vi "Process.vi"(8 "error in":errorcluster, 11 "Lockin.UI":refnum<class "Instrument UI.Lockin.lvclass">) -> (0 "error out":errorcluster, 3 "Lockin.UI out":refnum<class "Instrument UI.Lockin.lvclass">)   [LabVIEW 2019, in "Instrument.Lockin.lvlib" / "Instrument UI.Lockin.lvclass"]
doc: "---------------------------------------------------------------\nJKI State Machine Objects™\nhttp://jki.net/state-machine-objects/\nCopyright (C) 2005-2015, JKI <info@jki.net>\nALL RIGHTS RESERVEDJKI State Machine Objects (SMO) 1.0.0.5\nJKI - JKI\nCopyright (c) 2016, JKI"
uses:
  Instrument UI.Lockin.lvclass
  Instrument.DAQ/Typedefs/DAQ.Calibration--Cluster--Array.ctl
  Instrument.DAQ/Typedefs/DAQ.Calibration--Cluster.ctl
  Instrument.DAQ/Typedefs/Sweep.Channel--Cluster--Array.ctl
  Instrument.DAQ/Typedefs/Sweep.Channel--Cluster.ctl
  Instrument.DAQ/Typedefs/Sweep.Pattern--Enum.ctl
  Instrument.DAQ/Typedefs/Channel.Gain--Cluster--Array.ctl
  Instrument.DAQ/Typedefs/Channel.Gain--Cluster.ctl
  Instrument.Lockin/Typedefs/Results Type--Enum.ctl
  Instrument.DAQ/Typedefs/DAQ.Configuration--Cluster--Array.ctl
  Instrument.DAQ/Typedefs/DAQ.Configuration--Cluster.ctl
  Instrument.DAQ/Typedefs/DAQ.Config.AO.Range--enum.ctl
  Instrument.DAQ/Typedefs/DAQ.TerminalConfiguration--ring.ctl
  Instrument.DAQ/Typedefs/DAQ.Config.AI.Range--enum.ctl
  Instrument.DAQ/Typedefs/DAQ.Config.AI.Coupling--enum.ctl
  Instrument.DAQ/Typedefs/Simulation Mode--enum.ctl
  Instrument.DAQ/Typedefs/DAQ.Sampling.Fs Mode--enum.ctl
  Instrument.DAQ/Typedefs/AO.Channel--Cluster--Array.ctl
  Instrument.DAQ/Typedefs/AO.Channel--Cluster.ctl
  Instrument.DAQ/Typedefs/AO.Channel.Function--Enum.ctl
  Instrument.DAQ/Typedefs/AI.Channel--Cluster--Array.ctl
  Instrument.DAQ/Typedefs/AI.Channel--Cluster.ctl
  Instrument.DAQ/Typedefs/REF.Channel--Cluster--Array.ctl
  Instrument.DAQ/Typedefs/REF.Channel--Cluster.ctl
  Typedefs/Display-Enum.ctl
  C:/Program Files/National Instruments/LabVIEW 2019/vi.lib/JKI/JKI SMO/SMO/SMO.lvclass
  C:/Program Files/National Instruments/LabVIEW 2019/user.lib/LevyLab/Instrument Framework/Instrument UI/Instrument UI.lvclass
  C:/Program Files/National Instruments/LabVIEW 2019/vi.lib/JKI/JKI SMO/SMO.UI/SMO.UI.lvclass
  Instrument.DAQ/Typedefs/DAQ.Sampling.Sample Mode--Ring.ctl
  Instrument.DAQ/Typedefs/State--enum.ctl
  Instrument.Lockin/Typedefs/API/Lockin.setSweep_Table--cluster.ctl
  Instrument.Lockin/Typedefs/Offset Mode--Enum.ctl
  Instrument.DAQ/Typedefs/PrivateEvents--DAQ.setCalibration.ctl
  Instrument.DAQ/Typedefs/Status--enum.ctl
  <userlib>/LevyLab/Instrument Framework/Instrument UI/Instrument UI.lvclass/Instrument UI.ctl
  Instrument.Lockin/Instrument.Lockin.lvclass
  C:/Program Files/National Instruments/LabVIEW 2019/user.lib/LevyLab/Instrument Framework/Instrument/Instrument.lvclass
  Typedefs/UI.Configuration--Cluster.ctl
  Instrument.DAQ/Typedefs/Configuration.Channels--Cluster.ctl
  Instrument.DAQ/Typedefs/DAQ.Sampling--Cluster.ctl
  Instrument.DAQ/Typedefs/DAQ.Sampling.Sampling--Cluster.ctl
  Instrument.DAQ/Typedefs/Configuration.Prefilter--Cluster.ctl
  Instrument.DAQ/Typedefs/Channel.GainsAndOffsets--Cluster.ctl
  Instrument.DAQ/Typedefs/Configuration.AmplitudeLimit--Cluster.ctl
  Instrument.DAQ/Typedefs/Configuration.DCLimit--Cluster.ctl
  Instrument.DAQ/Typedefs/Configuration.LinkFrequencies--Cluster.ctl
  Instrument.DAQ/Typedefs/Sweep.Configuration--Cluster.ctl
  Instrument.DAQ/Typedefs/Configuration.DutyCycle--Cluster.ctl
  Instrument.Lockin/Typedefs/Lockin.getAllData--Cluster.ctl
  Instrument.DAQ/Typedefs/PublicEvents--DAQ.getWaveforms.ctl
  Instrument.DAQ/Typedefs/Results--Cluster.ctl
  Instrument.DAQ/Typedefs/PublicEvents--DAQ.getSweepWaveforms.ctl
  <userlib>/LevyLab/Configuration/Configuration.lvclass
  Typedefs/UI.References--Cluster.ctl
  Typedefs/UI.References.Booleans--Cluster.ctl
  Typedefs/UI.References.Clusters--Cluster.ctl
  Typedefs/UI.References.Graphs--Cluster.ctl
  <userlib>/LevyLab/Configuration/Configuration.lvclass/Configuration.ctl
  <vilib>/JKI/JKI SMO/SMO/SMO.lvclass/SMO.ctl
  <vilib>/JKI/JKI SMO/SMO.UI/SMO.UI.lvclass/SMO.UI.ctl
  Instrument.Lockin/Typedefs/API/Lockin.setState--cluster.ctl
  Instrument.Lockin/Typedefs/API/Lockin.Commands--Enum.ctl
  Instrument.Lockin/Typedefs/API/Lockin.Commands.Local--Enum.ctl
  Instrument.DAQ/Typedefs/PrivateEvents--DAQ.showUI.ctl
  Instrument.Lockin/Typedefs/API/Lockin.setLogMode--cluster.ctl
  Instrument.Lockin/Typedefs/API/Lockin.setSamplingMode--cluster.ctl
  Instrument.Lockin/Typedefs/API/Lockin.setSamplingFsMode--cluster.ctl
  fb76c5f8-a1bb-4bb3-bb88-03f40c6ef356.vi
  76a2c689-62cf-4547-b40d-909294413a54.vi
  ea889f97-4432-4e18-8daa-f8276c71e6b3.vi
  e313e854-8cc0-44b2-b8a5-b0d9dd449797.vi
  f60e4b8a-05f4-439c-aeb3-da82266228cf.vi
  5a499ed1-b987-4b60-a17a-49cbc4aa87e6.vi
  11ce9ad4-6d29-4ca4-b8bb-b11228104e6f.vi
  a8738246-2ac0-499e-83b1-af72f8904bf5.vi
  <vilib>/JKI/JKI SMO/SMO/Private/ReftoDVR--SMO.vi
  <vilib>/JKI/JKI SMO/SMO.UI/SMO.UI.ReftoDVR.vi
  11ce9ad4-6d29-4ca4-b8bb-b11228104e6f.vi/189031a7-82a1-4f0a-9ed5-d68f3439fd4c.vi
  11ce9ad4-6d29-4ca4-b8bb-b11228104e6f.vi/de7eedf1-e1e8-4423-8aaa-e1093bc59ae0.vi
  <userlib>/LevyLab/Debug/Debug/Get Debug Mode.vi
  <vilib>/Platform/browser.llb/Open URL in Default Browser (string).vi
  private/Set Plot Visibility (WDTWFGraph).vi
  <vilib>/measure/matone.llb/Extract Single Tone Information 1 Chan.vi
  private/Set Plot Color (WFChart2D).vi
  private/Set Legend (WDTWFGraph).vi
  <vilib>/Waveform/WDTOps.llb/WDT Waveform Duration DBL.vi
  <vilib>/Utility/Data Type/Get Type Information.vi
  <vilib>/Utility/Data Type/Get Numeric Information.vi
  <userlib>/_OpenG.lib/lvdata/lvdata.llb/Unwrap VVariant__ogtk.vi
  <vilib>/JDP Science/JSONtext/Variant to JSON Text.vi
  <userlib>/LevyLab/Instrument Framework/Instrument/API/Instrument.sendMessageToProcess (string).vi
  <vilib>/JKI/JKI SMO/SMO/SMO.lvclass
  <userlib>/LevyLab/Instrument Framework/Instrument/Instrument.lvclass
  <vilib>/JDP Science/JSONtext/LVClass Serializer/JSONtext LVClass Serializer.lvclass
  <userlib>/LevyLab/Instrument Framework/Instrument UI/Instrument UI.lvclass
  Instrument.DAQ/Instrument.DAQ.lvclass
  <vilib>/measure/NI_MAPro.lvlib
  <vilib>/JKI/JKI SMO/SMO.UI/SMO.UI.lvclass
  Lockin.Utilities/Lockin.Utilities.lvlib
  <userlib>/LevyLab/Debug/Debug.lvlib
  C:/Program Files/National Instruments/LabVIEW 2019/user.lib/LevyLab/Instrument Framework/Instrument Types/Lockin/Instrument.LockinAPI.lvclass
  private/Set All Plot Visibility (WFGraph).vi
  private/Set All Plot Visibility (XYGraph).vi
  private/Get Plot Visibility (WFGraph).vi
  private/Set Plot Visibility (WFGraph).vi
  private/Set Plot Visibility (XYGraph).vi
  private/Set Legend (WFGraph).vi
  private/Set Plot Color (WDTWFGraph).vi
  private/Set Plot Color (WFGraph).vi
  private/Set Legend (XYGraph).vi
  private/Set Plot Color (XYGraph).vi
  <vilib>/measure/maspectr.llb/FFT Power Spectrum and PSD for N Chan.vi
panel:
  out "Version":string="vDevelopment" caption="V"
  in  "Fs Multiplier":dbl=5000.0 format="%#_13g"
  in  "Refresh Rate (Hz)":dbl=10.0 format="%#_13g"
  in  "Decimate":enum16{"1", "10", "100", "1000"}(ring) caption="Enum 3"
  in  "Decimation (pre DSP)":i32=1
  in  "Decimation (post DSP)":i32=1
  in  "....................State....................":bool
  in  "....................Graph and UI....................":bool
  in  "....................DAQ and Channel....................":bool
  in  "....................Dynamic Events....................":bool
  in  "Left Tab":T1(tab)=enum."DAQ Settings"
  in  "f link (Hz)":dbl=13.0 format="%#_6p"
  in  "Link f?":bool
  in  "DC Limit All":bool
  in  "DC Limit None":bool
  in  "AC Limit All":bool
  in  "AC Limit None":bool
  out "-3dB BW (Hz)":dbl=50.0
  out "Noise BW (Hz)":dbl=50.0
  out "Settling Time (s)":dbl=50.0
  in  "REF Channels":T2 {"Roll-Off" min=1 max=4; "TC" min=1e-06 max=100.0 format="%#_3p"; "Phase" format="%#_3p"; "Frequency" min=1e-06 max=102400.0 format="%#_6p"; "Channel" min=1}
  in  "AO DC Limit":dbl=0.009999999 caption="DC limit" format="%#_6p"
  in  "AC Limit":dbl=0.009999999 caption="AC limit" format="%#_6p"
  in  "duty cycle (%)":dbl=50.0
  in  "Disable All":bool
  in  "Enable All":bool
  in  "AI Channels":T4 {"reference index" min=1; "References" items=["", "1", "2", "3", "4", "5", "6", "7", "8", "9"]; "Channel" min=1}
  in  "AO Channels":T6 {"Phase" format="%#_3g"; "Frequency" min=0.0001 max=200000.0 format="%#_6p"; "Offset" format="%#_6p"; "Amplitude" min=0.0 max=10.0 format="%#_6p"}
  out "Fs Output (S/s)":dbl=100.0
  in  "Remove Offset":bool
  in  "Measure Offset":bool
  in  "Fs (S/s) (buffer)":dbl=204800.0 format="%#_13g"
  in  "#s (S) (buffer)":i32=20480
  in  "Show DAQ UI":bool
  out "Actual Fs (S/s)":dbl=10.0 format="%#_13g"
  out "Actual #s (S)":i32=10
  in  "DAQ Config":T9 {"AI terminal config" items=[""=-1, "differential"=10106, "pseudodifferential"=12529]; "AI.Coupling" items=[""=0, "AC"=10045, "DC"=10050, "GND"=10066]; "AO terminal config" items=[""=-1, "differential"=10106, "pseudodifferential"=12529]}
  in  "Auto DAQ":bool caption="Auto Configure"
  in  "Fs Mode":T15
  in  "Logging":bool
  in  "AI Simulation mode":T16=enum."AI = noise*AO"
  in  "Reset Phase":bool
  in  "LP f (Hz)":dbl=100.0 format="%.3p"
  in  "Line":bool
  in  "Lowpass":bool
  in  "PLL AI Channel":i32=1 caption="AI Channel"
  in  "Enable PLL":bool caption="Enable"
  in  "Input Gain":T17
  in  "Output Gain":T17
  in  "Input Offsets":T17 {"Gain" format="%#_3p"}
  in  "Route Signal Type":T19 caption="Signal Type"
  in  "Route Ref Channel":i32=1 caption="Ref Channel"
  in  "Route AI Channel":i32=1 caption="AI Channel"
  out "Route Output (V)":dbl caption="Output (V)"
  in  "Route AO Channel":i32=1 caption="AO Channel" min=1
  in  "Enable Route":bool caption="Enable"
  in  "Sweep Pattern":cluster{"Channel":u16, "Sweep Pattern":dbl[]}[](array[cluster])=[{"Channel"=0, "Sweep Pattern"=[]}] {"Sweep Pattern" format="%#_3p"; "Channel" min=1 max=128}
  in  "Sweep Channels":T20=[{"Enable?"=FALSE, "Channel"=0, "Start"=0.0, "End"=0.1, "Pattern"=enum."Table", "Table"=[]}] {"Table" format="%#_1f"; "Channel" min=1 max=128; "Start" format="%#_6p"; "End" format="%#_6p"}
  in  "Sweep Time (s)":dbl=20.0
  in  "Initial Wait (s)":dbl=1.0
  out "Sweep Timer (s)":dbl caption="Timer (s)"
  in  "Return to Start?":bool
  out "System Serial Number":string caption="SMO State"
  out "Application Version":string caption="SMO State"
  out "Status":string
  out "Sampling Status":u32(colorbox)
  out "State Queue":string
  out "Sampling Status":string="Good"
  out "State History":string
  out "Wfm Refresh Time (ms)":u32=103
  out "Inst.DAQ State":string caption="SMO State"
  out "UI Refresh Time (ms)":u32=103
  out "Sweep Time":dbl format="%<%I:%M:%S %p %m/%d/%Y>T"
  out "State Time":dbl format="%<%I:%M:%S %p %m/%d/%Y>T"
  out "Cal Info":T23 {"DevTemp" format="%.1f"; "SelfCal.LastTemp" format="%.1f"; "SelfCal.LastDate/Time" format="%<%I:%M %p %m/%d/%Y>T"}
  in  "Get Calibration":bool
  in  "Self Calibrate":bool
  in  "Tab Control 3":enum32{"Page 1"}(tab)
  out "mean (V)":dbl format="%_3p"
  out "X (V)":dbl format="%_3p"
  out "Y (V)":dbl format="%_3p"
  in  "channel-reference":u16(ring) items=["AI1 REF 1"]
  out "R (V)":dbl format="%_3p"
  out "theta (°)":dbl format="%_3p"
  in  "Close":bool
  out "String":string
  in  "Pause":bool
  in  "Reset":bool
  in  "Start":bool
  in  "Help":bool
  in  "Start Sweep":bool
  in  "Stop Sweep":bool
  in  "Right Tab":T25(tab)
  in  "Sync?":bool
  in  "Sync Ch":i32=1
  out "f (Hz)":string
  out "phi (°)":string
  in  "Output":enum16{"AO", "REF"}(ring) caption="Enum 3"
  in  "Input":enum16{"Device", "ADC"}(ring) caption="Enum 3"
  out "REF Graph":waveform(dbl)[](graph)
  in  "AO Graph All":bool
  in  "AO Graph None":bool
  in  "AI Graph All":bool
  in  "AI Graph None":bool
  out "AI Graph":waveform(dbl)[](graph)
  in  "X Scale":enum16{"time", "samples"}(ring) caption="Enum 3"
  out "AO Graph":waveform(dbl)[](graph)
  in  "REF Graph None":bool
  in  "REF Graph All":bool
  out "Lockin 1":waveform(dbl)[](graph)
  in  "Display 2":T26 caption="Enum 3"
  in  "Y/Theta Range":dbl caption="Range" format="%#_6p"
  in  "Display 1":T26 caption="Enum 3"
  in  "X/R Range":dbl caption="Range" format="%#_6p"
  out "Lockin 2":waveform(dbl)[](graph)
  in  "Lockin Graph All":bool
  in  "Lockin Graph None":bool
  out "Results":string[][](table)
  out "Lockin XY":cluster{dbl[], dbl[]}[](graph)
  in  "XY Range":dbl caption="Range" format="%#_6p"
  in  "Lockin Graph None 2":bool
  in  "Lockin Graph All 2":bool
  out "Sweep AI":waveform(dbl)[](graph)
  out "Sweep AO":waveform(dbl)[](graph)
  out "Sweep Y":waveform(dbl)[](graph)
  out "Sweep X":waveform(dbl)[](graph)
  in  "chart?":bool=TRUE
  in  "chart all?":bool=TRUE
  in  "PS Display":enum16{"AO", "AI", "X", "Y", "R", "Theta"}(ring) caption="Enum 3"
  in  "# averages":u32=10 min=1
  in  "weighting mode":enum16{"Linear", "Exponential"}(ring)=enum."Exponential"
  in  "averaging mode":T27(ring)=enum."RMS averaging"
  in  "window":u32(ring)=1 items=["Rectangle"=0, "Hanning"=1, "Hamming"=2, "Blackman-Harris"=3, "Exact Blackman"=4, "Blackman"=5, "Flat Top"=6, "4 Term B-Harris "=7, "7 Term B-Harris"=8, "Low Sidelobe"=9, "Blackman Nuttall"=11, "Triangle"=30, "Bartlett-Hanning"=31, "Bohman"=32, "Parzen"=33, "Welch"=34, "Kaiser"=60, "Dolph-Chebyshev"=61, "Gaussian"=62]
  in  "export mode":u16(ring)=1 items=["Power Spectrum", "Power Spectral Density"]
  in  "restart":bool
  out "done?":bool=TRUE
  out "PS Waveform":cluster{"f0":dbl, "df":dbl, "magnitude":dbl[]}[](graph)
  out "averages":dbl=180.0
  out "PS Chart":dbl[][](graph)
  # "Lockin UI"
  # "For instructions on how to use the JKI State Machine Objects, examples and video tutorials, visit:\nhttp://jki.net/state-machine-objects/\n\nJKI State Machine Objects™\nhttp://jki.net/state-machine-objects/\nCopyright (C) 2005-2015, JKI <info@jki.net>\nALL RIGHTS RESERVED"
  # "- Choose an input lockin channel and value (X,Y, etc) and it will be written as a DC value to an output channel of your choosing.\n- Output is scaled by the input amplifier gain."
  # "Output"
  # "Input"
  # ">> DEVICE >>"
  # "(*)"
  # "ch"
  # "AC (V)"
  # "DC (V)"
  # "f (Hz)"
  # "phase (°)"
  # "function"
  # "sweep"
  # "(*)"
  # "ch"
  # "1     2    3"
  # "References"
  # "Offset"
  # "Output Settings"
  # "Reference"
  # "Reference Filter"
  # "ch"
  # "f (Hz)"
  # "phase (°)"
  # "TC (s)"
  # "order (n)"
  # "DAQ Channels"
  # "Device"
  # "AO"
  # "AI"
  # "terminals"
  # "ch"
  # "ch"
  # "range"
  # "range"
  # "coupling"
  # "terminals"
  # "Sampling"
  # "Pre-Filters"
  # "Simulation"
  # "Push \"Reset Acquisiton\" below when you want to apply new settings"
  # "not used during process-ing"
  # "DAQ"
  # "Logging"
  # "Output Gain"
  # "Input Offset / Gain"
  # "Route Lockin Input to Output"
  # "PLL"
  # "experimental ca 11/18/2025"
  # "experimental ca 11/18/2025"
  # "ch"
  # "Input gain"
  # "ch"
  # "Output gain"
  # "ch"
  # "Input offset"
  # "Sweep"
  # "pattern"
  # "(*)"
  # "ch"
  # "start"
  # "end"
  # "ch"
  # "table"
  # "Status"
  # "Calibration"
  # "Most Recent Self-Calibration"
  # "device"
  # "time"
  # "T (°C)"
  # "T (°C)"
  # "OK?"
  # "DAQ"
  # "Sweep"
  # "Application"
  # "Status"
  # "Input Graphs"
  # "Output Graphs"
  # "Lockin Results: Graph 1"
  # "Lockin Results: Graph 2"
  # "Lockin Results: Table"
  # "Lockin Results: Phasor Graph"
  # "Sweep AI"
  # "Sweep AO"
  # "Sweep Results"
  # "Sweep Results"
  # "Power Spectra"
  # "db( ):\ndB(V) for volts\ndB(A) for amps\ndB(°) for degrees"
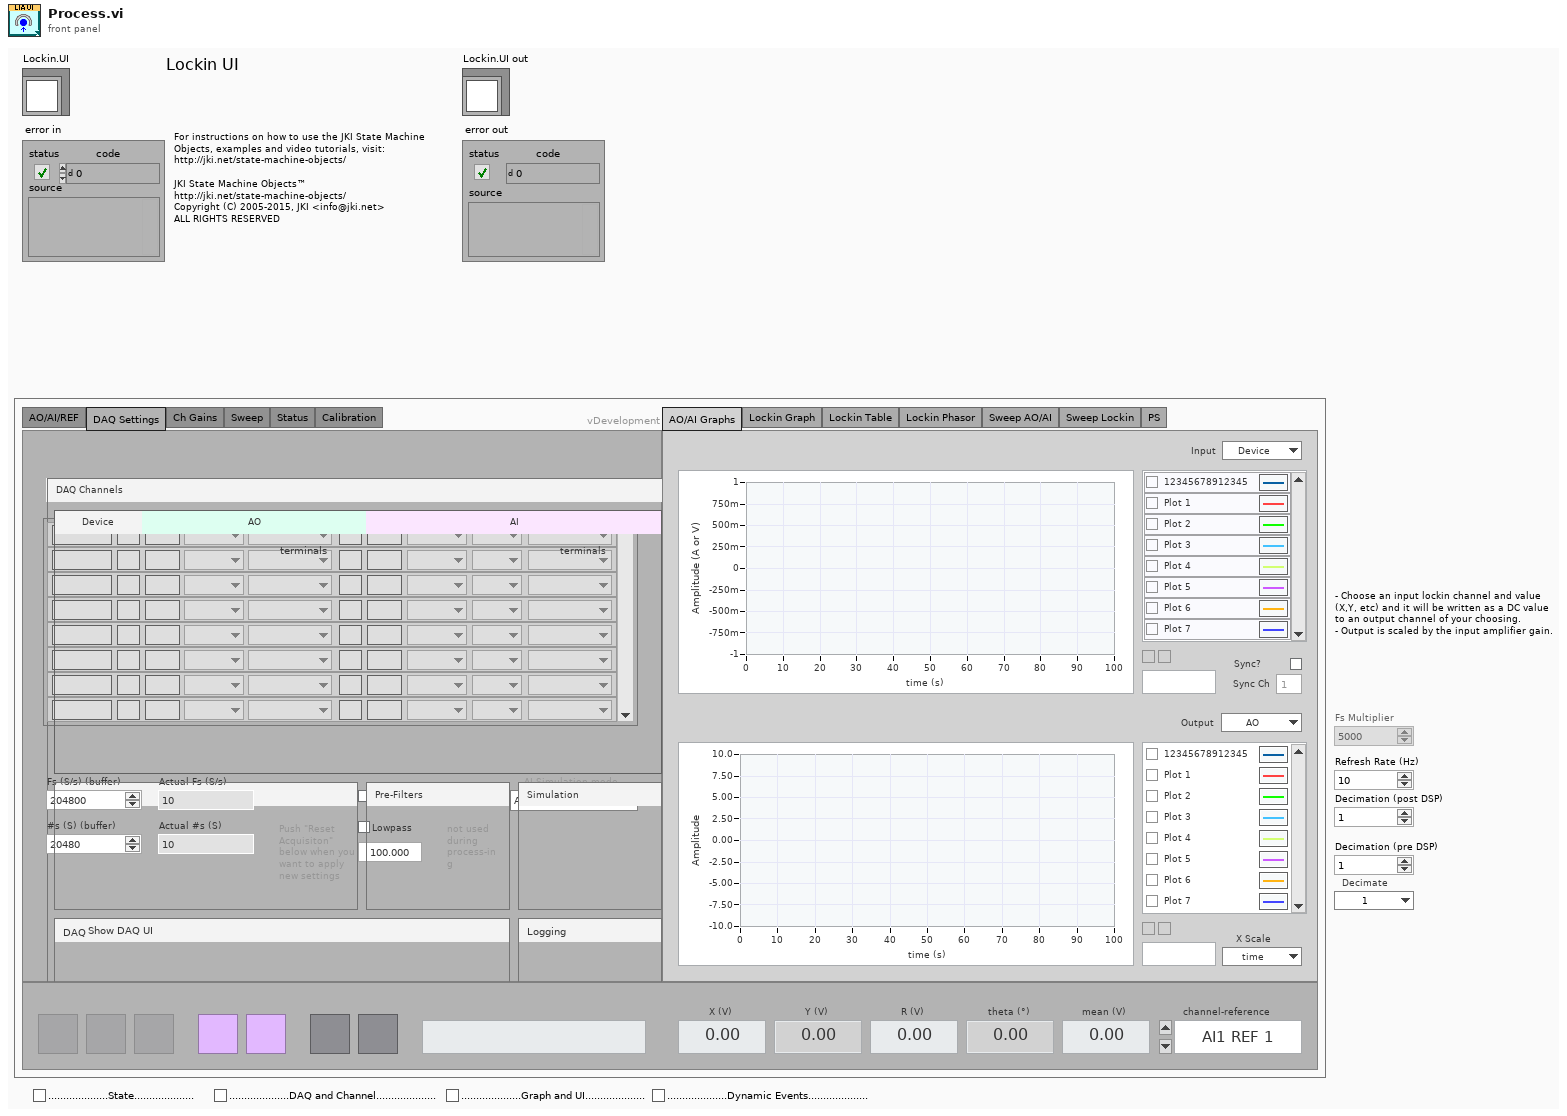
[diagram p1: front panel]
types:
  T1 = enum32{"AO/AI/REF", "DAQ Settings", "Ch Gains", "Sweep", "Status", "Calibration"}
  T2 = typedef "Instrument.Lockin.lvlib/Instrument.DAQ.lvclass/REF.Channel--Cluster--Array.ctl" = T3[]
  T3 = typedef "Instrument.Lockin.lvlib/Instrument.DAQ.lvclass/REF.Channel--Cluster.ctl" = cluster{"Enable?":bool, "Channel":i32, "Frequency":dbl, "Phase":dbl, "TC":dbl, "Roll-Off":i32}
  T4 = typedef "Instrument.Lockin.lvlib/Instrument.DAQ.lvclass/AI.Channel--Cluster--Array.ctl" = T5[]
  T5 = typedef "Instrument.Lockin.lvlib/Instrument.DAQ.lvclass/AI.Channel--Cluster.ctl" = cluster{"Enable?":bool, "Channel":i32, "References":u16[], "reference index":i32}
  T6 = typedef "Instrument.Lockin.lvlib/Instrument.DAQ.lvclass/AO.Channel--Cluster--Array.ctl" = T7[]
  T7 = typedef "Instrument.Lockin.lvlib/Instrument.DAQ.lvclass/AO.Channel--Cluster.ctl" = cluster{"Enable?":bool, "Channel":i32, "Amplitude":dbl, "Offset":dbl, "Frequency":dbl, "Phase":dbl, "Function":T8, "Sweeping?":bool, "Limit AC":bool, "Limit DC?":bool, "Duty Cycle":bool}
  T8 = typedef "Instrument.Lockin.lvlib/Instrument.DAQ.lvclass/AO.Channel.Function--Enum.ctl" = enum16{"sine", "square", "triangle", "saw"}
  T9 = typedef "Instrument.Lockin.lvlib/Instrument.DAQ.lvclass/DAQ.Configuration--Cluster--Array.ctl" = T10[]
  T10 = typedef "Instrument.Lockin.lvlib/Instrument.DAQ.lvclass/DAQ.Configuration--Cluster.ctl" = cluster{"Device":string, "Lockin.AO":string, "AO.Ch":string, "AO.Range":T11, "AO terminal config":T12, "Lockin.AI":string, "AI.Ch":string, "AI.Range":T13, "AI.Coupling":T14, "AI terminal config":T12}
  T11 = typedef "Instrument.Lockin.lvlib/Instrument.DAQ.lvclass/DAQ.Config.AO.Range--enum.ctl" = enum16{"±0.1", "±1.0", "±3.5", "±10.0", ""}
  T12 = typedef "Instrument.Lockin.lvlib/Instrument.DAQ.lvclass/DAQ.TerminalConfiguration--ring.ctl" = i32
  T13 = typedef "Instrument.Lockin.lvlib/Instrument.DAQ.lvclass/DAQ.Config.AI.Range--enum.ctl" = enum16{"±0.316", "±1.00", "±3.16", "±10.0", "±31.6", "±42.4", ""}
  T14 = typedef "Instrument.Lockin.lvlib/Instrument.DAQ.lvclass/DAQ.Config.AI.Coupling--enum.ctl" = u16
  T15 = typedef "Instrument.Lockin.lvlib/Instrument.DAQ.lvclass/DAQ.Sampling.Fs Mode--enum.ctl" = enum16{"Manual", "Auto Fs", "Max Fs"}
  T16 = typedef "Instrument.Lockin.lvlib/Instrument.DAQ.lvclass/Simulation Mode--enum.ctl" = enum16{"AI = HW simulated", "AI = noise*AO", "AI = waveguide"}
  T17 = typedef "Instrument.Lockin.lvlib/Instrument.DAQ.lvclass/Channel.Gain--Cluster--Array.ctl" = T18[]
  T18 = typedef "Instrument.Lockin.lvlib/Instrument.DAQ.lvclass/Channel.Gain--Cluster.ctl" = cluster{"Channel":string, "Gain":dbl}
  T19 = typedef "Instrument.Lockin.lvlib/Instrument.Lockin.lvclass/Results Type--Enum.ctl" = enum16{"X", "Y", "R", "Theta", "Mean"}
  T20 = typedef "Instrument.Lockin.lvlib/Instrument.DAQ.lvclass/Sweep.Channel--Cluster--Array.ctl" = T21[]
  T21 = typedef "Instrument.Lockin.lvlib/Instrument.DAQ.lvclass/Sweep.Channel--Cluster.ctl" = cluster{"Enable?":bool, "Channel":u16, "Start":dbl, "End":dbl, "Pattern":T22, "Table":dbl[]}
  T22 = typedef "Instrument.Lockin.lvlib/Instrument.DAQ.lvclass/Sweep.Pattern--Enum.ctl" = enum16{"Ramp /", "Ramp /\\", "Smooth Ramp _/", "Smooth Ramp _/\\_", "Table"}
  T23 = typedef "Instrument.Lockin.lvlib/Instrument.DAQ.lvclass/DAQ.Calibration--Cluster--Array.ctl" = T24[]
  T24 = typedef "Instrument.Lockin.lvlib/Instrument.DAQ.lvclass/DAQ.Calibration--Cluster.ctl" = cluster{"Active Device":string, "SelfCal.LastDate/Time":dbl, "SelfCal.LastTemp":dbl, "DevTemp":dbl, "calibration due?":bool}
  T25 = enum32{"AO/AI Graphs", "Lockin Graph", "Lockin Table", "Lockin Phasor", "Sweep AO/AI", "Sweep Lockin", "PS"}
  T26 = typedef "Instrument.Lockin.lvlib/Instrument UI.Lockin.lvclass/Display-Enum.ctl" = enum16{"X", "Y", "R", "Theta", "Mean"}
  T27 = enum16{"No averaging", "Vector averaging", "RMS averaging", "Peak hold"}
  T28 = enum16{"Spinner 1", "Spinner 2", "Spinner 3", "Spinner 4", "Spinner 5", "Spinner 6"}
  T29 = typedef "Instrument.Lockin.lvlib/Instrument.DAQ.lvclass/State--enum.ctl" = enum16{"start", "stop", "reset", "start sweep", "stop sweep"}
  T30 = typedef "Instrument.Lockin.lvlib/Instrument.Lockin.lvclass/Lockin.setSweep_Table--cluster.ctl" = cluster{"Channel":i32, "Table":dbl[]}
  T31 = typedef "Instrument.Lockin.lvlib/Instrument.Lockin.lvclass/Offset Mode--Enum.ctl" = enum16{"Measure", "Remove"}
  T32 = typedef "Instrument.Lockin.lvlib/Instrument.DAQ.lvclass/PrivateEvents--DAQ.setCalibration.ctl" = enum16{"Check", "Calibrate"}
  T33 = typedef "Instrument.Lockin.lvlib/Instrument.DAQ.lvclass/Status--enum.ctl" = enum16{"idle", "created", "started", "stopped", "sweeping"}
  T34 = enum32{"invalid app kind", "Development System", "Run Time System", "Student Edition", "Embedded LabVIEW", "Evaluation", "Custom"}
  T35 = enum32{"Invalid", "Standard", "Closed", "Hidden", "Minimized", "Maximized"}
  T36 = enum8{"Enabled", "Disabled", "Disabled and Grayed Out"}
  T37 = typedef "Instrument.Lockin.lvlib/Instrument.Lockin.lvclass/Lockin.setState--cluster.ctl" = cluster{"State":T29}
  T38 = typedef "Instrument.Lockin.lvlib/Instrument.Lockin.lvclass/Lockin.Commands--Enum.ctl" = enum16{"setAO", "setAO_Amplitude", "setAO_DC", "setAO_Frequency", "setAO_Phase", "setAO_Function", "setREF", "setREF_Frequency", "setREF_Phase", "setREF_TC", "setREF_Roll-Off", "setDAQ", "setSampling", "setState", "getState", "getAO", "getAI", "getResults", "getSampling", "getAOconfig", "getREFconfig", "setInputGain", "setOutputGain", "getInputGain", "getOutputGain", "setSamplingFsMode", "getSamplingFsMode", "setSweep", "setSweep_Time", "setSweep_Table", "getStatus", "getSweepResults", "getSweepWaveforms", "logConfiguration", "startLogging", "stopLogging"}
  T39 = typedef "Instrument.Lockin.lvlib/Instrument.Lockin.lvclass/Lockin.Commands.Local--Enum.ctl" = enum16{"autoConfigureDAQ", "setSimulationMode", "zeroPhase", "setCalibration", "setPreFilter", "setFrequencyLink", "setAmplitudeLimit", "setDCLimit", "setDutyCycle", "setSamplingDecimationPreDSP", "setSamplingDecimationPostDSP", "setSamplingMode", "setSamplingFsMultiplier", "setSamplingFsOutput", "setSamplingRefreshRate", "setData_State", "setData_DAQ", "setData_Sampling", "setData_Waveforms", "setData_Results", "setData_SweepWaveforms", "setData_AIChannels", "setData_AOChannels", "setData_REFChannels", "setData_InputGain", "setData_OutputGain", "showUI", "setAI", "setOffset", "setOffsetMode"}
  T40 = typedef "Instrument.Lockin.lvlib/Instrument.DAQ.lvclass/PrivateEvents--DAQ.showUI.ctl" = bool
  T41 = typedef "Instrument.Lockin.lvlib/Instrument.Lockin.lvclass/Lockin.setLogMode--cluster.ctl" = cluster{"interval":u32}
  T42 = typedef "Instrument.Lockin.lvlib/Instrument.Lockin.lvclass/Lockin.setSamplingMode--cluster.ctl" = cluster{"SampleMode":T43}
  T43 = typedef "Instrument.Lockin.lvlib/Instrument.DAQ.lvclass/DAQ.Sampling.Sample Mode--Ring.ctl" = i32
  T44 = typedef "Instrument.Lockin.lvlib/Instrument.Lockin.lvclass/Lockin.setSamplingFsMode--cluster.ctl" = cluster{"FsMode":T15}
  T45 = cluster{"averaging mode":enum16{"No averaging", "Vector averaging", "RMS averaging", "Peak hold"}, "weighting mode":enum16{"Linear", "Exponential"}, "number of averages":u32}
  T46 = typedef "Instrument.Lockin.lvlib/Instrument UI.Lockin.lvclass/UI.Configuration--Cluster.ctl" = cluster{"Channels":T47, "DAQ":cluster{"Configuration":T9, "cfg.Sampling":T48, "Calibration":T23, "Simulation mode":T16}, "PreFilter":T50, "Amplifers":T51, "Limit Amplitude":T52, "Limit DC":T53, "Link Frequencies":T54, "Sweep":T55, "Plot":cluster{"visibility.AI":bool[], "visibility.AO":bool[], "visibility.Lockin":bool[], "Display 1":T26, "Display 2":T26}, "Function Option":T56}
  T47 = typedef "Instrument.Lockin.lvlib/Instrument.DAQ.lvclass/Configuration.Channels--Cluster.ctl" = cluster{"Cfg_AO":T6, "Cfg_AI":T4, "Cfg_REF":T2}
  T48 = typedef "Instrument.Lockin.lvlib/Instrument.DAQ.lvclass/DAQ.Sampling--Cluster.ctl" = cluster{"Sampling":T49, "sample mode":i32, "Fs Mode":T15, "Fs Multiplier":dbl, "Refresh Rate (Hz)":dbl, "Decimation.PreDSP":i32, "Decimation.PostDSP":i32, "Fs.Output":dbl}
  T49 = typedef "Instrument.Lockin.lvlib/Instrument.DAQ.lvclass/DAQ.Sampling.Sampling--Cluster.ctl" = cluster{"Fs":dbl, "#s":i32}
  T50 = typedef "Instrument.Lockin.lvlib/Instrument.DAQ.lvclass/Configuration.Prefilter--Cluster.ctl" = cluster{"60 Hz":bool, "Low Pass":bool, "Low Pass Cutoff (Hz)":dbl}
  T51 = typedef "Instrument.Lockin.lvlib/Instrument.DAQ.lvclass/Channel.GainsAndOffsets--Cluster.ctl" = cluster{"Offset_AI":T17, "Gain_AI":T17, "Gain_AO":T17}
  T52 = typedef "Instrument.Lockin.lvlib/Instrument.DAQ.lvclass/Configuration.AmplitudeLimit--Cluster.ctl" = cluster{"Limit (V)":dbl}
  T53 = typedef "Instrument.Lockin.lvlib/Instrument.DAQ.lvclass/Configuration.DCLimit--Cluster.ctl" = cluster{"Limit (V)":dbl}
  T54 = typedef "Instrument.Lockin.lvlib/Instrument.DAQ.lvclass/Configuration.LinkFrequencies--Cluster.ctl" = cluster{"Link?":bool, "Frequency (Hz)":dbl}
  T55 = typedef "Instrument.Lockin.lvlib/Instrument.DAQ.lvclass/Sweep.Configuration--Cluster.ctl" = cluster{"sweepTime":dbl, "initialWaitTime":dbl, "returnToStart":bool, "sweepChannels":T20}
  T56 = typedef "Instrument.Lockin.lvlib/Instrument.DAQ.lvclass/Configuration.DutyCycle--Cluster.ctl" = cluster{"Option?":bool, "Duty Cycle (%)":dbl}
  T57 = typedef "Instrument.Lockin.lvlib/Instrument.Lockin.lvclass/Lockin.getAllData--Cluster.ctl" = cluster{"DAQ State":T33, "Waveforms":T58, "Results":T59, "SweepWaveforms":T60}
  T58 = typedef "Instrument.Lockin.lvlib/Instrument.DAQ.lvclass/PublicEvents--DAQ.getWaveforms.ctl" = cluster{"AO":waveform(dbl)[], "AI":waveform(dbl)[], "REF_X":waveform(dbl)[], "REF_Y":waveform(dbl)[], "X":waveform(dbl)[], "Y":waveform(dbl)[]}
  T59 = typedef "Instrument.Lockin.lvlib/Instrument.DAQ.lvclass/Results--Cluster.ctl" = cluster{"Time Stamp":timestamp, "Results (Dictionary)":cluster{"key":string, "value":dbl[]}[]}
  T60 = typedef "Instrument.Lockin.lvlib/Instrument.DAQ.lvclass/PublicEvents--DAQ.getSweepWaveforms.ctl" = cluster{"AO":waveform(dbl)[], "AI":waveform(dbl)[], "X":waveform(dbl)[], "Y":waveform(dbl)[]}
  T61 = typedef "Instrument.Lockin.lvlib/Instrument UI.Lockin.lvclass/UI.References--Cluster.ctl" = cluster{"Booleans":T62, "Clusters":T63, "Graphs":T64}
  T62 = typedef "Instrument.Lockin.lvlib/Instrument UI.Lockin.lvclass/UI.References.Booleans--Cluster.ctl" = cluster{"Start":refnum<vi>, "Pause":refnum<vi>, "Reset":refnum<vi>, "Trigger":refnum<vi>, "Help":refnum<vi>, "Close":refnum<vi>, "Start Sweep":refnum<vi>, "Stop Sweep":refnum<vi>}
  T63 = typedef "Instrument.Lockin.lvlib/Instrument UI.Lockin.lvclass/UI.References.Clusters--Cluster.ctl" = cluster{"AO Channels":refnum<vi>, "AI Channels":refnum<vi>, "REF Channels":refnum<vi>, "DAQ Config":refnum<vi>, "Sweep Channels":refnum<vi>, "Cal Info":refnum<vi>}
  T64 = typedef "Instrument.Lockin.lvlib/Instrument UI.Lockin.lvclass/UI.References.Graphs--Cluster.ctl" = cluster{"AI Graph":refnum<vi>, "AO Graph":refnum<vi>, "REF Graph":refnum<vi>, "Lockin 1":refnum<vi>, "Lockin 2":refnum<vi>, "Lockin XY":refnum<vi>, "Sweep X Graph":refnum<vi>, "Sweep Y Graph":refnum<vi>, "Sweep AI Graph":refnum<vi>, "Sweep AO Graph":refnum<vi>, "PS WFGraph":refnum<vi>, "PS Chart":refnum<vi>}
  T65 = cluster{"Core":cluster{"Current VI Reference":refnum<vi>, "Close Panel on Exit?":bool, "Last Error":cluster{"error":errorcluster, "previous state":string, "remaining states":string}, "Shutdown?":bool}, "SMO":refnum<class "Instrument UI.Lockin.lvclass">, "Lockin":refnum<class "Instrument.Lockin.lvclass">, "Configuration":refnum<class "Configuration.lvclass">, "UI Config":T46, "DAQ state":T33, "getAll":T57, "Waveform Charts":waveform(dbl)[][], "References":T61, "Message":cluster{"Command":variant, "Data":variant}, "Front Panel":refnum<vi>, "update waveform graphs":bool, "update lockin graphs":bool, "clear lockin charts":bool}
  T66 = cluster{"Enable?":bool, "Channel":bool, "References":bool[], "reference index":bool}[]
  T67 = typedef "SMO.lvclass/SMOState --Enum.ctl" = enum16{"unknown", "Created", "Started", "Stopped"}
  T68 = cluster{"Fs.Output (S/s)":dbl, "Decimation Factor":i32, "Settling Time (s)":dbl, "Noise Bandwidth (Hz)":dbl, "-3dB Bandwidth (Hz)":dbl, "Attenuation (dB)":dbl}
  T69 = cluster{"Current VI Reference":refnum<vi>, "Close Panel on Exit?":bool, "Last Error":cluster{"error":errorcluster, "previous state":string, "remaining states":string}, "Shutdown?":bool}
  T70 = typedef "SMO.lvclass/Protected Events.ctl" = cluster{"StopProcesses":refnum<user-event>, "AbortProcesses":refnum<user-event>, "Config Changed":refnum<user-event>, "Dependency":refnum<user-event>}
  T71 = typedef "Instrument.lvlib/Instrument.lvclass/PublicEvents--Cluster.ctl" = cluster{"MessageFromProcess":refnum<user-event>}
  T72 = typedef "SMO.UI.lvclass/PublicEvents--Cluster.ctl" = cluster{"UI Hidden":refnum<user-event>, "UI State":refnum<user-event>}
  T73 = typedef "SMO.lvclass/Public Events.ctl" = cluster{"Error":refnum<user-event>, "State":refnum<user-event>, "Reserve State":refnum<user-event>}
  T74 = typedef "Instrument.Lockin.lvlib/Instrument.DAQ.lvclass/PublicEvents--Cluster.ctl" = cluster{"getAIChannels":refnum<user-event>, "getAOChannels":refnum<user-event>, "getREFChannels":refnum<user-event>, "getWaveforms":refnum<user-event>, "getResults":refnum<user-event>, "getSweepWaveforms":refnum<user-event>, "getCalibration":refnum<user-event>, "getDAQState":refnum<user-event>, "getDAQconfig":refnum<user-event>, "getInputGain":refnum<user-event>, "getOutputGain":refnum<user-event>, "getInputOffset":refnum<user-event>, "getSampling":refnum<user-event>, "getSweepChannels":refnum<user-event>, "getDeviceIDN":refnum<user-event>}
  T75 = typedef "Instrument.lvlib/Instrument.lvclass/Instrument.IDN--cluster.ctl" = cluster{"vendor":string, "model":string, "serial":string, "firmware":string}
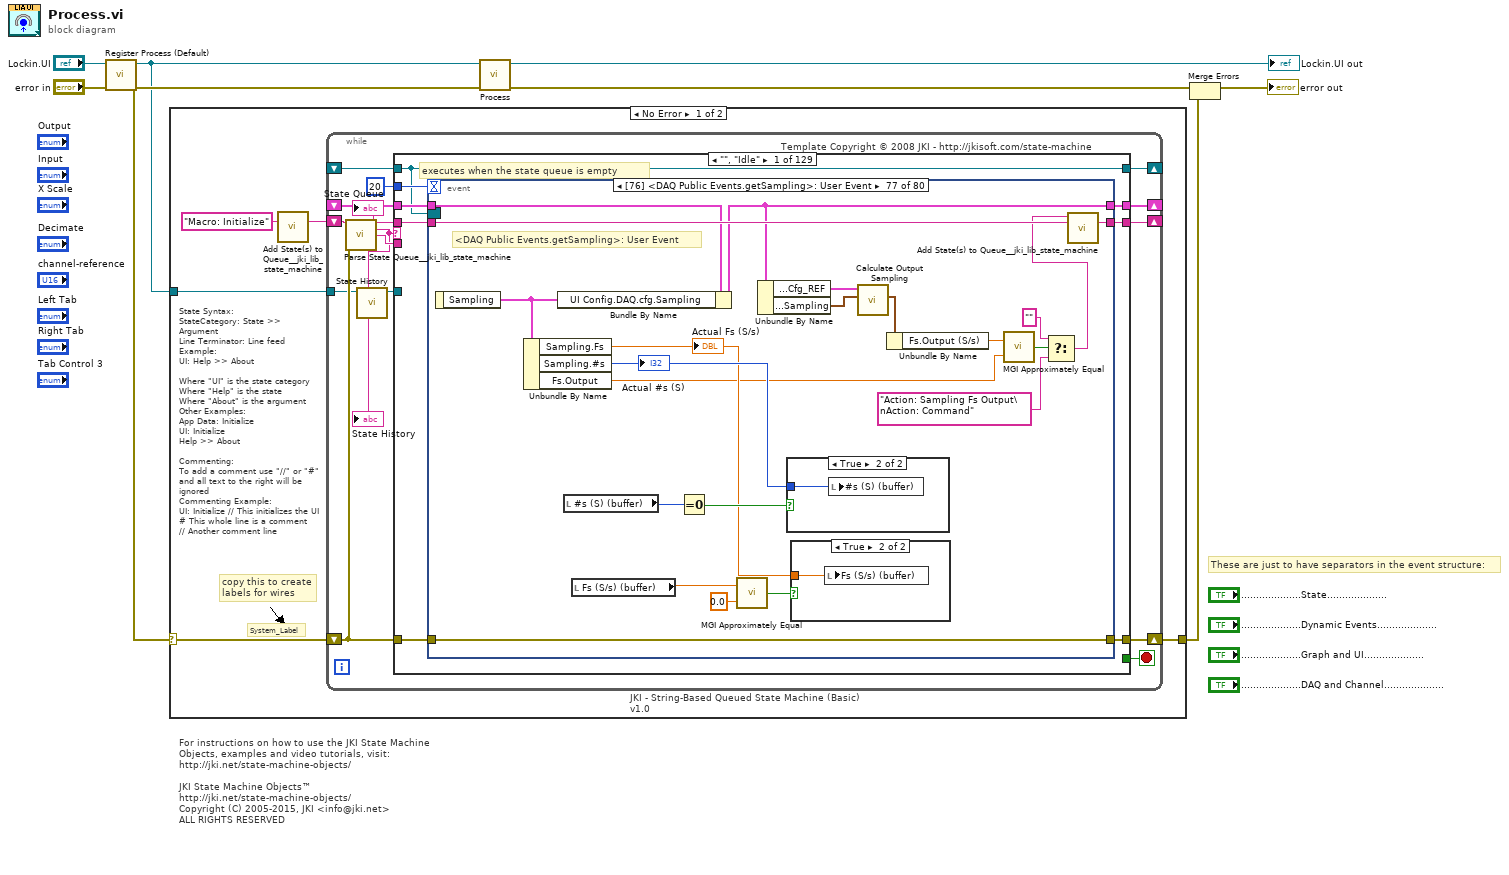
[diagram p0: block diagram]
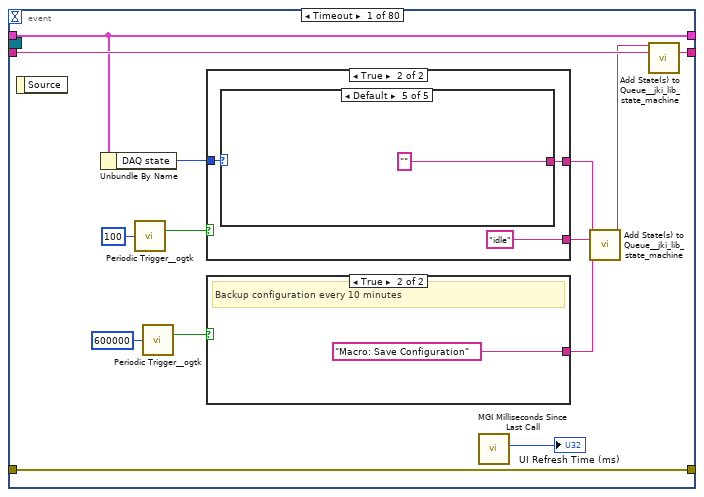
[diagram p2: hidden frame]
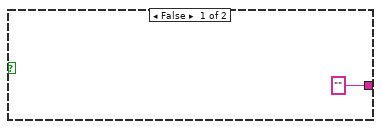
[diagram p3: hidden frame]
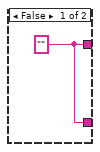
[diagram p4: hidden frame]
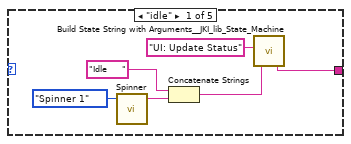
[diagram p5: hidden frame]
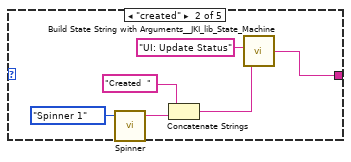
[diagram p6: hidden frame]
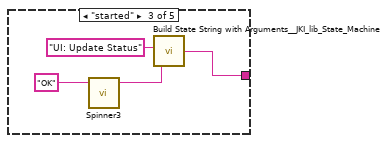
[diagram p7: hidden frame]
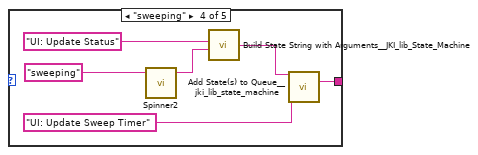
[diagram p8: hidden frame]
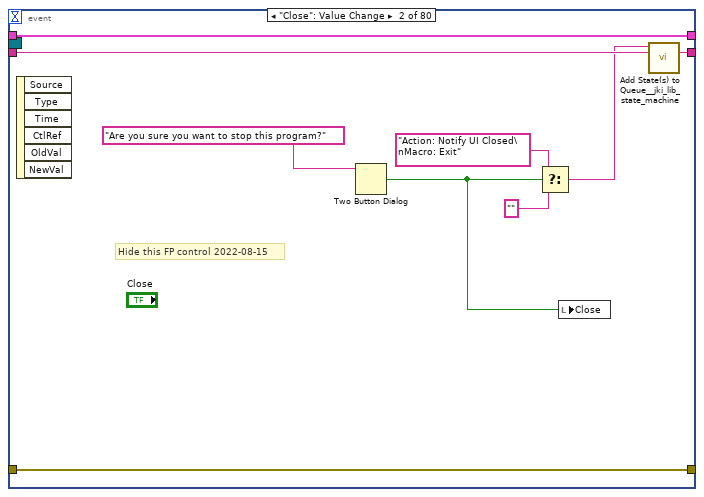
[diagram p9: hidden frame]
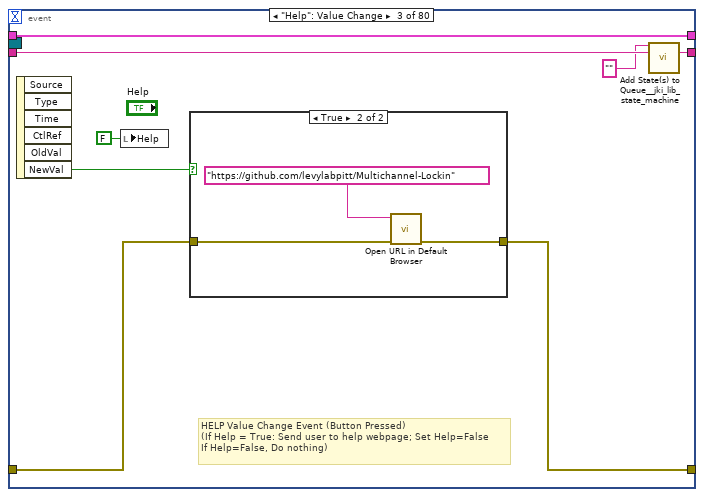
[diagram p10: hidden frame]
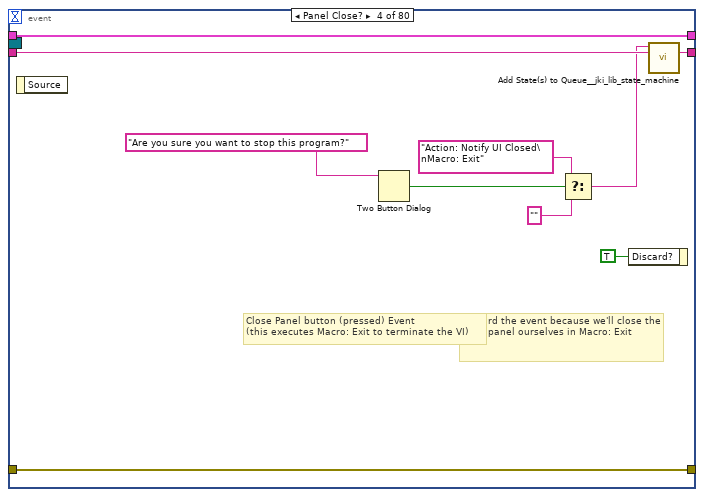
[diagram p12: hidden frame]
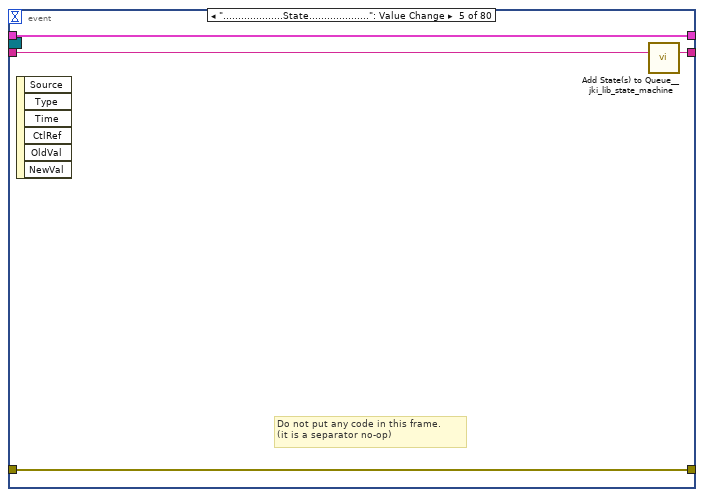
[diagram p13: hidden frame]
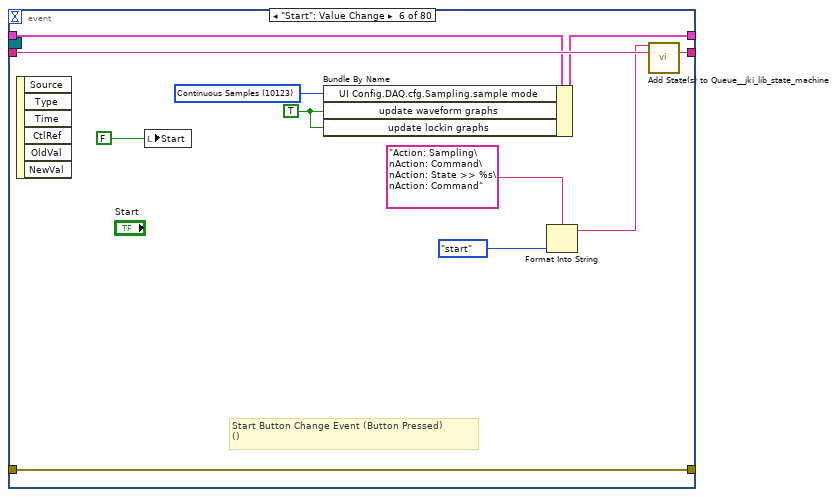
[diagram p14: hidden frame]
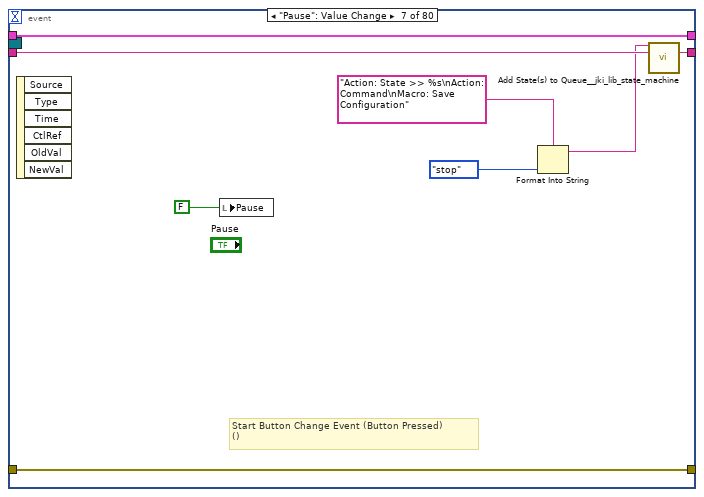
[diagram p15: hidden frame]
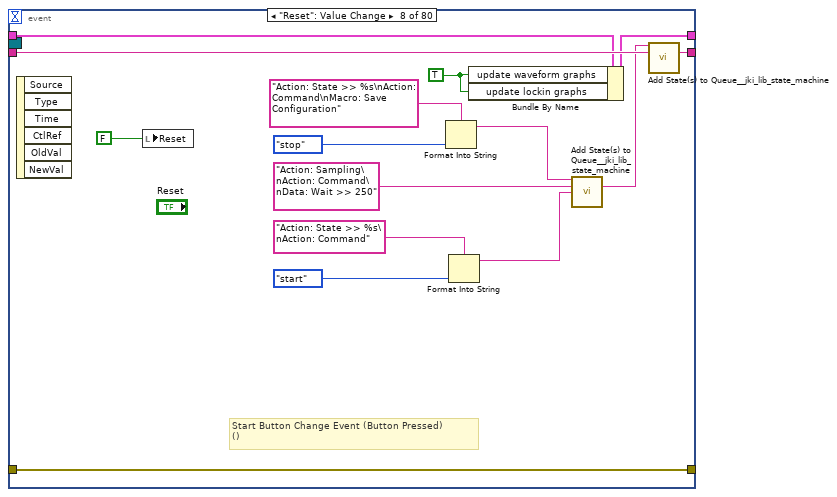
[diagram p16: hidden frame]
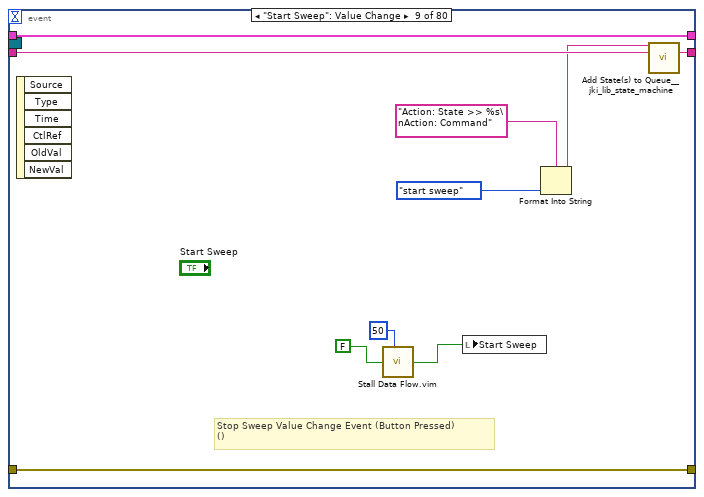
[diagram p17: hidden frame]
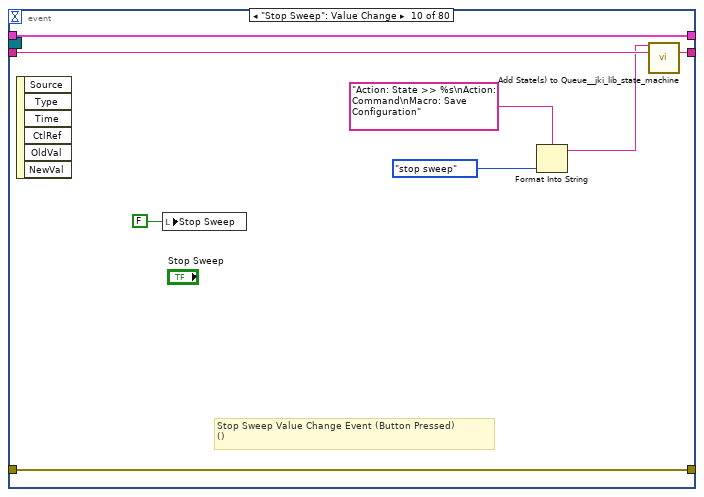
[diagram p18: hidden frame]
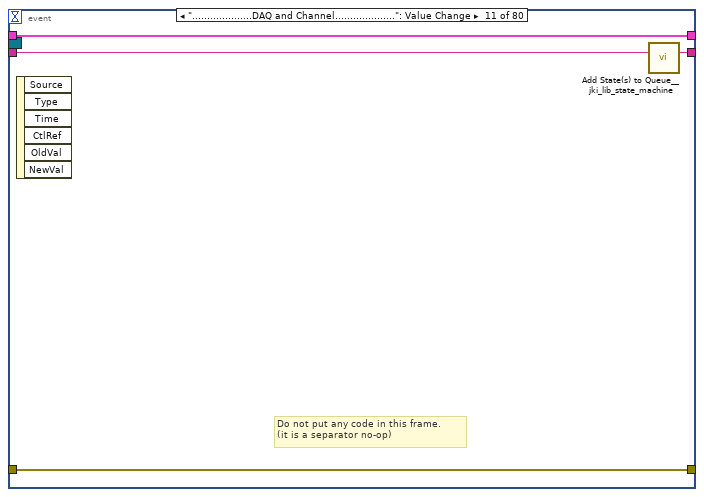
[diagram p19: hidden frame]
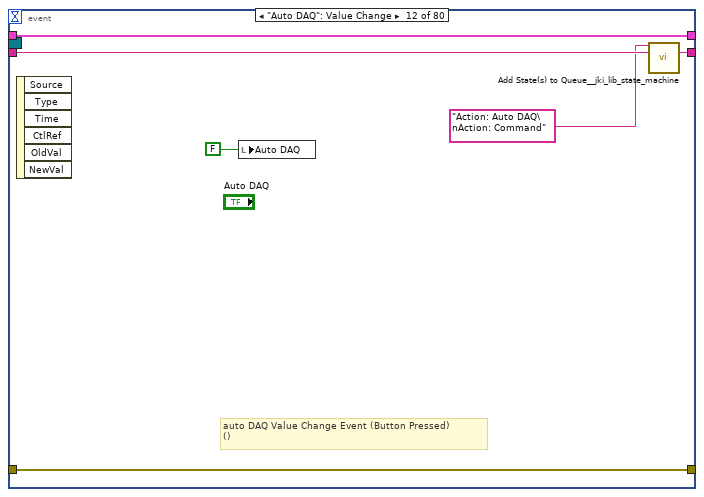
[diagram p20: hidden frame]
diagram:
  # "These are just to have separators in the event structure:"
  # "For instructions on how to use the JKI State Machine Objects, examples and video tutorials, visit:\nhttp://jki.net/state-machine-objects/\n\nJKI State Machine Objects™\nhttp://jki.net/state-machine-objects/\nCopyright (C) 2005-2015, JKI <info@jki.net>\nALL RIGHTS RESERVED"
  n1 = call <vilib>:"Register Process (Default).vi"("error in (no error)"="error in", "SMO"="Lockin.UI") -> ("error out"=w5:errorcluster, "SelfRef"=w4:refnum<class "Instrument UI.Lockin.lvclass">)  [unwired: 8 in]
  n2 = case shown="No Error" w5 {
    selector: w5 -> [w10 w2495]
    tunnel: w4 -> [w11 _]
    tunnel: [w9 w2495] -> w1
    frame No Error {
      # "State Syntax:\nStateCategory: State >> Argument\nLine Terminator: Line feed\nExample:\nUI: Help >> About\n\nWhere \"UI\" is the state category\nWhere \"Help\" is the state\nWhere \"About\" is the argument\nOther Examples:\nApp Data: Initialize\nUI: Initialize\nHelp >> About\n\nCommenting:\nTo add a comment use \"//\" or \"#\" and all text to the right will be ignored\nCommenting Example:\nUI: Initialize // This initializes the UI\n# This whole line is a comment\n// Another comment line"
      # "copy this to create labels for wires"
      # "System_Label"
      n3 = call <vilib>:"Add State(s) to Queue__jki_lib_state_machine.vi"("State(s) in (\"\")"="Macro: Initialize") -> ("States Out"=w13:string)  [unwired: 14 in]
      n4 = while "JKI - String-Based Queued State Machine (Basic) v1.0" {
        shift-right: [w24] -> _
        shift-left: _ -> [w23]
        shift-right: [w27] -> w9
        shift-left: w10 -> [w21]
        shift-right: [w26] -> _
        shift-left: w13 -> [w28]
        tunnel: w11 -> [w14]
        shift-right: [w20] -> _
        shift-left: _ -> [w19]
        stop <- w25 stop-if-true
        # "Template Copyright © 2008 JKI - http://jkisoft.com/state-machine"
        n5 = call <vilib>:"Parse State Queue__jki_lib_state_machine.vi"("State Queue"=w28, "Error In (no error)"=w21) -> ("Remaining States"=w16:string, "Current State"=w18:string, "Arguments"=w29:string)  [unwired: 11 in]
        "State Queue" <- w16
        n6 = call <userlib>:"State History.vi"("Current State"=w18, "SMO"=w14) -> ("SMO"=w15:refnum<class "Instrument UI.Lockin.lvclass">, "History"=→"State History":string)  [unwired: 8 in]
        n7 = case shown="\"\", \"Idle\"" w18 {
          selector: w18 -> [_ _ w792 _ _ _ _ _ _ _ _ _ _ _ _ _ _ _ _ _ _ _ _ _ _ _ _ _ _ _ _ _ _ _ _ _ _ _ _ _ _ _ _ _ _ _ _ _ _ _ _ _ _ _ _ _ _ _ _ _ _ _ _ _ _ _ _ _ _ _ _ _ _ _ _ _ _ _ _ _ _ _ _ _ _ _ _ _ _ _ _ _ _ _ _ _ _ _ _ _ _ _ _ _ _ _ _ _ _ _ _ _ _ _ _ _ _ _ _ _ _ _ _ _ _ _ _ _ _]
          tunnel: w16 -> [w37 w790 w796 w815 w818 w834 w839 w862 w883 w900 w929 w937 w944 w949 w963 w973 w986 w991 w1003 w1010 w1026 w1062 w1070 w1078 w1085 w1091 w1120 w1131 w1160 w1172 w1181 w1189 w1198 w1214 w1247 w1260 w1271 w1290 w1308 w1323 w1336 w1347 w1364 w1399 w1449 w1463 w1476 w1487 w1503 w1510 w1524 w1541 w1566 w1584 w1618 w1642 w1666 w1684 w1695 w1716 w1729 w1749 w1762 w1772 w1784 w1823 w1834 w1849 w1865 w1876 w1906 w1911 w1922 w1934 w1945 w1954 w1963 w1977 w1983 w1989 w1998 w2015 w2021 w2038 w2043 w2054 w2061 w2066 w2085 w2091 w2098 w2103 w2110 w2122 w2134 w2146 w2156 w2174 w2182 w2189 w2197 w2205 w2213 w2223 w2236 w2244 w2255 w2265 w2275 w2283 w2297 w2305 w2313 w2321 w2329 w2337 w2345 w2353 w2361 w2369 w2378 w2389 w2400 w2413 w2423 w2430 w2457 w2487 w2494]
          tunnel: w29 -> [_ _ _ _ _ _ _ _ _ _ _ w930 _ _ _ _ _ _ _ w1004 w1020 w1057 w1065 w1073 _ w1086 _ _ _ _ _ _ _ _ w1239 w1253 w1266 w1284 _ _ _ _ _ _ _ _ _ _ _ _ _ _ _ _ _ _ _ _ _ _ _ _ _ _ _ _ _ w1841 _ w1867 _ _ _ _ _ _ _ _ _ _ _ _ _ _ _ _ _ _ _ _ _ _ _ _ _ w2139 w2150 w2168 _ _ _ _ _ _ _ _ _ _ _ _ _ _ _ _ _ _ _ _ _ _ _ _ _ w2406 w2416 _ _ _ _]
          tunnel: w23 -> [w35 w787 w794 w806 w821 w830 w836 _ w864 w890 w924 w934 w939 w946 w959 w969 w982 w988 w997 w1008 w1022 w1058 w1067 w1075 w1082 w1088 w1101 w1127 w1155 w1163 w1173 w1184 w1194 w1203 w1241 w1255 w1267 w1285 w1305 w1312 w1333 w1344 w1361 w1395 w1446 w1460 w1473 w1484 w1500 w1507 w1521 w1538 w1562 w1579 w1594 w1627 w1663 w1678 w1687 w1712 w1722 w1745 w1759 w1767 w1780 w1820 w1829 w1846 w1862 w1868 w1890 w1908 w1918 w1924 w1942 w1951 w1960 w1974 w1979 w1985 w1990 w2004 w2018 w2024 w2040 w2051 w2056 w2063 w2083 w2089 w2092 w2099 w2106 w2118 w2130 w2141 w2151 w2169 w2177 w2184 w2192 w2200 w2208 w2214 w2231 w2239 w2250 w2260 w2270 w2278 w2292 w2300 w2308 w2316 w2324 w2332 w2340 w2348 w2356 w2364 w2373 w2384 w2393 w2408 w2418 w2425 w2454 w2481 w2488]
          tunnel: [w34 w788 w798 w812 w823 w829 w837 w852 w881 w898 w927 w935 w940 w947 w951 w968 w977 w989 w999 w1005 w1023 w1060 w1068 w1076 w1083 w1089 w1118 w1129 w1158 w1170 w1179 w1187 w1196 w1212 w1243 w1252 w1265 w1280 w1299 w1316 w1332 w1342 w1359 w1393 w1445 w1459 w1472 w1477 w1499 w1505 w1520 w1533 w1564 w1582 w1614 w1635 w1658 w1682 w1693 w1714 w1727 w1747 w1756 w1770 w1776 w1813 w1826 w1847 w1859 w1874 w1888 w1909 w1920 w1932 w1943 w1952 w1961 w1975 w1978 w1984 w1991 w2011 w2019 w2036 w2041 w2045 w2057 w2064 w2081 w2086 w2095 w2100 w2104 w2112 w2126 w2143 w2153 w2171 w2179 w2186 w2194 w2202 w2210 w2220 w2233 w2241 w2252 w2262 w2272 w2280 w2294 w2302 w2310 w2318 w2326 w2334 w2342 w2350 w2358 w2366 w2375 w2386 w2397 w2410 w2420 w2427 w2433 w2484 w2491] -> w27
          tunnel: w21 -> [w33 w788 w797 w812 w826 _ w837 w851 w881 w898 w927 w935 w941 w947 w957 w966 w978 w989 w1000 w1006 w1024 w1060 w1068 w1076 w1083 w1089 w1118 w1129 w1158 w1170 w1179 w1187 w1196 w1212 w1242 w1256 w1268 w1286 w1296 w1313 w1325 w1339 w1349 w1374 w1443 w1451 w1464 w1478 w1494 w1504 w1513 w1526 w1564 w1582 w1615 w1622 w1652 w1682 w1693 w1714 w1727 w1747 w1756 w1770 w1775 w1818 w1827 w1847 w1858 w1874 w1887 w1909 w1920 w1932 w1943 w1952 w1961 w1975 w1978 w1984 w1991 w2010 w2019 w2036 w2041 w2046 w2058 w2064 w2076 w2087 w2095 w2100 w2105 w2113 w2127 w2143 w2153 w2171 w2179 w2186 w2194 w2202 w2210 w2220 w2233 w2241 w2252 w2262 w2272 w2280 w2294 w2302 w2310 w2318 w2326 w2334 w2342 w2350 w2358 w2366 w2375 w2386 w2397 w2410 w2420 w2427 w2453 w2484 w2491]
          tunnel: [w36 w789 w795 w814 w817 w833 w838 w861 w882 w899 w928 w936 w943 w948 w962 w972 w985 w990 w1002 w1009 w1025 w1061 w1069 w1077 w1084 w1090 w1119 w1130 w1159 w1171 w1180 w1188 w1197 w1213 w1246 w1259 w1270 w1289 w1307 w1322 w1335 w1346 w1363 w1398 w1448 w1462 w1475 w1486 w1502 w1509 w1523 w1540 w1565 w1583 w1617 w1641 w1665 w1683 w1694 w1715 w1728 w1748 w1761 w1771 w1783 w1822 w1833 w1848 w1864 w1875 w1905 w1910 w1921 w1933 w1944 w1953 w1962 w1976 w1982 w1988 w1997 w2014 w2020 w2037 w2042 w2053 w2060 w2065 w2084 w2090 w2097 w2102 w2109 w2121 w2133 w2145 w2155 w2173 w2181 w2188 w2196 w2204 w2212 w2222 w2235 w2243 w2254 w2264 w2274 w2282 w2296 w2304 w2312 w2320 w2328 w2336 w2344 w2352 w2360 w2368 w2377 w2388 w2399 w2412 w2422 w2429 w2456 w2486 w2493] -> w26
          tunnel: [_ _ _ _ _ TRUE _ _ _ _ _ _ _ _ _ _ _ _ _ _ _ _ _ _ _ _ _ _ _ _ _ _ _ _ _ _ _ _ _ _ _ _ _ _ _ _ _ _ _ _ _ _ _ _ _ _ _ _ _ _ _ _ _ _ _ _ _ _ _ _ _ _ _ _ _ _ _ _ _ _ _ _ _ _ _ _ _ _ _ _ _ _ _ _ _ _ _ _ _ _ _ _ _ _ _ _ _ _ _ _ _ _ _ _ _ _ _ _ _ _ _ _ _ _ _ _ _ _ _] -> w25
          tunnel: [w32 w787 w794 w813 w820 w830 w836 w860 w879 w889 w924 w934 w939 w946 w960 w970 w983 w988 w997 w1008 w1022 w1058 w1067 w1075 w1082 w1088 w1101 w1127 w1156 w1164 w1173 w1184 w1194 w1203 w1241 w1255 w1267 w1285 w1304 w1312 w1333 w1344 w1361 w1395 w1446 w1460 w1473 w1484 w1500 w1507 w1521 w1538 w1562 w1579 w1595 w1627 w1663 w1678 w1687 w1712 w1722 w1745 w1759 w1767 w1780 w1820 w1829 w1846 w1862 w1870 w1890 w1908 w1918 w1925 w1942 w1951 w1960 w1974 w1979 w1985 w1990 w2004 w2018 w2025 w2040 w2051 w2056 w2063 w2083 w2089 w2093 w2099 w2106 w2119 w2131 w2142 w2152 w2170 w2178 w2185 w2193 w2201 w2209 w2215 w2232 w2240 w2251 w2261 w2271 w2279 w2293 w2301 w2309 w2317 w2325 w2333 w2341 w2349 w2357 w2365 w2374 w2385 w2396 w2409 w2419 w2426 w2454 w2482 w2489] -> w24
          tunnel: 20 ("Timeout") -> [w31 _ _ _ _ _ _ _ _ _ _ _ _ _ _ _ _ _ _ _ _ _ _ _ _ _ _ _ _ _ _ _ _ _ _ _ _ _ _ _ _ _ _ _ _ _ _ _ _ _ _ _ _ _ _ _ _ _ _ _ _ _ _ _ _ _ _ _ _ _ _ _ _ _ _ _ _ _ _ _ _ _ _ _ _ _ _ _ _ _ _ _ _ _ _ _ _ _ _ _ _ _ _ _ _ _ _ _ _ _ _ _ _ _ _ _ _ _ _ _ _ _ _ _ _ _ _ _ _]
          tunnel: w15 -> [_ _ _ _ _ _ _ w853 _ _ _ _ _ _ _ _ _ _ _ _ _ _ _ _ _ _ _ _ _ _ _ _ _ _ _ _ _ _ _ _ _ _ _ _ _ _ _ _ _ _ _ _ _ _ _ _ _ _ _ _ _ _ _ _ _ _ _ _ _ _ _ _ _ _ _ _ _ _ _ _ _ _ _ _ _ _ _ _ _ _ _ _ _ _ _ _ _ _ _ _ _ _ _ _ _ _ _ _ _ _ _ _ _ _ _ _ _ _ _ _ _ _ _ _ _ _ _ _ _]
          tunnel: [w30 w786 w791 w803 w828 w831 w835 w859 w880 w897 w926 w933 w938 w945 w961 w971 w984 w987 w1001 w1007 w1019 w1059 w1066 w1074 w1081 w1087 w1117 w1128 w1157 w1169 w1178 w1186 w1195 w1211 w1245 w1258 w1269 w1288 w1306 w1321 w1334 w1345 w1362 w1397 w1447 w1461 w1474 w1485 w1501 w1508 w1522 w1539 w1563 w1581 w1616 w1640 w1664 w1681 w1692 w1713 w1726 w1746 w1760 w1769 w1782 w1821 w1832 w1845 w1863 w1873 w1904 w1907 w1919 w1931 w1941 w1950 w1959 w1973 w1981 w1987 w1996 w2013 w2017 w2031 w2039 w2052 w2059 w2062 w2082 w2088 w2096 w2101 w2108 w2120 w2132 w2144 w2154 w2172 w2180 w2187 w2195 w2203 w2211 w2221 w2234 w2242 w2253 w2263 w2273 w2281 w2295 w2303 w2311 w2319 w2327 w2335 w2343 w2351 w2359 w2367 w2376 w2387 w2398 w2411 w2421 w2428 w2455 w2485 w2492] -> w20
          tunnel: w19 -> [w30 w786 w791 w803 w828 w831 w835 w859 w880 w897 w926 w933 w938 w945 w961 w971 w984 w987 w1001 w1007 w1019 w1059 w1066 w1074 w1081 w1087 w1117 w1128 w1157 w1169 w1178 w1186 w1195 w1211 w1245 w1258 w1269 w1288 w1306 w1321 w1334 w1345 w1362 w1397 w1447 w1461 w1474 w1485 w1501 w1508 w1522 w1539 w1563 w1581 w1616 w1640 w1664 w1681 w1692 w1713 w1726 w1746 w1760 w1769 w1782 w1821 w1832 w1845 w1863 w1873 w1904 w1907 w1919 w1931 w1941 w1950 w1959 w1973 w1981 w1987 w1996 w2013 w2017 w2031 w2039 w2052 w2059 w2062 _ w2088 w2096 w2101 w2108 w2120 w2132 w2144 w2154 w2172 w2180 w2187 w2195 w2203 w2211 w2221 w2234 w2242 w2253 w2263 w2273 w2281 w2295 w2303 w2311 w2319 w2327 w2335 w2343 w2351 w2359 w2367 w2376 w2387 w2398 w2411 w2421 w2428 w2455 w2485 w2492]
          frame "", "Idle" {
            # "executes when the state queue is empty"
            n8 = event shown="[76] <DAQ Public Events.getSampling>: User Event" {
              selector: w30 -> [_ _ _ _ _ _ _ _ _ _ _ _ _ _ _ _ _ _ _ _ _ _ _ _ _ _ _ _ _ _ _ _ _ _ _ _ _ _ _ _ _ _ _ _ _ _ _ _ _ _ _ _ _ _ _ _ _ _ _ _ _ _ _ _ _ _ _ _ _ _ _ _ _ _ _ _ _ _ _ _]
              dyn-events: _ -> [_ _ _ _ _ _ _ _ _ _ _ _ _ _ _ _ _ _ _ _ _ _ _ _ _ _ _ _ _ _ _ _ _ _ _ _ _ _ _ _ _ _ _ _ _ _ _ _ _ _ _ _ _ _ _ _ _ _ _ _ _ _ _ _ _ _ _ _ _ _ _ _ _ _ _ _ _ _ _ _]
              timeout: w31 -> [_ _ _ _ _ _ _ _ _ _ _ _ _ _ _ _ _ _ _ _ _ _ _ _ _ _ _ _ _ _ _ _ _ _ _ _ _ _ _ _ _ _ _ _ _ _ _ _ _ _ _ _ _ _ _ _ _ _ _ _ _ _ _ _ _ _ _ _ _ _ _ _ _ _ _ _ _ _ _ _]
              tunnel: w37 -> [w51 w89 w97 w111 w115 w126 w134 w149 w159 w167 w171 w177 w184 w190 w201 w220 w233 w240 w247 w255 w273 w290 w297 w304 w311 w318 w325 w332 w340 w351 w362 w373 w383 w391 w399 w405 w414 w430 w442 w449 w456 w463 w470 w477 w481 w486 w491 w496 w501 w506 w515 w531 w545 w557 w569 w584 w589 w594 w599 w604 w608 w613 w618 w622 w631 w637 w653 w668 w681 w688 w695 w702 w709 w716 w733 w740 w762 w771 w778 w785]
              tunnel: [w50 w88 w96 w110 w114 w125 w133 w148 w158 w166 w170 w176 w183 w189 w200 w219 w232 w239 w246 w254 w272 w289 w296 w303 w310 w317 w324 w331 w339 w350 w361 w372 w382 w390 w398 w404 w413 w429 w441 w448 w455 w462 w469 w476 w480 w485 w490 w495 w500 w505 w514 w530 w544 w556 w568 w583 w588 w593 w598 w603 w607 w612 w617 w621 w630 w636 w652 w667 w680 w687 w694 w701 w708 w715 w732 w739 w761 w770 w777 w784] -> w36
              tunnel: w35 -> [w48 w86 w94 w108 w113 w118 w127 w137 w154 w161 w169 w172 w179 w185 w197 w211 w228 w235 w241 w248 w264 w285 w292 w299 w306 w313 w320 w327 w335 w345 w356 w367 w378 w386 w394 w400 w409 w417 w436 w443 w453 w460 w467 w474 w479 w482 w487 w492 w497 w502 w510 w528 w542 w554 w566 w581 w586 w592 w596 w601 w606 w610 w615 w619 w628 w634 w645 w662 w674 w683 w691 w697 w705 w711 w725 w735 w759 w766 w773 w780]
              tunnel: [w49 w87 w93 w107 w112 w123 w131 w146 w153 w164 w168 w173 w181 w188 w199 w214 w231 w238 w245 w253 w271 w287 w294 w301 w308 w315 w322 w329 w337 w348 w359 w370 w380 w388 w396 w401 w411 w427 w440 w447 w454 w461 w468 w475 w478 w483 w488 w493 w498 w503 w512 w529 w543 w555 w567 w582 w585 w591 w595 w600 w605 w611 w616 w620 w629 w635 w651 w666 w677 w686 w693 w700 w707 w714 w731 w738 w760 w769 w776 w783] -> w34
              tunnel: w33 -> [w49 w87 w92 w107 w112 w123 w131 w146 w153 w164 w168 w173 w181 w188 w199 w214 w231 w238 w245 w253 w271 w287 w294 w301 w308 w315 w322 w329 w337 w348 w359 w370 w380 w388 w396 w401 w411 w427 w440 w447 w454 w461 w468 w475 w478 w483 w488 w493 w498 w503 w512 w529 w543 w555 w567 w582 w585 w591 w595 w600 w605 w611 w616 w620 w629 w635 w651 w666 w677 w686 w693 w700 w707 w714 w731 w738 w760 w769 w776 w783]
              tunnel: [w48 w86 w94 w108 w113 w119 w127 w136 w154 w161 w169 w172 w180 w187 w198 w213 w230 w237 w244 w252 w263 w286 w293 w300 w307 w314 w321 w328 w336 w344 w355 w366 w379 w387 w395 w400 w410 w426 w436 w443 w453 w460 w467 w474 w479 w482 w487 w492 w497 w502 w511 w528 w542 w554 w566 w581 w586 w592 w596 w601 w606 w610 w615 w619 w628 w634 w650 w661 w679 w684 w692 w699 w706 w712 w730 w736 w750 w767 w774 w781] -> w32
              event Timeout {
                n9 = event-data() -> ()  [unwired: 1 in, 1 out]
                n10 = Unbundle By Name(w48) -> ("DAQ state"=w47:T33)
                n11 = call <userlib>:"Periodic Trigger__ogtk.vi"("time (ms)"=u32 100) -> ("Triggered"=w45:bool)  [unwired: 12 in, 2 out]
                n12 = call <userlib>:"Periodic Trigger__ogtk.vi"("time (ms)"=u32 600000) -> ("Triggered"=w42:bool)  [unwired: 12 in, 2 out]
                n13 = case shown="True" w45 {
                  tunnel: w47 -> [_ w57]
                  tunnel: [w54 w56] -> w40
                  tunnel: [w54 "idle"] -> w38
                  frame False {
                    w54 = "" ("States Out")
                  }
                  frame True {
                    n14 = case shown="Default" w57 {
                      tunnel: [w58 w64 w72 w76 ""] -> w56
                      frame "idle" {
                        n15 = call "Spinner.vi"("Enum"=T28."Spinner 1") -> ("Spinner Out"=w61:string)  [unwired: 4 in]
                        n16 = Concatenate Strings("Idle     " ("Status"), w61) -> (w59:string)
                        n17 = call <vilib>:"Build State String with Arguments__JKI_lib_State_Machine.vi"("Arguments (\"\")"=w59, "State"="UI: Update Status") -> ("State with Arguments"=w58:string)  [unwired: 4 in]
                      }
                      frame "created" {
                        n18 = call "Spinner.vi"("Enum"=T28."Spinner 1") -> ("Spinner Out"=w67:string)  [unwired: 4 in]
                        n19 = Concatenate Strings("Created  " ("Status"), w67) -> (w65:string)
                        n20 = call <vilib>:"Build State String with Arguments__JKI_lib_State_Machine.vi"("Arguments (\"\")"=w65, "State"="UI: Update Status") -> ("State with Arguments"=w64:string)  [unwired: 4 in]
                      }
                      frame "started" {
                        n21 = call "Spinner3.vi"("String In"="OK") -> ("Spinner Out"=w70:string)  [unwired: 4 in]
                        n22 = call <vilib>:"Build State String with Arguments__JKI_lib_State_Machine.vi"("Arguments (\"\")"=w70, "State"="UI: Update Status") -> ("State with Arguments"=w72:string)  [unwired: 4 in]
                      }
                      frame "sweeping" {
                        n23 = call "Spinner2.vi"("String In"="sweeping") -> ("Spinner Out"=w74:string)  [unwired: 4 in]
                        n24 = call <vilib>:"Build State String with Arguments__JKI_lib_State_Machine.vi"("Arguments (\"\")"=w74, "State"="UI: Update Status") -> ("State with Arguments"=w78:string)  [unwired: 4 in]
                        n25 = call <vilib>:"Add State(s) to Queue__jki_lib_state_machine.vi"("State(s) in Front (\"\")"=w78, "State(s) at Back (\"\")"="UI: Update Sweep Timer") -> ("States Out"=w76:string)  [unwired: 13 in]
                      }
                      frame Default {
                      }
                    }
                  }
                }
                n26 = case shown="True" w42 {
                  tunnel: ["" "Macro: Save Configuration"] -> w41
                  frame False {
                  }
                  frame True {
                    # "Backup configuration every 10 minutes"
                  }
                }
                n27 = call <userlib>:"MGI Milliseconds Since Last Call.vi"() -> ("ms"=→"UI Refresh Time (ms)":u32)  [unwired: 6 in, 1 out]
                n28 = call <vilib>:"Add State(s) to Queue__jki_lib_state_machine.vi"("State(s) in Front (\"\")"=w40, "State(s) in (\"\")"=w38, "State(s) at Back (\"\")"=w41) -> ("States Out"=w39:string)  [unwired: 12 in]
                n29 = call <vilib>:"Add State(s) to Queue__jki_lib_state_machine.vi"("State(s) in Front (\"\")"=w39, "State(s) in (\"\")"=w51) -> ("States Out"=w50:string)  [unwired: 13 in]
              }
              event "Close": Value Change {
                # "Hide this FP control 2022-08-15"
                n30 = event-data() -> ()  [unwired: 1 in, 6 out]
                n31 = Two Button Dialog(message="Are you sure you want to stop this program?") -> (T button?=w81:bool)  [unwired: 2 in]
                n32 = Select(t="Action: Notify UI Closed\nMacro: Exit", s=w81, f="") -> (s? t:f=w82:string)
                n33 = local write "Close"(w81) -> ()
                n34 = call <vilib>:"Add State(s) to Queue__jki_lib_state_machine.vi"("State(s) in Front (\"\")"=w82, "State(s) in (\"\")"=w89) -> ("States Out"=w88:string)  [unwired: 13 in]
              }
              event "Help": Value Change {
                # "HELP Value Change Event (Button Pressed)\n(If Help = True: Send user to help webpage; Set Help=False\nIf Help=False, Do nothing)"
                n35 = event-data() -> ("NewVal"=w91:bool)  [unwired: 1 in, 5 out]
                n36 = local write "Help"(FALSE ("Help")) -> ()
                n37 = case shown="True" w91 {
                  tunnel: w92 -> [w98 w101]
                  tunnel: [w98 w100] -> w93
                  frame False {
                  }
                  frame True {
                    n38 = call-poly <vilib>:"Open URL in Default Browser.vi"("error in (no error)"=w101, "URL"="https://github.com/levylabpitt/Multichannel-Lockin") -> ("error out"=w100:errorcluster)  [unwired: 4 in, 1 out]
                  }
                }
                n39 = call <vilib>:"Add State(s) to Queue__jki_lib_state_machine.vi"("State(s) in Front (\"\")"="", "State(s) in (\"\")"=w97) -> ("States Out"=w96:string)  [unwired: 13 in]
              }
              event Panel Close? {
                # "Discard the event because we'll close the front panel ourselves in Macro: Exit"
                # "Close Panel button (pressed) Event\n(this executes Macro: Exit to terminate the VI)"
                n40 = event-data() -> ()  [unwired: 1 in, 1 out]
                n41 = Two Button Dialog(message="Are you sure you want to stop this program?") -> (T button?=w106:bool)  [unwired: 2 in]
                n42 = Select(t="Action: Notify UI Closed\nMacro: Exit", s=w106, f="") -> (s? t:f=w102:string)
                n43 = event-data("Discard?"=TRUE) -> ()  [unwired: 1 in, 1 out]
                n44 = call <vilib>:"Add State(s) to Queue__jki_lib_state_machine.vi"("State(s) in Front (\"\")"=w102, "State(s) in (\"\")"=w111) -> ("States Out"=w110:string)  [unwired: 13 in]
              }
              event "....................State....................": Value Change {
                # "Do not put any code in this frame.\n(it is a separator no-op)"
                n45 = event-data() -> ()  [unwired: 1 in, 6 out]
                n46 = call <vilib>:"Add State(s) to Queue__jki_lib_state_machine.vi"("State(s) in (\"\")"=w115) -> ("States Out"=w114:string)  [unwired: 14 in]
              }
              event "Start": Value Change {
                w116 = TRUE ("update graphs")
                w117 = T43 10123 items=["Finite Samples"=10178, "Continuous Samples"=10123] ("UI Config.DAQ.Sampling.Sample Mode")
                # "Start Button Change Event (Button Pressed)\n()"
                n47 = event-data() -> ()  [unwired: 1 in, 6 out]
                n48 = local write "Start"(FALSE ("Help")) -> ()
                n49 = Bundle By Name(cluster=w118, "UI Config.DAQ.cfg.Sampling.sample mode"=w117, "update waveform graphs"=w116, "update lockin graphs"=w116) -> (w119:T65)
                n50 = Format Into String(format string="Action: Sampling\nAction: Command\nAction: State >> %s\nAction: Command", State--enum."start" ("State")) -> (resulting string=w120:string)  [unwired: 2 in, 1 out]
                n51 = call <vilib>:"Add State(s) to Queue__jki_lib_state_machine.vi"("State(s) in Front (\"\")"=w120, "State(s) in (\"\")"=w126) -> ("States Out"=w125:string)  [unwired: 13 in]
              }
              event "Pause": Value Change {
                # "Start Button Change Event (Button Pressed)\n()"
                n52 = event-data() -> ()  [unwired: 1 in, 6 out]
                n53 = local write "Pause"(FALSE ("Help")) -> ()
                n54 = Format Into String(format string="Action: State >> %s\nAction: Command\nMacro: Save Configuration", State--enum."stop" ("State")) -> (resulting string=w128:string)  [unwired: 2 in, 1 out]
                n55 = call <vilib>:"Add State(s) to Queue__jki_lib_state_machine.vi"("State(s) in Front (\"\")"=w128, "State(s) in (\"\")"=w134) -> ("States Out"=w133:string)  [unwired: 13 in]
              }
              event "Reset": Value Change {
                w135 = TRUE
                # "Start Button Change Event (Button Pressed)\n()"
                n56 = event-data() -> ()  [unwired: 1 in, 6 out]
                n57 = local write "Reset"(FALSE ("Help")) -> ()
                n58 = Format Into String(format string="Action: State >> %s\nAction: Command\nMacro: Save Configuration", State--enum."stop" ("State")) -> (resulting string=w141:string)  [unwired: 2 in, 1 out]
                n59 = Format Into String(format string="Action: State >> %s\nAction: Command", State--enum."start" ("State")) -> (resulting string=w139:string)  [unwired: 2 in, 1 out]
                n60 = Bundle By Name(cluster=w137, "update waveform graphs"=w135, "update lockin graphs"=w135) -> (w136:T65)
                n61 = call <vilib>:"Add State(s) to Queue__jki_lib_state_machine.vi"("State(s) in Front (\"\")"=w141, "State(s) in (\"\")"="Action: Sampling\nAction: Command\nData: Wait >> 250", "State(s) at Back (\"\")"=w139) -> ("States Out"=w138:string)  [unwired: 12 in]
                n62 = call <vilib>:"Add State(s) to Queue__jki_lib_state_machine.vi"("State(s) in Front (\"\")"=w138, "State(s) in (\"\")"=w149) -> ("States Out"=w148:string)  [unwired: 13 in]
              }
              event "Start Sweep": Value Change {
                # "Stop Sweep Value Change Event (Button Pressed)\n()"
                n63 = event-data() -> ()  [unwired: 1 in, 6 out]
                n64 = call "Stall Data Flow.vim"("value in"=FALSE ("Start Sweep"), "milliseconds to wait"=u32 50) -> ("value out"=w150:bool)  [unwired: 1 out]
                n65 = local write "Start Sweep"(w150) -> ()
                n66 = Format Into String(format string="Action: State >> %s\nAction: Command", State--enum."start sweep" ("State")) -> (resulting string=w156:string)  [unwired: 2 in, 1 out]
                n67 = call <vilib>:"Add State(s) to Queue__jki_lib_state_machine.vi"("State(s) in Front (\"\")"=w156, "State(s) in (\"\")"=w159) -> ("States Out"=w158:string)  [unwired: 13 in]
              }
              event "Stop Sweep": Value Change {
                # "Stop Sweep Value Change Event (Button Pressed)\n()"
                n68 = event-data() -> ()  [unwired: 1 in, 6 out]
                n69 = local write "Stop Sweep"(FALSE ("Help")) -> ()
                n70 = Format Into String(format string="Action: State >> %s\nAction: Command\nMacro: Save Configuration", State--enum."stop sweep" ("State")) -> (resulting string=w160:string)  [unwired: 2 in, 1 out]
                n71 = call <vilib>:"Add State(s) to Queue__jki_lib_state_machine.vi"("State(s) in Front (\"\")"=w160, "State(s) in (\"\")"=w167) -> ("States Out"=w166:string)  [unwired: 13 in]
              }
              event "....................DAQ and Channel....................": Value Change {
                # "Do not put any code in this frame.\n(it is a separator no-op)"
                n72 = event-data() -> ()  [unwired: 1 in, 6 out]
                n73 = call <vilib>:"Add State(s) to Queue__jki_lib_state_machine.vi"("State(s) in (\"\")"=w171) -> ("States Out"=w170:string)  [unwired: 14 in]
              }
              event "Auto DAQ": Value Change {
                # "auto DAQ Value Change Event (Button Pressed)\n()"
                n74 = event-data() -> ()  [unwired: 1 in, 6 out]
                n75 = local write "Auto DAQ"(FALSE ("Help")) -> ()
                n76 = call <vilib>:"Add State(s) to Queue__jki_lib_state_machine.vi"("State(s) in Front (\"\")"="Action: Auto DAQ\nAction: Command", "State(s) in (\"\")"=w177) -> ("States Out"=w176:string)  [unwired: 13 in]
              }
              event Value Change {
                # "DAQ Config Value Change Event (Button Pressed)\n()"
                n77 = event-data() -> ()  [unwired: 1 in, 6 out]
                n78 = Bundle By Name(cluster=w179, "UI Config.DAQ.Configuration"="DAQ Config") -> (w180:T65)
                n79 = call <vilib>:"Add State(s) to Queue__jki_lib_state_machine.vi"("State(s) in Front (\"\")"="Action: DAQ Config\nAction: Command", "State(s) in (\"\")"=w184) -> ("States Out"=w183:string)  [unwired: 13 in]
              }
              event "Actual Fs (S/s)", "Actual #s (S)": Value Change {
                # "DAQ Config Value Change Event (Button Pressed)\n()"
                n80 = event-data() -> ()  [unwired: 1 in, 6 out]
                n81 = disable-structure shown="Disabled" {
                  disable-tunnel: [w194 w195] -> w187
                  disable-tunnel: ["Action: Sampling\nAction: Command" _] -> w186
                  disable-tunnel: w185 -> [w192 w195]
                  frame Disabled {
                    n82 = local read "Fs Output (S/s)"() -> (w191:dbl)
                    n83 = Bundle By Name(cluster=w192) -> (w194:T65)  [unwired: 2 in]
                    n84 = property on="Fs Output (S/s)" class="DigNum (strict)"("Val(Sgnl)"=w191) -> ()  [unwired: 2 in, 2 out]
                  }
                  frame Enabled {
                  }
                }
                n85 = call <vilib>:"Add State(s) to Queue__jki_lib_state_machine.vi"("State(s) in Front (\"\")"=w186, "State(s) in (\"\")"=w190) -> ("States Out"=w189:string)  [unwired: 13 in]
              }
              event "Fs Output (S/s)": Value Change {
                # "DAQ Config Value Change Event (Button Pressed)\n()"
                n86 = event-data() -> ()  [unwired: 1 in, 6 out]
                n87 = disable-structure shown="Disabled" {
                  disable-tunnel: [w208 w209] -> w198
                  disable-tunnel: w197 -> [w207 w209]
                  disable-tunnel: ["Action: Sampling Fs Output\nAction: Command" _] -> w196
                  frame Disabled {
                    n88 = Unbundle By Name(w207) -> ("UI Config.DAQ.cfg.Sampling.Sampling.Fs"=w205:dbl, "UI Config.DAQ.cfg.Sampling.Sampling.#s"=w206:i32)
                    n89 = Divide(x=w205, y=w206) -> (x/y=w204:dbl)
                    n90 = In Range and Coerce(upper limit=w205, lower limit=w204) -> (coerced(x)=w203:dbl)  [unwired: 1 in, 1 out]
                    n91 = local write "Fs Output (S/s)"(w203) -> ()
                    n92 = Bundle By Name(cluster=w207, "UI Config.DAQ.cfg.Sampling.Fs.Output"=w203) -> (w208:T65)
                  }
                  frame Enabled {
                  }
                }
                n93 = call <vilib>:"Add State(s) to Queue__jki_lib_state_machine.vi"("State(s) in Front (\"\")"=w196, "State(s) in (\"\")"=w201) -> ("States Out"=w200:string)  [unwired: 13 in]
              }
              event Value Change {
                n94 = event-data() -> ()  [unwired: 1 in, 6 out]
                n95 = control-ref of="Fs Multiplier"() -> (w218:refnum<vi>)
                n96 = control-ref of="Refresh Rate (Hz)"() -> (w217:refnum<vi>)
                n97 = Bundle By Name(cluster=w211, "UI Config.DAQ.cfg.Sampling.Fs Mode"="Fs Mode") -> (w213:T65)
                n98 = case shown="\"Manual\"" "Fs Mode" {
                  tunnel: [FALSE ("Visible") TRUE ("Visible") FALSE ("Visible")] -> w216
                  tunnel: [FALSE ("Visible") FALSE ("Visible") TRUE ("Visible")] -> w215
                  frame "Manual" {
                  }
                  frame "Auto Fs" {
                  }
                  frame "Max Fs" {
                  }
                }
                n99 = property class="DigNum (strict)"(reference=w218, "Visible"=w216) -> ()  [unwired: 1 in, 2 out]
                n100 = property class="DigNum (strict)"(reference=w217, "Visible"=w215) -> ()  [unwired: 1 in, 2 out]
                n101 = call <vilib>:"Add State(s) to Queue__jki_lib_state_machine.vi"("State(s) in Front (\"\")"="Action: Sampling Fs Mode\nAction: Command", "State(s) in (\"\")"=w220) -> ("States Out"=w219:string)  [unwired: 13 in]
              }
              event "Fs Multiplier": Value Change {
                # "DAQ Config Value Change Event (Button Pressed)\n()"
                n102 = event-data() -> ()  [unwired: 1 in, 6 out]
                n103 = Bundle By Name(cluster=w228, "UI Config.DAQ.cfg.Sampling.Fs Multiplier"="Fs Multiplier") -> (w230:T65)
                n104 = call <vilib>:"Add State(s) to Queue__jki_lib_state_machine.vi"("State(s) in Front (\"\")"="Action: Sampling Fs Multiplier\nAction: Command", "State(s) in (\"\")"=w233) -> ("States Out"=w232:string)  [unwired: 13 in]
              }
              event "Refresh Rate (Hz)": Value Change {
                # "DAQ Config Value Change Event (Button Pressed)\n()"
                n105 = event-data() -> ()  [unwired: 1 in, 6 out]
                n106 = Bundle By Name(cluster=w235, "UI Config.DAQ.cfg.Sampling.Refresh Rate (Hz)"="Refresh Rate (Hz)") -> (w237:T65)
                n107 = call <vilib>:"Add State(s) to Queue__jki_lib_state_machine.vi"("State(s) in Front (\"\")"="Action: Sampling Refresh Rate\nAction: Command", "State(s) in (\"\")"=w240) -> ("States Out"=w239:string)  [unwired: 13 in]
              }
              event "Decimation (pre DSP)": Value Change {
                # "Decimation Value Change Event (Button Pressed)\n()"
                n108 = event-data() -> ()  [unwired: 1 in, 6 out]
                n109 = Bundle By Name(cluster=w241, "UI Config.DAQ.cfg.Sampling.Decimation.PreDSP"="Decimation (pre DSP)") -> (w244:T65)
                n110 = call <vilib>:"Add State(s) to Queue__jki_lib_state_machine.vi"("State(s) in Front (\"\")"="Action: Sampling Decimation Pre DSP\nAction: Command", "State(s) in (\"\")"=w247) -> ("States Out"=w246:string)  [unwired: 13 in]
              }
              event "Decimation (post DSP)": Value Change {
                # "hide from user for now (8/12/2022)"
                # "Decimation Value Change Event (Button Pressed)\n()"
                n111 = event-data() -> ()  [unwired: 1 in, 6 out]
                n112 = Unbundle By Name(w248) -> ("DAQ state"=w250:T33)
                n113 = Bundle By Name(cluster=w248, "UI Config.DAQ.cfg.Sampling.Decimation.PostDSP"="Decimation (post DSP)") -> (w252:T65)
                n114 = case shown="\"started\"" w250 {
                  tunnel: ["Action: Sampling Decimation Post DSP\nAction: Command" w258] -> w249
                  frame Default {
                  }
                  frame "started" {
                    n115 = Format Into String(format string="Action: State >> %s\nAction: Command\nAction: Sampling Decimation Post DSP\nAction: Command\nAction: State >> %s\nAction: Command", State--enum."stop" ("State"), State--enum."start" ("State")) -> (resulting string=w258:string)  [unwired: 2 in, 1 out]
                  }
                }
                n116 = call <vilib>:"Add State(s) to Queue__jki_lib_state_machine.vi"("State(s) in Front (\"\")"=w249, "State(s) in (\"\")"=w255) -> ("States Out"=w254:string)  [unwired: 13 in]
              }
              event Value Change {
                # "check if ref index changed"
                # "AI Channels Value Change Event (Button Pressed)\n()"
                n117 = event-data() -> ("OldVal"=w270:T4, "NewVal"=w266:T4)  [unwired: 1 in, 4 out]
                n118 = Not Equal?(x=w270, y=w266) -> (x != y?=w269:T66)
                n119 = for {
                  tunnel: w269 -> [w283] mode=indexing
                  tunnel: [w282] -> w268 mode=indexing
                  n120 = Unbundle By Name(w283) -> ("reference index"=w282:bool)
                }
                n121 = Search 1D Array(1D array=w268, element=TRUE) -> (index of element=w265:i32)  [unwired: 1 in]
                n122 = case shown="-1" w265 {
                  selector: w265 -> [_ w280]
                  tunnel: w264 -> [w277 w281]
                  tunnel: [w276 w281] -> w263
                  tunnel: ["Action: AI Channels\nAction: Command" w278] -> w262
                  tunnel: "AI Channels" -> [w274 _]
                  frame -1 {
                    # "something else changed, alert DAQ process"
                    n123 = Bundle By Name(cluster=w277, "UI Config.Channels.Cfg_AI"=w274) -> (w276:T65)
                  }
                  frame Default {
                    n124 = Format Into String(format string="UI: Sync AI Ref Array >> %d", w280) -> (resulting string=w278:string)  [unwired: 2 in, 1 out]
                  }
                }
                n125 = call <vilib>:"Add State(s) to Queue__jki_lib_state_machine.vi"("State(s) in Front (\"\")"=w262, "State(s) in (\"\")"=w273) -> ("States Out"=w272:string)  [unwired: 13 in]
              }
              event Value Change {
                # "AO Channels Value Change Event (Button Pressed)\n()"
                n126 = event-data() -> ()  [unwired: 1 in, 6 out]
                n127 = Bundle By Name(cluster=w285, "UI Config.Channels.Cfg_AO"="AO Channels") -> (w286:T65)
                n128 = call <vilib>:"Add State(s) to Queue__jki_lib_state_machine.vi"("State(s) in Front (\"\")"="Action: AO Channels\nAction: Command", "State(s) in (\"\")"=w290) -> ("States Out"=w289:string)  [unwired: 13 in]
              }
              event Value Change {
                # "REF Channels Value Change Event (Button Pressed)\n()"
                n129 = event-data() -> ()  [unwired: 1 in, 6 out]
                n130 = Bundle By Name(cluster=w292, "UI Config.Channels.Cfg_REF"="REF Channels") -> (w293:T65)
                n131 = call <vilib>:"Add State(s) to Queue__jki_lib_state_machine.vi"("State(s) in Front (\"\")"="Action: REF Channels\nAction: Command\nAction: Sampling Fs Output\nAction: Command", "State(s) in (\"\")"=w297) -> ("States Out"=w296:string)  [unwired: 13 in]
              }
              event Value Change {
                # "DAQ Config Value Change Event (Button Pressed)\n()"
                n132 = event-data() -> ()  [unwired: 1 in, 6 out]
                n133 = Bundle By Name(cluster=w299, "UI Config.DAQ.Simulation mode"="AI Simulation mode") -> (w300:T65)
                n134 = call <vilib>:"Add State(s) to Queue__jki_lib_state_machine.vi"("State(s) in Front (\"\")"="Action: AI Simulate Mode\nAction: Command", "State(s) in (\"\")"=w304) -> ("States Out"=w303:string)  [unwired: 13 in]
              }
              event Value Change {
                # "DAQ Config Value Change Event (Button Pressed)\n()"
                n135 = event-data() -> ()  [unwired: 1 in, 6 out]
                n136 = Bundle By Name(cluster=w306, "UI Config.Amplifers.Gain_AI"="Input Gain") -> (w307:T65)
                n137 = call <vilib>:"Add State(s) to Queue__jki_lib_state_machine.vi"("State(s) in Front (\"\")"="Action: Input Gain\nAction: Command", "State(s) in (\"\")"=w311) -> ("States Out"=w310:string)  [unwired: 13 in]
              }
              event Value Change {
                # "DAQ Config Value Change Event (Button Pressed)\n()"
                n138 = event-data() -> ()  [unwired: 1 in, 6 out]
                n139 = Bundle By Name(cluster=w313, "UI Config.Amplifers.Offset_AI"="Input Offsets") -> (w314:T65)
                n140 = call <vilib>:"Add State(s) to Queue__jki_lib_state_machine.vi"("State(s) in Front (\"\")"="Action: Offset\nAction: Command", "State(s) in (\"\")"=w318) -> ("States Out"=w317:string)  [unwired: 13 in]
              }
              event Value Change {
                # "DAQ Config Value Change Event (Button Pressed)\n()"
                n141 = event-data() -> ()  [unwired: 1 in, 6 out]
                n142 = Bundle By Name(cluster=w320, "UI Config.Amplifers.Gain_AO"="Output Gain") -> (w321:T65)
                n143 = call <vilib>:"Add State(s) to Queue__jki_lib_state_machine.vi"("State(s) in Front (\"\")"="Action: Output Gain\nAction: Command", "State(s) in (\"\")"=w325) -> ("States Out"=w324:string)  [unwired: 13 in]
              }
              event "AC Limit": Value Change {
                # "Limit Amplitudes Paramaters Change Event ()\n()"
                n144 = event-data() -> ()  [unwired: 1 in, 6 out]
                n145 = Bundle By Name(cluster=w327, "UI Config.Limit Amplitude.Limit (V)"="AC Limit") -> (w328:T65)
                n146 = call <vilib>:"Add State(s) to Queue__jki_lib_state_machine.vi"("State(s) in Front (\"\")"="Action: Limit Amplitude\nAction: Command", "State(s) in (\"\")"=w332) -> ("States Out"=w331:string)  [unwired: 13 in]
              }
              event "AC Limit All": Value Change {
                # "Limit Amplitudes Paramaters Change Event ()\n()"
                n147 = event-data() -> ()  [unwired: 1 in, 6 out]
                n148 = Unbundle By Name(w335) -> ("UI Config.Channels.Cfg_AO"=w334:T6)
                n149 = for {
                  tunnel: w334 -> [w343] mode=indexing
                  tunnel: [w341] -> w333 mode=indexing
                  n150 = Bundle By Name(cluster=w343, "Limit AC"=TRUE) -> (w341:T7)
                }
                n151 = Bundle By Name(cluster=w335, "UI Config.Channels.Cfg_AO"=w333) -> (w336:T65)
                n152 = local write "AO Channels"(w333) -> ()
                n153 = call <vilib>:"Add State(s) to Queue__jki_lib_state_machine.vi"("State(s) in Front (\"\")"="Action: AO Channels\nAction: Command", "State(s) in (\"\")"=w340) -> ("States Out"=w339:string)  [unwired: 13 in]
              }
              event "AC Limit None": Value Change {
                # "Limit Amplitudes Paramaters Change Event ()\n()"
                n154 = event-data() -> ()  [unwired: 1 in, 6 out]
                n155 = Unbundle By Name(w345) -> ("UI Config.Channels.Cfg_AO"=w347:T6)
                n156 = for {
                  tunnel: w347 -> [w354] mode=indexing
                  tunnel: [w352] -> w346 mode=indexing
                  n157 = Bundle By Name(cluster=w354, "Limit AC"=FALSE) -> (w352:T7)
                }
                n158 = Bundle By Name(cluster=w345, "UI Config.Channels.Cfg_AO"=w346) -> (w344:T65)
                n159 = local write "AO Channels"(w346) -> ()
                n160 = call <vilib>:"Add State(s) to Queue__jki_lib_state_machine.vi"("State(s) in Front (\"\")"="Action: AO Channels\nAction: Command", "State(s) in (\"\")"=w351) -> ("States Out"=w350:string)  [unwired: 13 in]
              }
              event "DC Limit All": Value Change {
                # "Limit Amplitudes Paramaters Change Event ()\n()"
                n161 = event-data() -> ()  [unwired: 1 in, 6 out]
                n162 = Unbundle By Name(w356) -> ("UI Config.Channels.Cfg_AO"=w358:T6)
                n163 = for {
                  tunnel: w358 -> [w365] mode=indexing
                  tunnel: [w363] -> w357 mode=indexing
                  n164 = Bundle By Name(cluster=w365, "Limit DC?"=TRUE ("Limit AC")) -> (w363:T7)
                }
                n165 = Bundle By Name(cluster=w356, "UI Config.Channels.Cfg_AO"=w357) -> (w355:T65)
                n166 = local write "AO Channels"(w357) -> ()
                n167 = call <vilib>:"Add State(s) to Queue__jki_lib_state_machine.vi"("State(s) in Front (\"\")"="Action: AO Channels\nAction: Command", "State(s) in (\"\")"=w362) -> ("States Out"=w361:string)  [unwired: 13 in]
              }
              event "DC Limit None": Value Change {
                # "Limit Amplitudes Paramaters Change Event ()\n()"
                n168 = event-data() -> ()  [unwired: 1 in, 6 out]
                n169 = Unbundle By Name(w367) -> ("UI Config.Channels.Cfg_AO"=w369:T6)
                n170 = for {
                  tunnel: w369 -> [w376] mode=indexing
                  tunnel: [w374] -> w368 mode=indexing
                  n171 = Bundle By Name(cluster=w376, "Limit DC?"=FALSE ("Limit AC")) -> (w374:T7)
                }
                n172 = Bundle By Name(cluster=w367, "UI Config.Channels.Cfg_AO"=w368) -> (w366:T65)
                n173 = local write "AO Channels"(w368) -> ()
                n174 = call <vilib>:"Add State(s) to Queue__jki_lib_state_machine.vi"("State(s) in Front (\"\")"="Action: AO Channels\nAction: Command", "State(s) in (\"\")"=w373) -> ("States Out"=w372:string)  [unwired: 13 in]
              }
              event "AO DC Limit": Value Change {
                # "Limit Amplitudes Paramaters Change Event ()\n()"
                n175 = event-data() -> ()  [unwired: 1 in, 6 out]
                n176 = Bundle By Name(cluster=w378, "UI Config.Limit DC.Limit (V)"="AO DC Limit") -> (w379:T65)
                n177 = call <vilib>:"Add State(s) to Queue__jki_lib_state_machine.vi"("State(s) in Front (\"\")"="Action: Limit DC\nAction: Command", "State(s) in (\"\")"=w383) -> ("States Out"=w382:string)  [unwired: 13 in]
              }
              event "Link f?", "f link (Hz)": Value Change {
                # "Link Frequencies Parameters Change Event ()\n()"
                n178 = event-data() -> ()  [unwired: 1 in, 6 out]
                n179 = Bundle By Name(cluster=w386, "UI Config.Link Frequencies.Link?"="Link f?", "UI Config.Link Frequencies.Frequency (Hz)"="f link (Hz)") -> (w387:T65)
                n180 = call <vilib>:"Add State(s) to Queue__jki_lib_state_machine.vi"("State(s) in Front (\"\")"="Action: Link Frequencies\nAction: Command", "State(s) in (\"\")"=w391) -> ("States Out"=w390:string)  [unwired: 13 in]
              }
              event "duty cycle (%)": Value Change {
                # "Link Frequencies Parameters Change Event ()\n()"
                n181 = event-data() -> ()  [unwired: 1 in, 6 out]
                n182 = Bundle By Name(cluster=w394, "UI Config.Function Option.Option?"=FALSE ("Function Option"), "UI Config.Function Option.Duty Cycle (%)"="duty cycle (%)") -> (w395:T65)
                n183 = call <vilib>:"Add State(s) to Queue__jki_lib_state_machine.vi"("State(s) in Front (\"\")"="Action: Duty Cycle\nAction: Command", "State(s) in (\"\")"=w399) -> ("States Out"=w398:string)  [unwired: 13 in]
              }
              event "Reset Phase": Value Change {
                # "Reset Phase Value Change Event (Button Pressed)\n()"
                n184 = event-data() -> ()  [unwired: 1 in, 6 out]
                n185 = local write "Reset Phase"(FALSE ("Help")) -> ()
                n186 = call <vilib>:"Add State(s) to Queue__jki_lib_state_machine.vi"("State(s) in Front (\"\")"="Action: Zero Phase\nAction: Command", "State(s) in (\"\")"=w405) -> ("States Out"=w404:string)  [unwired: 13 in]
              }
              event "Line", "Lowpass", "LP f (Hz)": Value Change {
                # "Prefilter Paramters Change Event ()\n()"
                n187 = event-data() -> ()  [unwired: 1 in, 6 out]
                n188 = Bundle By Name(cluster=w409, "UI Config.PreFilter.60 Hz"="Line", "UI Config.PreFilter.Low Pass"="Lowpass", "UI Config.PreFilter.Low Pass Cutoff (Hz)"="LP f (Hz)") -> (w410:T65)
                n189 = call <vilib>:"Add State(s) to Queue__jki_lib_state_machine.vi"("State(s) in Front (\"\")"="Action: PreFilter\nAction: Command", "State(s) in (\"\")"=w414) -> ("States Out"=w413:string)  [unwired: 13 in]
              }
              event "Sweep Time (s)", "Return to Start?", "Initial Wait (s)", "Sweep Pattern": Value Change {
                # "Sweep Parameters (Time, Wait, Return, Channels) Change Event ()\n()"
                n190 = event-data() -> ()  [unwired: 1 in, 6 out]
                n191 = Unbundle By Name(w417) -> ("UI Config.Sweep"=w422:T55)
                n192 = for {
                  tunnel: [w435] -> w415 mode=indexing
                  tunnel: "Sweep Pattern" -> [w434] mode=indexing
                  n193 = Unbundle By Name(w434) -> ("Channel"=w433:u16, "Sweep Pattern"=w432:dbl[])
                  n194 = Bundle By Name(cluster=T30 {"Channel"=1, "Table"=[]} ("setSweep_Table"), "Channel"=w433, "Table"=w432) -> (w435:T30)
                }
                n195 = Bundle By Name(cluster=w422, "sweepTime"="Sweep Time (s)", "initialWaitTime"="Initial Wait (s)", "returnToStart"="Return to Start?", "sweepChannels"="Sweep Channels") -> (w416:T55)
                n196 = call "Replace Sweep Waveforms.vi"("Channels New"=w415, "Sweep in"=w416) -> ("Sweep out"=w423:T55)  [unwired: 9 in]
                n197 = Bundle By Name(cluster=w417, "UI Config.Sweep"=w423) -> (w426:T65)
                n198 = call <vilib>:"Add State(s) to Queue__jki_lib_state_machine.vi"("State(s) in Front (\"\")"="Action: Sweep\nAction: Command", "State(s) in (\"\")"=w430) -> ("States Out"=w429:string)  [unwired: 13 in]
                "Sweep Timer (s)" <- 0.0 ("Sweep Timer (s)")
              }
              event "Remove Offset": Value Change {
                # "Remove Offset Value Change Event (Button Pressed)\n()"
                n199 = event-data() -> ()  [unwired: 1 in, 6 out]
                n200 = Format Into String(format string="Action: Offset Mode >> %s\nAction: Command", Offset_Mode--Enum."Remove" ("Offset Mode")) -> (resulting string=w437:string)  [unwired: 2 in, 1 out]
                n201 = call <vilib>:"Add State(s) to Queue__jki_lib_state_machine.vi"("State(s) in Front (\"\")"=w437, "State(s) in (\"\")"=w442) -> ("States Out"=w441:string)  [unwired: 13 in]
              }
              event "Measure Offset": Value Change {
                # "Measure Offset Value Change Event (Button Pressed)\n()"
                n202 = event-data() -> ()  [unwired: 1 in, 6 out]
                n203 = Format Into String(format string="Action: Offset Mode >> %s\nAction: Command", Offset_Mode--Enum."Measure" ("Offset Mode")) -> (resulting string=w444:string)  [unwired: 2 in, 1 out]
                n204 = call <vilib>:"Add State(s) to Queue__jki_lib_state_machine.vi"("State(s) in Front (\"\")"=w444, "State(s) in (\"\")"=w449) -> ("States Out"=w448:string)  [unwired: 13 in]
              }
              event "Get Calibration": Value Change {
                # "Get Calibration Value Change Event (Button Pressed)\n()"
                n205 = event-data() -> ()  [unwired: 1 in, 6 out]
                n206 = Format Into String(format string="Action: Calibrate >> %s\nAction: Command", PrivateEvents--DAQ.setCalibration."Check" ("setCalibration")) -> (resulting string=w451:string)  [unwired: 2 in, 1 out]
                n207 = call <vilib>:"Add State(s) to Queue__jki_lib_state_machine.vi"("State(s) in Front (\"\")"=w451, "State(s) in (\"\")"=w456) -> ("States Out"=w455:string)  [unwired: 13 in]
              }
              event "Self Calibrate": Value Change {
                # "Get Calibration Value Change Event (Button Pressed)\n()"
                n208 = event-data() -> ()  [unwired: 1 in, 6 out]
                n209 = Format Into String(format string="Action: Calibrate >> %s\nAction: Command", PrivateEvents--DAQ.setCalibration."Calibrate" ("setCalibration")) -> (resulting string=w457:string)  [unwired: 2 in, 1 out]
                n210 = call <vilib>:"Add State(s) to Queue__jki_lib_state_machine.vi"("State(s) in Front (\"\")"=w457, "State(s) in (\"\")"=w463) -> ("States Out"=w462:string)  [unwired: 13 in]
              }
              event "Show DAQ UI": Value Change {
                # "Get Calibration Value Change Event (Button Pressed)\n()"
                n211 = event-data() -> ()  [unwired: 1 in, 6 out]
                n212 = Format Into String(format string="Action: show DAQ UI >> %s\nAction: Command", "Show DAQ UI") -> (resulting string=w464:string)  [unwired: 2 in, 1 out]
                n213 = call <vilib>:"Add State(s) to Queue__jki_lib_state_machine.vi"("State(s) in Front (\"\")"=w464, "State(s) in (\"\")"=w470) -> ("States Out"=w469:string)  [unwired: 13 in]
              }
              event "Logging": Value Change {
                # "Get Calibration Value Change Event (Button Pressed)\n()"
                n214 = event-data() -> ("NewVal"=w471:bool)  [unwired: 1 in, 5 out]
                n215 = Format Into String(format string="Action: Logging >> %s\nAction: Command", w471) -> (resulting string=w472:string)  [unwired: 2 in, 1 out]
                n216 = call <vilib>:"Add State(s) to Queue__jki_lib_state_machine.vi"("State(s) in Front (\"\")"=w472, "State(s) in (\"\")"=w477) -> ("States Out"=w476:string)  [unwired: 13 in]
              }
              event "....................Graph and UI....................": Value Change {
                # "Do not put any code in this frame.\n(it is a separator no-op)"
                n217 = event-data() -> ()  [unwired: 1 in, 6 out]
                n218 = call <vilib>:"Add State(s) to Queue__jki_lib_state_machine.vi"("State(s) in (\"\")"=w481) -> ("States Out"=w480:string)  [unwired: 14 in]
              }
              event Value Change {
                # "Display Value Change Event (Button Pressed)\n()"
                n219 = event-data() -> ()  [unwired: 1 in, 6 out]
                n220 = call <vilib>:"Add State(s) to Queue__jki_lib_state_machine.vi"("State(s) in Front (\"\")"="UI: Defer Panel Updates >> TRUE\nUI: Update Lockin Graph Labels\nUI: Defer Panel Updates >> FALSE", "State(s) in (\"\")"=w486) -> ("States Out"=w485:string)  [unwired: 13 in]
              }
              event "PS Display": Value Change {
                w489 = "UI: Defer Panel Updates >> TRUE\nUI: Update PS Graph Labels\nUI: Update PS Graph Legend\nUI: Defer Panel Updates >> FALSE"  # UI: Defer Panel Updates >> TRUE UI: Update PS Graph Labels UI: Update PS Graph Legend UI: Defer Panel Updates >> FALSE
                # "Display Value Change Event (Button Pressed)\n()"
                n221 = event-data() -> ()  [unwired: 1 in, 6 out]
                n222 = call <vilib>:"Add State(s) to Queue__jki_lib_state_machine.vi"("State(s) in Front (\"\")"=w489, "State(s) in (\"\")"=w491) -> ("States Out"=w490:string)  [unwired: 13 in]
              }
              event "AI Graph": Plot Attribute Change {
                # "Display Value Change Event (Button Pressed)\n()"
                n223 = event-data() -> ()  [unwired: 1 in, 8 out]
                n224 = call <vilib>:"Add State(s) to Queue__jki_lib_state_machine.vi"("State(s) in Front (\"\")"="UI: Defer Panel Updates >> TRUE\nUI: Sync AI Plot Visibility\nUI: Defer Panel Updates >> FALSE", "State(s) in (\"\")"=w496) -> ("States Out"=w495:string)  [unwired: 13 in]
              }
              event "AO Graph": Value Change {
                # "Display Value Change Event (Button Pressed)\n()"
                n225 = event-data() -> ()  [unwired: 1 in, 6 out]
                n226 = call <vilib>:"Add State(s) to Queue__jki_lib_state_machine.vi"("State(s) in Front (\"\")"="UI: Defer Panel Updates >> TRUE\nUI: Sync AO Plot Visibility\nUI: Defer Panel Updates >> FALSE", "State(s) in (\"\")"=w501) -> ("States Out"=w500:string)  [unwired: 13 in]
              }
              event "Lockin 1": Plot Attribute Change {
                # "Display Value Change Event (Button Pressed)\n()"
                n227 = event-data() -> ()  [unwired: 1 in, 8 out]
                n228 = call <vilib>:"Add State(s) to Queue__jki_lib_state_machine.vi"("State(s) in Front (\"\")"="UI: Defer Panel Updates >> TRUE\nUI: Sync Lockin Plot Visibility\nUI: Defer Panel Updates >> FALSE", "State(s) in (\"\")"=w506) -> ("States Out"=w505:string)  [unwired: 13 in]
              }
              event "Lockin 1", "Lockin 2": Shortcut Menu Selection? (App) {
                # "Display Value Change Event (Button Pressed)\n()"
                n229 = event-data() -> ("ItemTag"=w509:string)  [unwired: 1 in]
                n230 = Equal?(x="APP_SC_CLEAR_GRAPH", y=w509) -> (x = y?=w507:bool)
                n231 = Bundle By Name(cluster=w510, "clear lockin charts"=w507) -> (w511:T65)
                n232 = event-data("Discard?"=w507) -> ()  [unwired: 1 in, 1 out]
                n233 = call <vilib>:"Add State(s) to Queue__jki_lib_state_machine.vi"("State(s) in Front (\"\")"="", "State(s) in (\"\")"=w515) -> ("States Out"=w514:string)  [unwired: 13 in]
              }
              event "Disable All", "Enable All": Value Change {
                # "AI Disable or Enable Change Event (Button Pressed)\n()"
                n234 = event-data() -> ("CtlRef"=w518:refnum<vi>)  [unwired: 1 in, 5 out]
                n235 = control-ref of="Disable All"() -> (w520:refnum<vi>)
                n236 = Equal?(x=w518, y=w520) -> (x = y?=w519:bool)
                n237 = call "Stall Data Flow.vim"("value in"=w519, "milliseconds to wait"=u32 50) -> ("value out"=w517:bool)  [unwired: 1 out]
                n238 = Select(t="Disable" ("Arguments (\"\")"), s=w519, f="ALL 1" ("Arguments (\"\")")) -> (s? t:f=w521:string)
                n239 = flat-sequence {
                  tunnel: w517 -> [_]
                  frame #0 {
                    n240 = local write "Enable All"(FALSE ("Disable all AI Ref")) -> ()
                    n241 = local write "Disable All"(FALSE ("Disable all AI Ref")) -> ()
                  }
                }
                n242 = call <vilib>:"Build State String with Arguments__JKI_lib_State_Machine.vi"("Arguments (\"\")"=w521, "State"="UI: Update AI REF Channels") -> ("State with Arguments"=w526:string)  [unwired: 4 in]
                n243 = call <vilib>:"Add State(s) to Queue__jki_lib_state_machine.vi"("State(s) in Front (\"\")"=w526, "State(s) at Back (\"\")"="Action: AI Channels\nAction: Command") -> ("States Out"=w524:string)  [unwired: 13 in]
                n244 = call <vilib>:"Add State(s) to Queue__jki_lib_state_machine.vi"("State(s) in Front (\"\")"=w524, "State(s) in (\"\")"=w531) -> ("States Out"=w530:string)  [unwired: 13 in]
              }
              event "AI Graph All", "AI Graph None": Value Change {
                # "AI Graph All/None Value Change Event (Button Pressed)\n()"
                n245 = event-data() -> ("CtlRef"=w541:refnum<vi>)  [unwired: 1 in, 5 out]
                n246 = control-ref of="AI Graph All"() -> (w540:refnum<vi>)
                n247 = Equal?(x=w541, y=w540) -> (x = y?=w537:bool)
                n248 = Select(t="ALL" ("Arguments (\"\")"), s=w537, f="NONE" ("Arguments (\"\")")) -> (s? t:f=w535:string)
                n249 = Format Into String(format string="UI: Defer Panel Updates >> TRUE\nUI: AI Graphs Plot Visibility >> %s\nUI: Defer Panel Updates >> FALSE", w535) -> (resulting string=w534:string)  [unwired: 2 in, 1 out]
                n250 = call <vilib>:"Add State(s) to Queue__jki_lib_state_machine.vi"("State(s) in Front (\"\")"=w534, "State(s) in (\"\")"=w545) -> ("States Out"=w544:string)  [unwired: 13 in]
              }
              event "AO Graph All", "AO Graph None": Value Change {
                # "AO Graph All Value Change Event (Button Pressed)\n()"
                n251 = event-data() -> ("CtlRef"=w553:refnum<vi>)  [unwired: 1 in]
                n252 = control-ref of="AO Graph All"() -> (w552:refnum<vi>)
                n253 = Equal?(x=w553, y=w552) -> (x = y?=w551:bool)
                n254 = Select(t="ALL" ("Arguments (\"\")"), s=w551, f="NONE" ("Arguments (\"\")")) -> (s? t:f=w547:string)
                n255 = Format Into String(format string="UI: Defer Panel Updates >> TRUE\nUI: AO Graphs Plot Visibility >> %s\nUI: Defer Panel Updates >> FALSE", w547) -> (resulting string=w546:string)  [unwired: 2 in, 1 out]
                n256 = call <vilib>:"Add State(s) to Queue__jki_lib_state_machine.vi"("State(s) in Front (\"\")"=w546, "State(s) in (\"\")"=w557) -> ("States Out"=w556:string)  [unwired: 13 in]
              }
              event "REF Graph All", "REF Graph None": Value Change {
                # "AO Graph All Value Change Event (Button Pressed)\n()"
                n257 = event-data() -> ("CtlRef"=w565:refnum<vi>)  [unwired: 1 in]
                n258 = control-ref of="REF Graph All"() -> (w564:refnum<vi>)
                n259 = Equal?(x=w565, y=w564) -> (x = y?=w563:bool)
                n260 = Select(t="ALL" ("Arguments (\"\")"), s=w563, f="NONE" ("Arguments (\"\")")) -> (s? t:f=w559:string)
                n261 = Format Into String(format string="UI: Defer Panel Updates >> TRUE\nUI: REF Graphs Plot Visibility >> %s\nUI: Defer Panel Updates >> FALSE", w559) -> (resulting string=w558:string)  [unwired: 2 in, 1 out]
                n262 = call <vilib>:"Add State(s) to Queue__jki_lib_state_machine.vi"("State(s) in Front (\"\")"=w558, "State(s) in (\"\")"=w569) -> ("States Out"=w568:string)  [unwired: 13 in]
              }
              event "Lockin Graph All", "Lockin Graph None", "Lockin Graph All 2", "Lockin Graph None 2": Value Change {
                # "Lockin Graph All Value Change Event (Button Pressed)\n()"
                n263 = event-data() -> ("CtlRef"=w573:refnum<vi>)  [unwired: 1 in]
                n264 = control-ref of="Lockin Graph All"() -> (w580:refnum<vi>)
                n265 = control-ref of="Lockin Graph All 2"() -> (w574:refnum<vi>)
                n266 = Equal?(x=w573, y=w580) -> (x = y?=w571:bool)
                n267 = Equal?(x=w573, y=w574) -> (x = y?=w572:bool)
                n268 = Or(x=w571, y=w572) -> (x .or. y?=w570:bool)
                n269 = Select(t="ALL" ("Arguments (\"\")"), s=w570, f="NONE" ("Arguments (\"\")")) -> (s? t:f=w576:string)
                n270 = Format Into String(format string="UI: Defer Panel Updates >> TRUE\nUI: Lockin Graphs Plot Visibility >> %s\nUI: Defer Panel Updates >> FALSE", w576) -> (resulting string=w575:string)  [unwired: 2 in, 1 out]
                n271 = call <vilib>:"Add State(s) to Queue__jki_lib_state_machine.vi"("State(s) in Front (\"\")"=w575, "State(s) in (\"\")"=w584) -> ("States Out"=w583:string)  [unwired: 13 in]
              }
              event "X/R Range", "Y/Theta Range", "XY Range": Value Change {
                # "X/R Range, Y/Theta Range, XY Range Value Change Event\n(this executes UI: Update Lockin Graph Range)"
                n272 = event-data() -> ()  [unwired: 1 in, 6 out]
                n273 = call <vilib>:"Add State(s) to Queue__jki_lib_state_machine.vi"("State(s) in Front (\"\")"="UI: Defer Panel Updates >> TRUE\nUI: Update Lockin Graph Range\nUI: Defer Panel Updates >> FALSE", "State(s) in (\"\")"=w589) -> ("States Out"=w588:string)  [unwired: 13 in]
              }
              event "Output": Value Change {
                # "Y Axis (Output) Value Change Event\n(this executes UI: Show Hide AO Waveform Graphs)"
                n274 = event-data() -> ()  [unwired: 1 in, 6 out]
                n275 = call <vilib>:"Add State(s) to Queue__jki_lib_state_machine.vi"("State(s) in Front (\"\")"="UI: Defer Panel Updates >> TRUE\nUI: Show Hide AO Waveform Graphs\nUI: Defer Panel Updates >> FALSE", "State(s) in (\"\")"=w594) -> ("States Out"=w593:string)  [unwired: 13 in]
              }
              event "X Scale": Value Change {
                # "X Axis Value Change Event\n(this executes UI: Update Waveform Graph Labels)"
                n276 = event-data() -> ()  [unwired: 1 in, 6 out]
                n277 = call <vilib>:"Add State(s) to Queue__jki_lib_state_machine.vi"("State(s) in Front (\"\")"="UI: Defer Panel Updates >> TRUE\nUI: Update Waveform Graph Labels\nUI: Defer Panel Updates >> FALSE", "State(s) in (\"\")"=w599) -> ("States Out"=w598:string)  [unwired: 13 in]
              }
              event "export mode": Value Change {
                # "PS export mode Value Change Event\n(this executes UI: Update PS Graph Labels)"
                n278 = event-data() -> ()  [unwired: 1 in, 6 out]
                n279 = call <vilib>:"Add State(s) to Queue__jki_lib_state_machine.vi"("State(s) in Front (\"\")"="UI: Defer Panel Updates >> TRUE\nUI: Update PS Graph Labels\nUI: Defer Panel Updates >> FALSE", "State(s) in (\"\")"=w604) -> ("States Out"=w603:string)  [unwired: 13 in]
              }
              event "....................Dynamic Events....................": Value Change {
                # "Do not put any code in this frame.\n(it is a separator no-op)"
                n280 = event-data() -> ()  [unwired: 1 in, 6 out]
                n281 = call <vilib>:"Add State(s) to Queue__jki_lib_state_machine.vi"("State(s) in (\"\")"=w608) -> ("States Out"=w607:string)  [unwired: 14 in]
              }
              event User Event {
                # "<SMO Protected Events.StopProcesses>: User Event"
                n282 = event-data() -> ()  [unwired: 1 in, 5 out]
                n283 = call <vilib>:"Add State(s) to Queue__jki_lib_state_machine.vi"("State(s) in Front (\"\")"="Macro: Exit", "State(s) in (\"\")"=w613) -> ("States Out"=w612:string)  [unwired: 13 in]
              }
              event User Event {
                # "<SMO Protected Events.AbortProcesses>: User Event"
                # "On Abort, no nice macro exit, but exit right away"
                n284 = event-data() -> ()  [unwired: 1 in, 5 out]
                n285 = call <vilib>:"Add State(s) to Queue__jki_lib_state_machine.vi"("State(s) in Front (\"\")"="Exit", "State(s) in (\"\")"=w618) -> ("States Out"=w617:string)  [unwired: 13 in]
              }
              event User Event {
                # "<SMO.UI Public Events.UI Hidden>: User Event"
                n286 = event-data() -> ()  [unwired: 1 in, 5 out]
                n287 = call <vilib>:"Add State(s) to Queue__jki_lib_state_machine.vi"("State(s) in (\"\")"=w622) -> ("States Out"=w621:string)  [unwired: 14 in]
              }
              event User Event {
                # "<DAQ SMO Public Events.Error>: User Event"
                n288 = event-data() -> ("code"=w626:i32, "source"=w625:string)  [unwired: 1 in]
                n289 = Format Into String(format string="%d %s", w626, w625) -> (resulting string=w624:string)  [unwired: 2 in, 1 out]
                n290 = call <userlib>:"State History.vi"("Current State"=w624) -> ("History"=→"Status":string)  [unwired: 9 in, 1 out]
                n291 = call <vilib>:"Add State(s) to Queue__jki_lib_state_machine.vi"("State(s) in (\"\")"=w631) -> ("States Out"=w630:string)  [unwired: 14 in]
              }
              event User Event {
                # "<DAQ SMO Public Events.State>: User Event"
                n292 = event-data() -> ("SMO State"=w632:T67)  [unwired: 1 in, 4 out]
                n293 = case shown="\"Started\"" w632 {
                  tunnel: ["UI: Enable Buttons" ("State Queue") "//DONE: Stop\n//DONE: Start" ("State Queue")] -> w633
                  frame "Started" {
                  }
                  frame Default {
                  }
                }
                n294 = call <vilib>:"Add State(s) to Queue__jki_lib_state_machine.vi"("State(s) in Front (\"\")"=w633, "State(s) in (\"\")"=w637) -> ("States Out"=w636:string)  [unwired: 13 in]
              }
              event User Event {
                # "<DAQ Public Events.getDAQState>: User Event"
                n295 = event-data() -> ("status"=w644:T33)  [unwired: 1 in, 4 out]
                n296 = Get Date/Time In Seconds() -> (seconds since 1Jan1904=w647:timestamp)
                n297 = Format Into String(w644) -> (resulting string=→"Inst.DAQ State":string)  [unwired: 3 in, 1 out]
                n298 = To Double Precision Float(number=w647) -> (double precision float=→"State Time":dbl)
                n299 = case shown="\"sweeping\"" w644 {
                  frame Default {
                  }
                  frame "sweeping" {
                    n300 = call <userlib>:"MGI Milliseconds Since Last Reset.vi"("Reset (F)"=TRUE) -> ()  [unwired: 5 in, 2 out]
                  }
                }
                n301 = Bundle By Name(cluster=w645, "DAQ state"=w644) -> (w650:T65)
                n302 = Format Into String(w644) -> (resulting string=w643:string)  [unwired: 3 in, 1 out]
                n303 = call <vilib>:"Build State String with Arguments__JKI_lib_State_Machine.vi"("Arguments (\"\")"=w643, "State"="UI: Update Status") -> ("State with Arguments"=w642:string)  [unwired: 4 in]
                n304 = call <vilib>:"Add State(s) to Queue__jki_lib_state_machine.vi"("State(s) in Front (\"\")"=w642, "State(s) in (\"\")"="UI: Defer Panel Updates >> TRUE\nUI: Update Booleans\nUI: Defer Panel Updates >> FALSE" ("State")) -> ("States Out"=w641:string)  [unwired: 13 in]
                n305 = call <vilib>:"Add State(s) to Queue__jki_lib_state_machine.vi"("State(s) in Front (\"\")"=w641, "State(s) in (\"\")"=w653) -> ("States Out"=w652:string)  [unwired: 13 in]
              }
              event User Event {
                # "== T when \"start\" button pressed"
                # "<DAQ Public Events.getWaveforms>: User Event"
                n306 = event-data() -> ("AO"=w660:waveform(dbl)[], "AI"=w659:waveform(dbl)[], "REF_X"=w658:waveform(dbl)[], "REF_Y"=w657:waveform(dbl)[])  [unwired: 1 in, 4 out]
                n307 = Unbundle By Name(w662) -> ("update waveform graphs"=w665:bool)
                n308 = Bundle By Name(cluster=w662, "update waveform graphs"=FALSE ("update graphs"), "getAll.Waveforms.AO"=w660, "getAll.Waveforms.AI"=w659, "getAll.Waveforms.REF_X"=w658, "getAll.Waveforms.REF_Y"=w657) -> (w661:T65)
                n309 = Select(t="Macro: Initialize Waveform Graphs", s=w665, f="Macro: Update Waveform Graphs") -> (s? t:f=w655:string)
                n310 = call <vilib>:"Add State(s) to Queue__jki_lib_state_machine.vi"("State(s) in Front (\"\")"=w655, "State(s) in (\"\")"=w668) -> ("States Out"=w667:string)  [unwired: 13 in]
              }
              event User Event {
                # "== T when \"start\" button pressed"
                # "<DAQ Public Events.getResults>: User Event"
                n311 = event-data() -> ("Results"=w678:T59)  [unwired: 1 in, 4 out]
                n312 = Unbundle By Name(w674) -> ("update lockin graphs"=w673:bool)
                n313 = Bundle By Name(cluster=w674, "update lockin graphs"=FALSE, "getAll.Results"=w678) -> (w679:T65)
                n314 = Select(t="Macro: Initialize Lockin Graphs", s=w673, f="") -> (s? t:f=w669:string)
                n315 = call <vilib>:"Add State(s) to Queue__jki_lib_state_machine.vi"("State(s) in Front (\"\")"=w669, "State(s) at Back (\"\")"="Macro: Update Lockin Graphs") -> ("States Out"=w672:string)  [unwired: 13 in]
                n316 = call <vilib>:"Add State(s) to Queue__jki_lib_state_machine.vi"("State(s) in Front (\"\")"=w672, "State(s) in (\"\")"=w681) -> ("States Out"=w680:string)  [unwired: 13 in]
              }
              event User Event {
                # "<DAQ Public Events.getCalibration>: User Event"
                n317 = event-data() -> ("Calibration"=w682:T23)  [unwired: 1 in, 4 out]
                "Cal Info" <- w682
                n318 = Bundle By Name(cluster=w683, "UI Config.DAQ.Calibration"=w682) -> (w684:T65)
                n319 = call <vilib>:"Add State(s) to Queue__jki_lib_state_machine.vi"("State(s) in Front (\"\")"="", "State(s) in (\"\")"=w688) -> ("States Out"=w687:string)  [unwired: 13 in]
              }
              event User Event {
                # "<DAQ Public Events.getAOChannels>: User Event"
                n320 = event-data() -> ("Channels: AO"=w690:T6)  [unwired: 1 in, 4 out]
                n321 = local write "AO Channels"(w690) -> ()
                n322 = Bundle By Name(cluster=w691, "UI Config.Channels.Cfg_AO"=w690) -> (w692:T65)
                n323 = call <vilib>:"Add State(s) to Queue__jki_lib_state_machine.vi"("State(s) in Front (\"\")"="" ("f"), "State(s) in (\"\")"=w695) -> ("States Out"=w694:string)  [unwired: 13 in]
              }
              event User Event {
                # "<DAQ Public Events.getAIChannels>: User Event"
                n324 = event-data() -> ("Channels.AI"=w698:T4)  [unwired: 1 in, 4 out]
                n325 = Bundle By Name(cluster=w697, "UI Config.Channels.Cfg_AI"=w698) -> (w699:T65)
                n326 = local write "AI Channels"(w698) -> ()
                n327 = call <vilib>:"Add State(s) to Queue__jki_lib_state_machine.vi"("State(s) in Front (\"\")"="" ("State(s) in Front (\"\")"), "State(s) in (\"\")"=w702) -> ("States Out"=w701:string)  [unwired: 13 in]
              }
              event User Event {
                # "<DAQ Public Events.getREFChannels>: User Event"
                n328 = event-data() -> ("Channels: REF"=w704:T2)  [unwired: 1 in, 4 out]
                n329 = Bundle By Name(cluster=w705, "UI Config.Channels.Cfg_REF"=w704) -> (w706:T65)
                n330 = local write "REF Channels"(w704) -> ()
                n331 = call <vilib>:"Add State(s) to Queue__jki_lib_state_machine.vi"("State(s) in Front (\"\")"="UI: Defer Panel Updates >> TRUE\nUI: Update Channel Ring\nUI: Update AI REF Channel Ring\nUI: Remove Unused References\nUI: Defer Panel Updates >> FALSE", "State(s) in (\"\")"=w709) -> ("States Out"=w708:string)  [unwired: 13 in]
              }
              event User Event {
                # "<DAQ Public Events.getSweepChannels>: User Event"
                n332 = event-data() -> ("Channels.Sweep"=w710:T55)  [unwired: 1 in, 4 out]
                n333 = Bundle By Name(cluster=w711, "UI Config.Sweep"=w710) -> (w712:T65)
                n334 = call <vilib>:"Add State(s) to Queue__jki_lib_state_machine.vi"("State(s) in Front (\"\")"="UI: Update Sweep Config", "State(s) in (\"\")"=w716) -> ("States Out"=w715:string)  [unwired: 13 in]
              }
              event User Event {
                # "<DAQ Public Events.getSweepWaveforms>: User Event"
                n335 = event-data() -> ("AO"=w729:waveform(dbl)[], "AI"=w728:waveform(dbl)[], "X"=w727:waveform(dbl)[], "Y"=w726:waveform(dbl)[])  [unwired: 1 in, 4 out]
                n336 = Bundle By Name(cluster=w725, "getAll.SweepWaveforms.AO"=w729, "getAll.SweepWaveforms.AI"=w728, "getAll.SweepWaveforms.X"=w727, "getAll.SweepWaveforms.Y"=w726) -> (w730:T65)
                n337 = Unbundle By Name(w725) -> ("DAQ state"=w717:T33)
                n338 = Get Date/Time In Seconds() -> (seconds since 1Jan1904=w719:timestamp)
                n339 = To Double Precision Float(number=w719) -> (double precision float=→"Sweep Time":dbl)
                n340 = Equal?(x=Status--enum."idle" ("getAll.DAQ state"), y=w717) -> (x = y?=w722:bool)
                n341 = Format Into String(w717) -> ()  [unwired: 3 in, 2 out]
                n342 = Select(t="Macro: Initialize Waveform Graphs", s=w722, f="UI: Update Sweep Graphs") -> (s? t:f=w720:string)
                n343 = call <vilib>:"Add State(s) to Queue__jki_lib_state_machine.vi"("State(s) in Front (\"\")"=w720, "State(s) in (\"\")"=w733) -> ("States Out"=w732:string)  [unwired: 13 in]
              }
              event User Event {
                # "<DAQ Public Events.getDAQconfig>: User Event"
                n344 = event-data() -> ("New Ch []"=w734:T9)  [unwired: 1 in]
                n345 = Bundle By Name(cluster=w735, "UI Config.DAQ.Configuration"=w734) -> (w736:T65)
                n346 = local write "DAQ Config"(w734) -> ()
                n347 = call <vilib>:"Add State(s) to Queue__jki_lib_state_machine.vi"("State(s) in Front (\"\")"="UI: Defer Panel Updates >> TRUE\nUI: Update AI Waveform Graphs Legends\nUI: Update AI Waveform Graphs Colors\nUI: Update AO Waveform Graphs Legends\nUI: Update AO Waveform Graphs Colors\nUI: Defer Panel Updates >> FALSE", "State(s) in (\"\")"=w740) -> ("States Out"=w739:string)  [unwired: 13 in]
              }
              event User Event {
                # "<DAQ Public Events.getSampling>: User Event"
                n348 = event-data() -> ("Sampling"=w758:T48)  [unwired: 1 in]
                n349 = Unbundle By Name(w758) -> ("Sampling.Fs"=w751:dbl, "Sampling.#s"=w753:i32, "Fs.Output"=w745:dbl)
                "Actual Fs (S/s)" <- w751
                "Actual #s (S)" <- w753
                n350 = Bundle By Name(cluster=w759, "UI Config.DAQ.cfg.Sampling"=w758) -> (w750:T65)
                n351 = local read "#s (S) (buffer)"() -> (w757:i32)
                n352 = local read "Fs (S/s) (buffer)"() -> (w755:dbl)
                n353 = Equal To 0?(x=w757) -> (x = 0?=w754:bool)
                n354 = call <userlib>:"MGI Approximately Equal.vi"("Numeric 2"=0.0, "Numeric 1"=w755) -> ("approx = ?"=w752:bool)
                n355 = Unbundle By Name(w750) -> ("UI Config.Channels.Cfg_REF"=w749:T2, "UI Config.DAQ.cfg.Sampling.Sampling"=w748:T49)
                n356 = case shown="True" w754 {
                  tunnel: w753 -> [_ w764]
                  frame False {
                  }
                  frame True {
                    n357 = local write "#s (S) (buffer)"(w764) -> ()
                  }
                }
                n358 = case shown="True" w752 {
                  tunnel: w751 -> [_ w763]
                  frame False {
                  }
                  frame True {
                    n359 = local write "Fs (S/s) (buffer)"(w763) -> ()
                  }
                }
                n360 = call "Calculate Output Sampling.vi"("sampling info"=w748, "Cfg_REF"=w749) -> ("Filter Parameters"=w747:T68)  [unwired: 8 in, 1 out]
                n361 = Unbundle By Name(w747) -> ("Fs.Output (S/s)"=w746:dbl)
                n362 = call <userlib>:"MGI Approximately Equal.vi"("Numeric 2"=w745, "Numeric 1"=w746) -> ("approx = ?"=w744:bool)
                n363 = Select(t="", s=w744, f="Action: Sampling Fs Output\nAction: Command") -> (s? t:f=w741:string)
                n364 = call <vilib>:"Add State(s) to Queue__jki_lib_state_machine.vi"("State(s) in Front (\"\")"=w741, "State(s) in (\"\")"=w762) -> ("States Out"=w761:string)  [unwired: 13 in]
              }
              event User Event {
                # "<DAQ Public Events.getInputGain>: User Event"
                n365 = event-data() -> ("Input Gain"=w765:T17)  [unwired: 1 in, 4 out]
                n366 = Bundle By Name(cluster=w766, "UI Config.Amplifers.Gain_AI"=w765) -> (w767:T65)
                n367 = local write "Input Gain"(w765) -> ()
                n368 = call <vilib>:"Add State(s) to Queue__jki_lib_state_machine.vi"("State(s) in Front (\"\")"="", "State(s) in (\"\")"=w771) -> ("States Out"=w770:string)  [unwired: 13 in]
              }
              event User Event {
                # "<DAQ Public Events.getOutputGain>: User Event"
                n369 = event-data() -> ("Output Gain"=w772:T17)  [unwired: 1 in, 4 out]
                n370 = Bundle By Name(cluster=w773, "UI Config.Amplifers.Gain_AO"=w772) -> (w774:T65)
                n371 = local write "Output Gain"(w772) -> ()
                n372 = call <vilib>:"Add State(s) to Queue__jki_lib_state_machine.vi"("State(s) in Front (\"\")"="", "State(s) in (\"\")"=w778) -> ("States Out"=w777:string)  [unwired: 13 in]
              }
              event User Event {
                # "<DAQ Public Events.getInputOffset>: User Event"
                n373 = event-data() -> ("Input Offset"=w779:T17)  [unwired: 1 in, 4 out]
                n374 = Bundle By Name(cluster=w780, "UI Config.Amplifers.Offset_AI"=w779) -> (w781:T65)
                n375 = local write "Input Offsets"(w779) -> ()
                n376 = call <vilib>:"Add State(s) to Queue__jki_lib_state_machine.vi"("State(s) in Front (\"\")"="", "State(s) in (\"\")"=w785) -> ("States Out"=w784:string)  [unwired: 13 in]
              }
            }
          }
          frame "---------- Core ----------" {
            # "Do not put any code in this frame.\n(it is a separator no-op)"
            n377 = call <vilib>:"Add State(s) to Queue__jki_lib_state_machine.vi"("State(s) in (\"\")"=w790) -> ("States Out"=w789:string)  [unwired: 14 in]
          }
          frame Default {
            w801 = 42 items=["No error", "Argument error", "Memory is full", "Out of zone", "End of file", "File already open", "Generic file I/O error", "File not found", "File permission error", "Disk is full", "Duplicate path", "Too many files open", "System feature not enabled", "Resource file not found", "Cannot add resource", "Resource not found", "Image not found", "Image memory error", "Pen does not exist", "Config type invalid", "Config token not found", "Config parse error", "Config memory error", "Bad external code format", "Bad external code offset", "External code not present", "Null window", "Destroy window error", "Null menu", "Print aborted", "Bad print record", "Print driver error", "Windows error during printing", "Memory error during printing", "Print dialog error", "Generic print error", "Invalid device refnum", "Device not found", "Device parameter error", "Device unit error", "Cannot open device", "Device call aborted", "Generic error", "Cancelled by user", "Object ID too low", "Object ID too high", "Object not in heap", "Unknown heap", "Unknown object (invalid DefProc)", "Unknown object (DefProc not in table)", "Message out of range", "Invalid (null) method", "Unknown message", "Manager call not supported", "Bad address", "Network operation in progress", "Network operation timed out", "Connection is busy", "Network attribute not supported", "Network error", "Address in use", "System out of memory", "Connection aborted", "Connection refused", "Not connected", "Already connected", "Connection closed", "Initialization error (interapplication manager)", "Bad occurrence", "Wait on unbound occurrence handler", "Occurrence queue overflow", "Datalog type conflict", "Unused", "Unrecognized type (interapplication manager)", "Memory corrupt", "Failed to make temporary DLL", "Old CIN version", "Drag socket not found", "Failed to load drop-object", "Failed to register OLE object", "Failed to release OLE object", "Format specifier type mismatch", "Unknown format specifier", "Too few format specifiers", "Too many format specifiers", "Scan failed", "Newer CIN version", "Error converting to variant", "Runtime menu error", "Password tampered", "Variant attribute not found", "Incompatible variant data type", "Event data is not available", "Event Store is not present", "Occurrence is not found", "Event Queue is not created", "Event info is not available", "Refnum passed is NULL", "Error retrieving Class GUID", "Error retrieving CoClass GUID", "Error retrieving TypeLib GUID.", "Bad built application magic bytes.", "Specific driver is different from the specific driver associated with the Logical Name.", "There is no session opened to the class driver.", "Max Error", "MAX - Error with config objects", "MAX - Error loading configuration", "MAX - Group not supported"]
            # "Current State"
            # "Do not delete, rename, or modify this frame.\n(this is used to capture unhandled states and typos)"
            # "Handle mistyped state name (developer tool)"
            n378 = Format Into String(format string="Software Exception: Unhandled State \"%s\"." ("message"), error in=w797, w792) -> (resulting string=w800:string, error out=w799:errorcluster)  [unwired: 1 in]
            n379 = call <vilib>:"Error Cluster From Error Code.vi"("show call chain? (False)"=TRUE, "error in (no error)"=w799, "error message (\"\")"=w800, "error code (0)"=w801) -> ("error out"=w798:errorcluster)  [unwired: 5 in]
            n380 = call <vilib>:"Add State(s) to Queue__jki_lib_state_machine.vi"("State(s) in (\"\")"=w796) -> ("States Out"=w795:string)  [unwired: 14 in]
          }
          frame "Initialize Core Data" {
            # "Do not delete, rename, or modify this frame.\n(this is used to determine panel behavior on exit)"
            # "originally closed?"
            # "exe?"
            # "If panel starts closed or is an EXE, then close it when we exit"
            n381 = property class="VI"() -> ("Front Panel.Open"=w811:bool)  [unwired: 2 in, 2 out]
            n382 = property class="App"() -> ("App.Kind"=w810:T34)  [unwired: 2 in, 2 out]
            n383 = control-ref of="Current VI Reference"() -> (w804:refnum<vi>)
            n384 = Not(x=w811) -> (.not. x?=w808:bool)
            n385 = Equal?(x=w810, y=T34."Run Time System" ("Application:Kind")) -> (x = y?=w807:bool)
            n386 = Or(x=w808, y=w807) -> (x .or. y?=w805:bool)
            n387 = Bundle By Name(cluster=w806, "Core.Current VI Reference"=w804, "Core.Close Panel on Exit?"=w805) -> (w813:T65)
            n388 = call <vilib>:"Add State(s) to Queue__jki_lib_state_machine.vi"("State(s) in (\"\")"=w815) -> ("States Out"=w814:string)  [unwired: 14 in]
          }
          frame "Error Handler" {
            w823 = errorcluster {"status"=FALSE, "code"=0, "source"=""}  # No error
            # "There was an error while handling the error.\nStop the process. This error can only occur if public events references are invalid or if the state machine object is destroyed."
            # "Overwrite this method to handle errors and pass to parent if not handled. Parent will fire a public event if the error is not handled up the chain of classes."
            # "Handle any errors here.\nYou can also output any states to clean-up after errors occur"
            n389 = Unbundle By Name(w821) -> ("SMO"=w827:refnum<class "Instrument UI.Lockin.lvclass">)
            n390 = call-dynamic "Handle Error.vi"("Stop on Unhandled Error (T)"=FALSE, "error in"=w826, "SMO"=w827) -> ("handling error"=w824:errorcluster, "Unhandled error"=w822:errorcluster)  [unwired: 6 in, 1 out]
            n391 = Bundle By Name(cluster=w821, "Core.Last Error.remaining states"=w818, "Core.Last Error.error"=w822) -> (w820:T65)
            n392 = Select(t="Exit", s=w824, f="Macro: Post Error Handling") -> (s? t:f=w817:string)
          }
          frame "Exit" {
            # "Do not put any code in this frame.\n(No errors that occur here will be handled.)"
            n393 = Unbundle By Name(w830) -> ("Core.Last Error.error"=w829:errorcluster)
            n394 = call <vilib>:"Add State(s) to Queue__jki_lib_state_machine.vi"("State(s) in (\"\")"=w834) -> ("States Out"=w833:string)  [unwired: 14 in]
          }
          frame "---------- Data ----------" {
            # "Do not put any code in this frame.\n(It is a separator no-op. You can make a copy of this frame to create a new Data frame)"
            n395 = call <vilib>:"Add State(s) to Queue__jki_lib_state_machine.vi"("State(s) in (\"\")"=w839) -> ("States Out"=w838:string)  [unwired: 14 in]
          }
          frame "Data: Initialize" {
            w840 = FALSE  # clear lockin charts
            w841 = waveform(dbl)[][] []  # Waveform Charts
            w842 = FALSE  # update lockin graphs
            w843 = FALSE  # update waveform graphs
            w847 = T69 {"Current VI Reference"=refnum, "Close Panel on Exit?"=FALSE, "Last Error"={"error"={"status"=FALSE, "code"=0, "source"=""}, "previous state"="", "remaining states"=""}, "Shutdown?"=FALSE}  # Core
            w846 = refnum<vi> refnum  # Front Panel
            w845 = Status--enum."idle"  # DAQ state
            (unwired) string[] []  # Plot Names
            w849 = refnum<class "Instrument.Lockin.lvclass"> refnum  # Lockin
            w855 = T46 {"Channels"={"Cfg_AO"=[], "Cfg_AI"=[], "Cfg_REF"=[]}, "DAQ"={"Configuration"=[], "cfg.Sampling"={"Sampling"={"Fs"=0.0, "#s"=0}, "sample mode"=0, "Fs Mode"=enum."Manual", "Fs Multiplier"=0.0, "Refresh Rate (Hz)"=0.0, "Decimation.PreDSP"=0, "Decimation.PostDSP"=0, "Fs.Output"=0.0}, "Calibration"=[], "Simulation mode"=enum."AI = HW simulated"}, "PreFilter"={"60 Hz"=FALSE, "Low Pass"=FALSE, "Low Pass Cutoff (Hz)"=0.0}, "Amplifers"={"Offset_AI"=[], "Gain_AI"=[], "Gain_AO"=[]}, "Limit Amplitude"={"Limit (V)"=0.0}, "Limit DC"={"Limit (V)"=0.0}, "Link Frequencies"={"Link?"=FALSE, "Frequency (Hz)"=0.0}, "Sweep"={"sweepTime"=0.0, "initialWaitTime"=0.0, "returnToStart"=FALSE, "sweepChannels"=[]}, "Plot"={"visibility.AI"=[], "visibility.AO"=[], "visibility.Lockin"=[], "Display 1"=enum."X", "Display 2"=enum."X"}, "Function Option"={"Option?"=FALSE, "Duty Cycle (%)"=0.0}}  # UI Config
            w856 = cluster{"Command":variant, "Data":variant} {"Command"=variant, "Data"=variant}  # Message
            w844 = T57 {"DAQ State"=enum."idle", "Waveforms"={"AO"=[], "AI"=[], "REF_X"=[], "REF_Y"=[], "X"=[], "Y"=[]}, "Results"={"Time Stamp"=timestamp(0 s since 1904-01-01), "Results (Dictionary)"=[]}, "SweepWaveforms"={"AO"=[], "AI"=[], "X"=[], "Y"=[]}}  # getAll
            w857 = refnum<class "Configuration.lvclass"> refnum  # Configuration
            w858 = T61 {"Booleans"={"Start"=refnum, "Pause"=refnum, "Reset"=refnum, "Trigger"=refnum, "Help"=refnum, "Close"=refnum, "Start Sweep"=refnum, "Stop Sweep"=refnum}, "Clusters"={"AO Channels"=refnum, "AI Channels"=refnum, "REF Channels"=refnum, "DAQ Config"=refnum, "Sweep Channels"=refnum, "Cal Info"=refnum}, "Graphs"={"AI Graph"=refnum, "AO Graph"=refnum, "REF Graph"=refnum, "Lockin 1"=refnum, "Lockin 2"=refnum, "Lockin XY"=refnum, "Sweep X Graph"=refnum, "Sweep Y Graph"=refnum, "Sweep AI Graph"=refnum, "Sweep AO Graph"=refnum, "PS WFGraph"=refnum, "PS Chart"=refnum}}  # References
            # "do not delete - used by framework"
            # "Initialize the shift-register data, here.\n(data names are defined by what you wire into the bundle function)"
            n396 = call <userlib>:"Read Instrument.vi"("error in (no error)"=w851, "Instrument UI in"=w853) -> ("error out"=w850:errorcluster, "Instrument"=w854:refnum<class "Instrument.lvclass">)  [unwired: 7 in, 1 out]
            n397 = To More Specific Class(target class=w849, reference=w854, error in=w850) -> (specific class reference=w848:refnum<class "Instrument.Lockin.lvclass">, error out=w852:errorcluster)
            n398 = Bundle("Core"=w847, "SMO"=w853, "Lockin"=w848, "Configuration"=w857, "UI Config"=w855, "DAQ state"=w845, "getAll"=w844, "Waveform Charts"=w841, "References"=w858, "Message"=w856, "Front Panel"=w846, "update waveform graphs"=w843, "update lockin graphs"=w842, "clear lockin charts"=w840) -> (w860:T65)  [unwired: 1 in]
            n399 = call <vilib>:"Add State(s) to Queue__jki_lib_state_machine.vi"("State(s) in (\"\")"=w862) -> ("States Out"=w861:string)  [unwired: 14 in]
          }
          frame "Data: Initialize Control References" {
            n400 = Unbundle By Name(w864) -> ("Core.Current VI Reference"=w863:refnum<vi>)
            n401 = control-ref of="Start"() -> (w872:refnum<vi>)
            n402 = control-ref of="Pause"() -> (w871:refnum<vi>)
            n403 = control-ref of="Reset"() -> (w870:refnum<vi>)
            n404 = control-ref of="Help"() -> (w869:refnum<vi>)
            n405 = control-ref of="Close"() -> (w868:refnum<vi>)
            n406 = control-ref of="Start Sweep"() -> (w867:refnum<vi>)
            n407 = control-ref of="Stop Sweep"() -> (w866:refnum<vi>)
            n408 = control-ref of="AO Channels"() -> (w878:refnum<vi>)
            n409 = control-ref of="AI Channels"() -> (w873:refnum<vi>)
            n410 = control-ref of="REF Channels"() -> (w877:refnum<vi>)
            n411 = control-ref of="DAQ Config"() -> (w876:refnum<vi>)
            n412 = control-ref of="Sweep Channels"() -> (w875:refnum<vi>)
            n413 = control-ref of="Cal Info"() -> (w874:refnum<vi>)
            n414 = property class="VI"(reference=w863) -> ("Front Panel"=w865:refnum<vi>)  [unwired: 1 in, 2 out]
            n415 = Bundle By Name(cluster=w864, "References.Booleans.Start"=w872, "References.Booleans.Pause"=w871, "References.Booleans.Reset"=w870, "References.Booleans.Help"=w869, "References.Booleans.Close"=w868, "References.Booleans.Start Sweep"=w867, "References.Booleans.Stop Sweep"=w866, "References.Clusters.AO Channels"=w878, "References.Clusters.AI Channels"=w873, "References.Clusters.REF Channels"=w877, "References.Clusters.DAQ Config"=w876, "References.Clusters.Sweep Channels"=w875, "References.Clusters.Cal Info"=w874, "Front Panel"=w865) -> (w879:T65)
            n416 = call <vilib>:"Add State(s) to Queue__jki_lib_state_machine.vi"("State(s) in (\"\")"=w883) -> ("States Out"=w882:string)  [unwired: 14 in]
          }
          frame "Data: Initialize Graph References" {
            n417 = control-ref of="REF Graph"() -> (w884:refnum<vi>)
            n418 = control-ref of="Lockin 1"() -> (w894:refnum<vi>)
            n419 = control-ref of="Lockin 2"() -> (w893:refnum<vi>)
            n420 = control-ref of="AI Graph"() -> (w896:refnum<vi>)
            n421 = control-ref of="AO Graph"() -> (w895:refnum<vi>)
            n422 = control-ref of="Lockin XY"() -> (w892:refnum<vi>)
            n423 = control-ref of="Sweep X"() -> (w885:refnum<vi>)
            n424 = control-ref of="Sweep Y"() -> (w886:refnum<vi>)
            n425 = control-ref of="Sweep AI"() -> (w887:refnum<vi>)
            n426 = control-ref of="Sweep AO"() -> (w888:refnum<vi>)
            n427 = control-ref of="PS Waveform"() -> (w891:refnum<vi>)
            n428 = Bundle By Name(cluster=w890, "References.Graphs.AI Graph"=w896, "References.Graphs.AO Graph"=w895, "References.Graphs.REF Graph"=w884, "References.Graphs.Lockin 1"=w894, "References.Graphs.Lockin 2"=w893, "References.Graphs.Lockin XY"=w892, "References.Graphs.Sweep X Graph"=w885, "References.Graphs.Sweep Y Graph"=w886, "References.Graphs.Sweep AI Graph"=w887, "References.Graphs.Sweep AO Graph"=w888, "References.Graphs.PS WFGraph"=w891) -> (w889:T65)
            n429 = call <vilib>:"Add State(s) to Queue__jki_lib_state_machine.vi"("State(s) in (\"\")"=w900) -> ("States Out"=w899:string)  [unwired: 14 in]
          }
          frame "Data: Waveform Legends" {
            n430 = Unbundle By Name(w924) -> ("getAll.Waveforms.AI"=w923:waveform(dbl)[], "getAll.Waveforms.AO"=w922:waveform(dbl)[], "getAll.Waveforms.REF_X"=w905:waveform(dbl)[])
            n431 = Array Size(array=w923) -> (size(s)=w918:i32)
            n432 = Array Size(array=w922) -> (size(s)=w920:i32)
            n433 = Array Size(array=w905) -> (size(s)=w902:i32)
            n434 = call "Is Value Changed.vim"("value"=w902) -> ("changed or first call?"=w901:bool)
            n435 = call "Is Value Changed.vim"("value"=w918) -> ("changed or first call?"=w917:bool)
            n436 = call "Is Value Changed.vim"("value"=w920) -> ("changed or first call?"=w919:bool)
            n437 = Select(t="UI: Update AI Waveform Graphs Legends\nUI: Update AI Waveform Graphs Colors", s=w917, f="") -> (s? t:f=w907:string)
            n438 = Select(t="UI: Update AO Waveform Graphs Legends\nUI: Update AO Waveform Graphs Colors", s=w919, f="") -> (s? t:f=w908:string)
            n439 = Select(t="UI: Update REF Waveform Graphs Legends\nUI: Update REF Waveform Graphs Colors", s=w901, f="") -> (s? t:f=w903:string)
            n440 = call <vilib>:"Add State(s) to Queue__jki_lib_state_machine.vi"("State(s) in Front (\"\")"=w907, "State(s) in (\"\")"=w908, "State(s) at Back (\"\")"=w903) -> ("States Out"=w910:string)  [unwired: 12 in]
            n441 = call <vilib>:"Add State(s) to Queue__jki_lib_state_machine.vi"("State(s) in Front (\"\")"="UI: Defer Panel Updates >> TRUE" ("State(s) in Front (\"\")"), "State(s) in (\"\")"=w910, "State(s) at Back (\"\")"="UI: Defer Panel Updates >> FALSE" ("State(s) in Front (\"\")")) -> ("States Out"=w911:string)  [unwired: 12 in]
            n442 = Empty String/Path?(string/path=w910) -> (empty?=w914:bool)
            n443 = Select(t=w910, s=w914, f=w911) -> (s? t:f=w909:string)
            n444 = call <vilib>:"Add State(s) to Queue__jki_lib_state_machine.vi"("State(s) in Front (\"\")"=w909, "State(s) in (\"\")"=w929) -> ("States Out"=w928:string)  [unwired: 13 in]
          }
          frame "Data: Wait" {
            # "Data: wait.\n(wait for X ms)"
            n445 = Scan From String(input string=w930, default 1=u32 0 ("milliseconds to wait")) -> (output 1=w931:u32)  [unwired: 3 in, 3 out]
            n446 = Wait (ms)(milliseconds to wait=w931) -> ()  [unwired: 1 out]
            n447 = call <vilib>:"Add State(s) to Queue__jki_lib_state_machine.vi"("State(s) in (\"\")"=w937) -> ("States Out"=w936:string)  [unwired: 14 in]
          }
          frame "Data: Cleanup" {
            # "Cleanup any data and references, here.\n(this is called automatically, by the Macro: Exit)"
            n448 = Unbundle By Name(w939) -> ("Core.Current VI Reference"=w942:refnum<vi>)
            n449 = Close Reference(reference=w942, error in (no error)=w941) -> (error out=w940:errorcluster)
            n450 = call <vilib>:"Add State(s) to Queue__jki_lib_state_machine.vi"("State(s) in (\"\")"=w944) -> ("States Out"=w943:string)  [unwired: 14 in]
          }
          frame "---------- Configuration ----------" {
            # "Do not put any code in this frame.\n(It is a separator no-op. You can make a copy of this frame to create a new Data frame)"
            n451 = call <vilib>:"Add State(s) to Queue__jki_lib_state_machine.vi"("State(s) in (\"\")"=w949) -> ("States Out"=w948:string)  [unwired: 14 in]
          }
          frame "Configuration: Initialize" {
            # "Do not put any code in this frame.\n(It is a separator no-op. You can make a copy of this frame to create a new Data frame)"
            n452 = Unbundle By Name(w959) -> ("Lockin"=w958:refnum<class "Instrument.Lockin.lvclass">)
            n453 = call <vilib>:"GetName.vi"("error in (no error)"=w957, "SMO"=w958) -> ("error out"=w955:errorcluster, "Name"=w956:string)  [unwired: 6 in, 2 out]
            n454 = call <userlib>:"Default Path.vi"("error in (no error)"=w955, "Folder Name [Application Name]"=w956) -> ("error out"=w952:errorcluster, "Configuration out"=w954:refnum<class "Configuration.lvclass">)  [unwired: 8 in]
            n455 = call <userlib>:"Write Section.vi"("error in (no error)"=w952, "Section"="UI", "Configuration in"=w954) -> ("error out"=w951:errorcluster, "Configuration out"=w953:refnum<class "Configuration.lvclass">)  [unwired: 7 in]
            n456 = Bundle By Name(cluster=w959, "Configuration"=w953) -> (w960:T65)
            n457 = call <vilib>:"Add State(s) to Queue__jki_lib_state_machine.vi"("State(s) in (\"\")"=w963) -> ("States Out"=w962:string)  [unwired: 14 in]
          }
          frame "Configuration: Write File" {
            # "Do not put any code in this frame.\n(It is a separator no-op. You can make a copy of this frame to create a new Data frame)"
            n458 = Unbundle By Name(w969) -> ("Configuration"=w964:refnum<class "Configuration.lvclass">, "UI Config"=w965:T46)
            n459 = call <userlib>:"Write Configuration.vi"("error in (no error)"=w966, "Variant"=w965, "Configuration in"=w964) -> ("error out"=w968:errorcluster, "Configuration out"=w967:refnum<class "Configuration.lvclass">)  [unwired: 7 in]
            n460 = Bundle By Name(cluster=w969, "Configuration"=w967) -> (w970:T65)
            n461 = call <vilib>:"Add State(s) to Queue__jki_lib_state_machine.vi"("State(s) in (\"\")"=w973) -> ("States Out"=w972:string)  [unwired: 14 in]
          }
          frame "Configuration: Read File" {
            # "Do not put any code in this frame.\n(It is a separator no-op. You can make a copy of this frame to create a new Data frame)"
            n462 = Unbundle By Name(w982) -> ("Configuration"=w974:refnum<class "Configuration.lvclass">, "UI Config"=w976:T46)
            n463 = call <userlib>:"Read Configuration.vi"("INI Fomatted Cluster Type"=w976, "error in (no error)"=w978, "Configuration in"=w974) -> ("error out"=w980:errorcluster, "Configuration"=w981:variant, "Configuration out"=w979:refnum<class "Configuration.lvclass">)  [unwired: 6 in]
            n464 = Variant To Data(error in=w980, type=w976, Variant=w981) -> (data=w975:T46, error out=w977:errorcluster)
            n465 = Bundle By Name(cluster=w982, "Configuration"=w979, "UI Config"=w975) -> (w983:T65)
            n466 = call <vilib>:"Add State(s) to Queue__jki_lib_state_machine.vi"("State(s) in (\"\")"=w986) -> ("States Out"=w985:string)  [unwired: 14 in]
          }
          frame "---------- UI ----------" {
            # "Do not put any code in this frame.\n(It is a separator no-op. You can make a copy of this frame to create a new UI frame)"
            n467 = call <vilib>:"Add State(s) to Queue__jki_lib_state_machine.vi"("State(s) in (\"\")"=w991) -> ("States Out"=w990:string)  [unwired: 14 in]
          }
          frame "UI: Initialize" {
            # "size window to decoration box on front panel"
            # "Initialize the User Interface here.\n(this is called automatically, by the Macro: Init)"
            n468 = call "Application Version.vi"() -> ("Version"=→"Version" →"Application Version":string)
            n469 = call <userlib>:"Fit VI window to Largest Dec__ogtk.vi"("error in (no error)"=w1000, "border spacing (2 px)"=-4) -> ("error out"=w999:errorcluster)  [unwired: 4 in, 1 out]
            n470 = local write "Sampling Status"(u32 6618880) -> ()
            n471 = call <vilib>:"Build State String with Arguments__JKI_lib_State_Machine.vi"("Arguments (\"\")"="Initializing..." ("Status"), "State"="UI: Update Status") -> ("State with Arguments"=w994:string)  [unwired: 4 in]
            n472 = call <vilib>:"Add State(s) to Queue__jki_lib_state_machine.vi"("State(s) in Front (\"\")"=w994, "State(s) in (\"\")"=w1003) -> ("States Out"=w1002:string)  [unwired: 13 in]
          }
          frame "UI: Cursor Set" {
            # "Argument"
            # "Initialize the User Interface, here.\n(this is called automatically, by the Macro: Init)"
            n473 = disable-structure shown="Default" {
              disable-tunnel: w1006 -> [w1011 w1014]
              disable-tunnel: [w1011 w1013] -> w1005
              disable-tunnel: w1004 -> [_ w1012]
              frame condition #0 {
              }
              frame condition #1 (active) {
                n474 = case shown="\"Idle\", Default" w1012 {
                  tunnel: w1014 -> [w1016 w1018]
                  tunnel: [w1015 w1017] -> w1013
                  frame "Idle", Default {
                    n475 = call <vilib>:"Unset Busy.vi"("error in (no error)"=w1016) -> ("error out"=w1015:errorcluster)  [unwired: 10 in]
                  }
                  frame "Busy" {
                    n476 = call <vilib>:"Set Busy.vi"("error in (no error)"=w1018) -> ("error out"=w1017:errorcluster)  [unwired: 9 in, 1 out]
                  }
                }
              }
            }
            n477 = call <vilib>:"Add State(s) to Queue__jki_lib_state_machine.vi"("State(s) in (\"\")"=w1010) -> ("States Out"=w1009:string)  [unwired: 14 in]
          }
          frame "UI: Front Panel State" {
            # "Argument"
            # "Set Front Panel Open or Closed\n(Usage: \"UI: Front Panel State >> Open|Close\")"
            n478 = Unbundle By Name(w1022) -> ("Core.Current VI Reference"=w1021:refnum<vi>)
            n479 = disable-structure shown="Default" {
              disable-tunnel: w1024 -> [w1030 w1053]
              disable-tunnel: [w1029 w1053] -> w1023
              disable-tunnel: w1021 -> [w1028 _]
              disable-tunnel: w1020 -> [w1027 _]
              frame condition #0 (active) {
                n480 = case shown="\"Close\"" w1027 {
                  tunnel: w1030 -> [w1034 w1047]
                  tunnel: [w1036 w1048] -> w1029
                  tunnel: w1028 -> [w1035 w1045]
                  frame "Open", Default {
                    n481 = property class="VI"(reference=w1035, error in=w1034) -> (reference out=w1032:refnum<vi>, error out=w1033:errorcluster, "FP.State"=w1031:T35)
                    n482 = case shown="\"Closed\"" w1031 {
                      tunnel: [w1039 w1042] -> w1036
                      tunnel: w1033 -> [w1038 w1042]
                      tunnel: w1032 -> [w1037 _]
                      frame "Closed" {
                        n483 = invoke class="VI" method="FP.Open"(reference=w1037, error in=w1038, "Activate"=TRUE, "State"=T35."Standard") -> (error out=w1039:errorcluster)  [unwired: 1 in, 4 out]
                      }
                      frame Default {
                      }
                    }
                  }
                  frame "Close" {
                    n484 = property class="VI"(reference=w1045, error in=w1047) -> (reference out=w1044:refnum<vi>, error out=w1046:errorcluster, "FP.State"=w1043:T35)
                    n485 = case shown="Default" w1043 {
                      tunnel: [w1049 w1052] -> w1048
                      tunnel: w1046 -> [w1049 w1051]
                      tunnel: w1044 -> [_ w1050]
                      frame "Invalid", "Closed" {
                      }
                      frame Default {
                        n486 = invoke class="VI" method="FP.Close"(reference=w1050, error in=w1051) -> (error out=w1052:errorcluster)  [unwired: 1 in, 2 out]
                      }
                    }
                  }
                }
              }
              frame condition #1 {
              }
            }
            n487 = call <vilib>:"Add State(s) to Queue__jki_lib_state_machine.vi"("State(s) in (\"\")"=w1026) -> ("States Out"=w1025:string)  [unwired: 14 in]
          }
          frame "UI: Defer Panel Updates" {
            # "Do not put any code in this frame.\n(It is a separator no-op. You can make a copy of this frame to create a new UI frame)"
            n488 = Unbundle By Name(w1058) -> ("Front Panel"=w1056:refnum<vi>)
            n489 = Scan From String(input string=w1057, default 1=FALSE) -> (output 1=w1055:bool)  [unwired: 3 in, 3 out]
            n490 = property class="Pnl"(reference=w1056, "Defer Panel Updates"=w1055) -> ()  [unwired: 1 in, 2 out]
            n491 = call <vilib>:"Add State(s) to Queue__jki_lib_state_machine.vi"("State(s) in (\"\")"=w1062) -> ("States Out"=w1061:string)  [unwired: 14 in]
          }
          frame "UI: Set Left Tab" {
            # "Do not put any code in this frame.\n(It is a separator no-op. You can make a copy of this frame to create a new UI frame)"
            n492 = Scan From String(input string=w1065, default 1=T1."AO/AI/REF" ("Left Tab")) -> (output 1=w1064:T1)  [unwired: 3 in, 3 out]
            n493 = local write "Left Tab"(w1064) -> ()
            n494 = call <vilib>:"Add State(s) to Queue__jki_lib_state_machine.vi"("State(s) in (\"\")"=w1070) -> ("States Out"=w1069:string)  [unwired: 14 in]
          }
          frame "UI: Set Right Tab" {
            # "Do not put any code in this frame.\n(It is a separator no-op. You can make a copy of this frame to create a new UI frame)"
            n495 = Scan From String(input string=w1073, default 1=T25."AO/AI Graphs" ("Right Tab")) -> (output 1=w1072:T25)  [unwired: 3 in, 3 out]
            n496 = local write "Right Tab"(w1072) -> ()
            n497 = call <vilib>:"Add State(s) to Queue__jki_lib_state_machine.vi"("State(s) in (\"\")"=w1078) -> ("States Out"=w1077:string)  [unwired: 14 in]
          }
          frame "UI: Init Scroll Bars" {
            w1080 = u32[] [0] ("Index Values")
            w1079 = u32 0 ("Legend:Scroll Position")
            # "UI: Init Scroll Bars.\n(Scroll to the top)"
            n498 = property on="Lockin 1" class="WFGraph (strict)"("LegScrollPos"=w1079) -> ()  [unwired: 2 in, 2 out]
            n499 = property on="Lockin 2" class="WFGraph (strict)"("LegScrollPos"=w1079) -> ()  [unwired: 2 in, 2 out]
            n500 = property on="AI Graph" class="WFGraph (strict)"("LegScrollPos"=w1079) -> ()  [unwired: 2 in, 2 out]
            n501 = property on="AO Graph" class="WFGraph (strict)"("LegScrollPos"=w1079) -> ()  [unwired: 2 in, 2 out]
            n502 = property on="REF Graph" class="WFGraph (strict)"("LegScrollPos"=w1079) -> ()  [unwired: 2 in, 2 out]
            n503 = property on="Lockin XY" class="XYGraph (strict)"("LegScrollPos"=w1079) -> ()  [unwired: 2 in, 2 out]
            n504 = property on="AO Channels" class="Arr (strict)"("Index Values"=w1080) -> ()  [unwired: 2 in, 2 out]
            n505 = property on="DAQ Config" class="Arr (strict)"("Index Values"=w1080) -> ()  [unwired: 2 in, 2 out]
            n506 = property on="Sweep AI" class="WFGraph (strict)"("LegScrollPos"=w1079) -> ()  [unwired: 2 in, 2 out]
            n507 = property on="Sweep AO" class="WFGraph (strict)"("LegScrollPos"=w1079) -> ()  [unwired: 2 in, 2 out]
            n508 = property on="Sweep X" class="WFGraph (strict)"("LegScrollPos"=w1079) -> ()  [unwired: 2 in, 2 out]
            n509 = property on="Sweep Y" class="WFGraph (strict)"("LegScrollPos"=w1079) -> ()  [unwired: 2 in, 2 out]
            n510 = property on="PS Waveform" class="WFGraph (strict)"("LegScrollPos"=w1079) -> ()  [unwired: 2 in, 2 out]
            n511 = property on="AI Channels" class="Arr (strict)"("Index Values"=w1080) -> ()  [unwired: 2 in, 2 out]
            n512 = call <vilib>:"Add State(s) to Queue__jki_lib_state_machine.vi"("State(s) in (\"\")"=w1085) -> ("States Out"=w1084:string)  [unwired: 14 in]
          }
          frame "UI: Update Status" {
            # "UI: Update Status.\n()"
            n513 = case shown="Default" w1086 {
              selector: w1086 -> [w1092 _]
              frame Default {
                "String" <- w1092
              }
              frame "" {
              }
            }
            n514 = call <vilib>:"Add State(s) to Queue__jki_lib_state_machine.vi"("State(s) in (\"\")"=w1091) -> ("States Out"=w1090:string)  [unwired: 14 in]
          }
          frame "UI: Cluster to UI" {
            # "Initialize the UI elements from data wire\n(this is called automatically, by the Macro: Init)"
            n515 = Unbundle By Name(w1101) -> ("UI Config.Channels.Cfg_AO"=w1116:T6, "UI Config.Channels.Cfg_AI"=w1114:T4, "UI Config.Channels.Cfg_REF"=w1115:T2, "UI Config.DAQ.Configuration"=w1108:T9, "UI Config.DAQ.cfg.Sampling.Sampling.Fs"=w1097:dbl, "UI Config.DAQ.cfg.Sampling.Sampling.#s"=w1096:i32, "UI Config.DAQ.cfg.Sampling.Fs Mode"=w1093:T15, "UI Config.DAQ.cfg.Sampling.Fs Multiplier"=w1109:dbl, "UI Config.DAQ.cfg.Sampling.Refresh Rate (Hz)"=w1110:dbl, "UI Config.DAQ.cfg.Sampling.Fs.Output"=w1100:dbl, "UI Config.DAQ.cfg.Sampling.Decimation.PreDSP"=w1106:i32, "UI Config.DAQ.Simulation mode"=w1107:T16, "UI Config.PreFilter.60 Hz"=w1113:bool, "UI Config.PreFilter.Low Pass"=w1112:bool, "UI Config.PreFilter.Low Pass Cutoff (Hz)"=w1111:dbl, "UI Config.Amplifers.Offset_AI"=w1094:T17, "UI Config.Amplifers.Gain_AI"=w1099:T17, "UI Config.Amplifers.Gain_AO"=w1095:T17, "UI Config.Sweep.sweepTime"=w1102:dbl, "UI Config.Sweep.initialWaitTime"=w1103:dbl, "UI Config.Sweep.returnToStart"=w1104:bool, "UI Config.Sweep.sweepChannels"=w1105:T20)
            n516 = local write "Actual #s (S)"(w1096) -> ()
            n517 = local write "Actual Fs (S/s)"(w1097) -> ()
            n518 = local write "Input Offsets"(w1094) -> ()
            n519 = local write "Input Gain"(w1099) -> ()
            n520 = local write "Output Gain"(w1095) -> ()
            n521 = local write "Fs Output (S/s)"(w1100) -> ()
            n522 = local write "Fs (S/s) (buffer)"(w1097) -> ()
            n523 = local write "#s (S) (buffer)"(w1096) -> ()
            n524 = local write "AO Channels"(w1116) -> ()
            n525 = local write "AI Channels"(w1114) -> ()
            n526 = local write "REF Channels"(w1115) -> ()
            n527 = local write "DAQ Config"(w1108) -> ()
            n528 = local write "Fs Multiplier"(w1109) -> ()
            n529 = local write "Refresh Rate (Hz)"(w1110) -> ()
            n530 = local write "Decimation (pre DSP)"(w1106) -> ()
            n531 = local write "AI Simulation mode"(w1107) -> ()
            n532 = local write "Line"(w1113) -> ()
            n533 = local write "Lowpass"(w1112) -> ()
            n534 = local write "LP f (Hz)"(w1111) -> ()
            n535 = local write "Sweep Time (s)"(w1102) -> ()
            n536 = local write "Initial Wait (s)"(w1103) -> ()
            n537 = local write "Return to Start?"(w1104) -> ()
            n538 = local write "Sweep Channels"(w1105) -> ()
            n539 = local write "Fs Mode"(w1093) -> ()
            n540 = call <vilib>:"Add State(s) to Queue__jki_lib_state_machine.vi"("State(s) in Front (\"\")"="" ("State(s) in Front (\"\")"), "State(s) in (\"\")"=w1120) -> ("States Out"=w1119:string)  [unwired: 13 in]
          }
          frame "UI: Cluster to UI 2" {
            # "Initialize the UI elements from data wire (2)\n(this is called automatically by Macro: Init)"
            n541 = Unbundle By Name(w1127) -> ("UI Config.Limit Amplitude.Limit (V)"=w1126:dbl, "UI Config.Limit DC.Limit (V)"=w1123:dbl, "UI Config.Link Frequencies.Link?"=w1124:bool, "UI Config.Link Frequencies.Frequency (Hz)"=w1125:dbl, "UI Config.Plot.Display 1"=w1122:T26, "UI Config.Plot.Display 2"=w1121:T26)
            n542 = local write "Display 1"(w1122) -> ()
            n543 = local write "Link f?"(w1124) -> ()
            n544 = local write "Display 2"(w1121) -> ()
            n545 = local write "AC Limit"(w1126) -> ()
            n546 = local write "f link (Hz)"(w1125) -> ()
            n547 = local write "AO DC Limit"(w1123) -> ()
            n548 = call <vilib>:"Add State(s) to Queue__jki_lib_state_machine.vi"("State(s) in (\"\")"=w1131) -> ("States Out"=w1130:string)  [unwired: 14 in]
          }
          frame "UI: UI to Cluster" {
            # "Write UI elements to data wire\n(this is called automatically, by the Macro: Save Configuration)"
            n549 = local read "AO Channels"() -> (w1154:T6)
            n550 = local read "AI Channels"() -> (w1152:T4)
            n551 = local read "REF Channels"() -> (w1153:T2)
            n552 = local read "DAQ Config"() -> (w1145:T9)
            n553 = local read "Fs Mode"() -> (w1148:T15)
            n554 = local read "Fs Multiplier"() -> (w1146:dbl)
            n555 = local read "Refresh Rate (Hz)"() -> (w1147:dbl)
            n556 = local read "Decimation (pre DSP)"() -> (w1143:i32)
            n557 = local read "AI Simulation mode"() -> (w1144:T16)
            n558 = local read "Line"() -> (w1151:bool)
            n559 = local read "Lowpass"() -> (w1150:bool)
            n560 = local read "LP f (Hz)"() -> (w1149:dbl)
            n561 = local read "Sweep Time (s)"() -> (w1139:dbl)
            n562 = local read "Initial Wait (s)"() -> (w1140:dbl)
            n563 = local read "Return to Start?"() -> (w1141:bool)
            n564 = local read "Sweep Channels"() -> (w1142:T20)
            n565 = local read "Actual #s (S)"() -> (w1135:i32)
            n566 = local read "Actual Fs (S/s)"() -> (w1134:dbl)
            n567 = local read "Fs Output (S/s)"() -> (w1133:dbl)
            n568 = local read "Input Offsets"() -> (w1136:T17)
            n569 = local read "Input Gain"() -> (w1138:T17)
            n570 = local read "Output Gain"() -> (w1137:T17)
            n571 = Bundle By Name(cluster=w1155, "UI Config.Channels.Cfg_AO"=w1154, "UI Config.Channels.Cfg_AI"=w1152, "UI Config.Channels.Cfg_REF"=w1153, "UI Config.DAQ.Configuration"=w1145, "UI Config.DAQ.cfg.Sampling.Sampling.Fs"=w1134, "UI Config.DAQ.cfg.Sampling.Sampling.#s"=w1135, "UI Config.DAQ.cfg.Sampling.Fs Mode"=w1148, "UI Config.DAQ.cfg.Sampling.Fs Multiplier"=w1146, "UI Config.DAQ.cfg.Sampling.Refresh Rate (Hz)"=w1147, "UI Config.DAQ.cfg.Sampling.Fs.Output"=w1133, "UI Config.DAQ.cfg.Sampling.Decimation.PreDSP"=w1143, "UI Config.DAQ.Simulation mode"=w1144, "UI Config.PreFilter.60 Hz"=w1151, "UI Config.PreFilter.Low Pass"=w1150, "UI Config.PreFilter.Low Pass Cutoff (Hz)"=w1149, "UI Config.Amplifers.Offset_AI"=w1136, "UI Config.Amplifers.Gain_AI"=w1138, "UI Config.Amplifers.Gain_AO"=w1137, "UI Config.Sweep.sweepTime"=w1139, "UI Config.Sweep.initialWaitTime"=w1140, "UI Config.Sweep.returnToStart"=w1141, "UI Config.Sweep.sweepChannels"=w1142) -> (w1156:T65)
            n572 = call <vilib>:"Add State(s) to Queue__jki_lib_state_machine.vi"("State(s) in Front (\"\")"="" ("State(s) in Front (\"\")"), "State(s) in (\"\")"=w1160) -> ("States Out"=w1159:string)  [unwired: 13 in]
          }
          frame "UI: UI to Cluster 2" {
            # "Write UI elements to data wire (2)\n(this is called automatically, by the Macro: Save Configuration)"
            n573 = local read "Link f?"() -> (w1166:bool)
            n574 = local read "Display 1"() -> (w1162:T26)
            n575 = local read "Display 2"() -> (w1161:T26)
            n576 = local read "AO DC Limit"() -> (w1167:dbl)
            n577 = local read "f link (Hz)"() -> (w1165:dbl)
            n578 = local read "AC Limit"() -> (w1168:dbl)
            n579 = Bundle By Name(cluster=w1163, "UI Config.Limit Amplitude.Limit (V)"=w1168, "UI Config.Limit DC.Limit (V)"=w1167, "UI Config.Link Frequencies.Link?"=w1166, "UI Config.Link Frequencies.Frequency (Hz)"=w1165, "UI Config.Plot.Display 1"=w1162, "UI Config.Plot.Display 2"=w1161) -> (w1164:T65)
            n580 = call <vilib>:"Add State(s) to Queue__jki_lib_state_machine.vi"("State(s) in (\"\")"=w1172) -> ("States Out"=w1171:string)  [unwired: 14 in]
          }
          frame "UI: Reinit To Default" {
            # "UI: Reinit To Default.\n(I)"
            n581 = Unbundle By Name(w1173) -> ("References.Booleans"=w1175:T62, "References.Graphs.Lockin 1"=w1177:refnum<vi>, "References.Graphs.Lockin 2"=w1176:refnum<vi>)
            n582 = Cluster To Array(cluster=w1175) -> (array=w1174:refnum<vi>[])
            n583 = for {
              tunnel: w1174 -> [w1182] mode=indexing
              n584 = invoke on="Invoke Node" class="Bool (strict)" method="Reinit To Default"(reference=w1182) -> ()  [unwired: 2 in, 3 out]
            }
            n585 = invoke on="Invoke Node" class="WFGraph (strict)" method="Reinit To Default"(reference=w1177) -> ()  [unwired: 2 in, 3 out]
            n586 = invoke on="Invoke Node" class="WFGraph (strict)" method="Reinit To Default"(reference=w1176) -> ()  [unwired: 2 in, 3 out]
            n587 = call <vilib>:"Add State(s) to Queue__jki_lib_state_machine.vi"("State(s) in (\"\")"=w1181) -> ("States Out"=w1180:string)  [unwired: 14 in]
          }
          frame "UI: Disable Buttons" {
            # "UI: Disable Buttons\n(Disable all booleans)"
            n588 = Unbundle By Name(w1184) -> ("References.Booleans"=w1185:T62)
            n589 = Cluster To Array(cluster=w1185) -> (array=w1183:refnum<vi>[])
            n590 = for {
              tunnel: w1183 -> [w1190] mode=indexing
              n591 = property class="Bool (strict)"(reference=w1190, "DisabledEnum"=T36."Disabled and Grayed Out" ("Disabled")) -> ()  [unwired: 1 in, 2 out]
            }
            n592 = call <vilib>:"Add State(s) to Queue__jki_lib_state_machine.vi"("State(s) in (\"\")"=w1189) -> ("States Out"=w1188:string)  [unwired: 14 in]
          }
          frame "UI: Enable Buttons" {
            # "UI: Enable Buttons.\n(Enable booleans after SMO starts.)"
            n593 = Unbundle By Name(w1194) -> ("References.Booleans"=w1193:T62)
            n594 = Cluster To Array(cluster=w1193) -> (array=w1192:refnum<vi>[])
            n595 = for {
              tunnel: w1192 -> [w1199] mode=indexing
              n596 = property class="Bool (strict)"(reference=w1199, "DisabledEnum"=T36."Enabled" ("Disabled")) -> ()  [unwired: 1 in, 2 out]
            }
            n597 = call <vilib>:"Add State(s) to Queue__jki_lib_state_machine.vi"("State(s) in (\"\")"=w1198) -> ("States Out"=w1197:string)  [unwired: 14 in]
          }
          frame "UI: Update Booleans" {
            # "UI: Update Booleans.\n(Call in response to state upate)"
            n598 = Unbundle By Name(w1203) -> ("DAQ state"=w1202:T33, "References.Booleans.Start"=w1209:refnum<vi>, "References.Booleans.Pause"=w1208:refnum<vi>, "References.Booleans.Reset"=w1210:refnum<vi>, "References.Booleans.Trigger"=w1207:refnum<vi>, "References.Booleans.Start Sweep"=w1206:refnum<vi>, "References.Booleans.Stop Sweep"=w1204:refnum<vi>)
            n599 = case shown="\"idle\", Default" w1202 {
              tunnel: w1210 -> [w1221 w1227 w1230 w1233 _]
              tunnel: w1209 -> [w1222 w1224 w1231 w1234 _]
              tunnel: w1208 -> [_ _ _ _ _]
              tunnel: w1207 -> [w1220 _ w1229 _ _]
              tunnel: w1206 -> [_ w1226 _ _ _]
              tunnel: [w1219 w1228 w1232 w1236 _] -> w1205
              tunnel: [_ w1223 _ w1235 _] -> w1201
              tunnel: w1204 -> [_ w1225 _ _ _]
              frame "idle", Default {
                n600 = Build Array(w1222, w1221, w1220) -> (w1219:refnum<vi>[])
              }
              frame "started" {
                n601 = Build Array(w1224) -> (w1223:refnum<vi>[])
                n602 = Build Array(w1227, w1226, w1225) -> (w1228:refnum<vi>[])
              }
              frame "stopped" {
                n603 = Build Array(w1231, w1230, w1229) -> (w1232:refnum<vi>[])
              }
              frame "created" {
                n604 = Build Array(w1234) -> (w1235:refnum<vi>[])
                n605 = Build Array(w1233) -> (w1236:refnum<vi>[])
              }
              frame "sweeping" {
              }
            }
            n606 = for {
              tunnel: w1201 -> [w1215] mode=indexing
              n607 = property class="Bool (strict)"(reference=w1215, "Value"=TRUE) -> ()  [unwired: 1 in, 2 out]
            }
            n608 = for {
              tunnel: w1205 -> [w1217] mode=indexing
              n609 = property class="Bool (strict)"(reference=w1217, "Value"=FALSE) -> ()  [unwired: 1 in, 2 out]
            }
            n610 = call <vilib>:"Add State(s) to Queue__jki_lib_state_machine.vi"("State(s) in (\"\")"=w1214) -> ("States Out"=w1213:string)  [unwired: 14 in]
          }
          frame "UI: AI Graphs Plot Visibility" {
            n611 = Unbundle By Name(w1241) -> ("References.Graphs.AI Graph"=w1240:refnum<vi>, "References.Graphs.Sweep AI Graph"=w1237:refnum<vi>)
            n612 = case shown="\"None\", Default" w1239 {
              tunnel: [FALSE TRUE] -> w1238
              frame "None", Default {
              }
              frame "ALL" {
              }
            }
            n613 = call-poly "Set All Plot Visibility.vi"("error in (no error)"=w1242, "All Visible?"=w1238, "WFGraph in"=w1237) -> ("error out"=w1244:errorcluster)  [unwired: 8 in]
            n614 = call-poly "Set All Plot Visibility.vi"("error in (no error)"=w1244, "All Visible?"=w1238, "WFGraph in"=w1240) -> ("error out"=w1243:errorcluster)  [unwired: 8 in]
            n615 = call <vilib>:"Add State(s) to Queue__jki_lib_state_machine.vi"("State(s) in (\"\")"=w1247) -> ("States Out"=w1246:string)  [unwired: 14 in]
          }
          frame "UI: AO Graphs Plot Visibility" {
            n616 = Unbundle By Name(w1255) -> ("References.Graphs.AO Graph"=w1254:refnum<vi>, "References.Graphs.Sweep AO Graph"=w1251:refnum<vi>)
            n617 = case shown="\"ALL\"" w1253 {
              tunnel: [FALSE TRUE] -> w1250
              frame "None", Default {
              }
              frame "ALL" {
              }
            }
            n618 = call-poly "Set All Plot Visibility.vi"("error in (no error)"=w1256, "All Visible?"=w1250, "WFGraph in"=w1251) -> ("error out"=w1257:errorcluster)  [unwired: 8 in]
            n619 = call-poly "Set All Plot Visibility.vi"("error in (no error)"=w1257, "All Visible?"=w1250, "WFGraph in"=w1254) -> ("error out"=w1252:errorcluster)  [unwired: 8 in]
            n620 = call <vilib>:"Add State(s) to Queue__jki_lib_state_machine.vi"("State(s) in (\"\")"=w1260) -> ("States Out"=w1259:string)  [unwired: 14 in]
          }
          frame "UI: REF Graphs Plot Visibility" {
            n621 = Unbundle By Name(w1267) -> ("References.Graphs.REF Graph"=w1264:refnum<vi>)
            n622 = case shown="\"ALL\"" w1266 {
              tunnel: [FALSE TRUE] -> w1263
              frame "None", Default {
              }
              frame "ALL" {
              }
            }
            n623 = call-poly "Set All Plot Visibility.vi"("error in (no error)"=w1268, "All Visible?"=w1263, "WFGraph in"=w1264) -> ("error out"=w1265:errorcluster)  [unwired: 8 in]
            n624 = call <vilib>:"Add State(s) to Queue__jki_lib_state_machine.vi"("State(s) in (\"\")"=w1271) -> ("States Out"=w1270:string)  [unwired: 14 in]
          }
          frame "UI: Lockin Graphs Plot Visibility" {
            n625 = Unbundle By Name(w1285) -> ("References.Graphs.Lockin 1"=w1276:refnum<vi>, "References.Graphs.Lockin 2"=w1277:refnum<vi>, "References.Graphs.Lockin XY"=w1278:refnum<vi>, "References.Graphs.Sweep X Graph"=w1275:refnum<vi>, "References.Graphs.Sweep Y Graph"=w1274:refnum<vi>)
            n626 = case shown="\"ALL\"" w1284 {
              tunnel: [FALSE TRUE] -> w1279
              frame "None", Default {
              }
              frame "ALL" {
              }
            }
            n627 = call-poly "Set All Plot Visibility.vi"("error in (no error)"=w1286, "All Visible?"=w1279, "WFGraph in"=w1274) -> ("error out"=w1287:errorcluster)  [unwired: 8 in]
            n628 = call-poly "Set All Plot Visibility.vi"("error in (no error)"=w1287, "All Visible?"=w1279, "WFGraph in"=w1275) -> ("error out"=w1283:errorcluster)  [unwired: 8 in]
            n629 = call-poly "Set All Plot Visibility.vi"("error in (no error)"=w1283, "All Visible?"=w1279, "XYGraph in"=w1278) -> ("error out"=w1282:errorcluster)  [unwired: 7 in, 1 out]
            n630 = call-poly "Set All Plot Visibility.vi"("error in (no error)"=w1282, "All Visible?"=w1279, "WFGraph in"=w1277) -> ("error out"=w1281:errorcluster)  [unwired: 8 in]
            n631 = call-poly "Set All Plot Visibility.vi"("error in (no error)"=w1281, "All Visible?"=w1279, "WFGraph in"=w1276) -> ("error out"=w1280:errorcluster)  [unwired: 8 in]
            n632 = call <vilib>:"Add State(s) to Queue__jki_lib_state_machine.vi"("State(s) in (\"\")"=w1290) -> ("States Out"=w1289:string)  [unwired: 14 in]
          }
          frame "UI: Get Plot Visibility" {
            n633 = Unbundle By Name(w1305) -> ("References.Graphs.AI Graph"=w1302:refnum<vi>, "References.Graphs.AO Graph"=w1301:refnum<vi>, "References.Graphs.Lockin 1"=w1303:refnum<vi>)
            n634 = call-poly "Get Plot Visibility.vi"("error in (no error)"=w1296, "WFGraph in"=w1302) -> ("error out"=w1297:errorcluster, "Plot.Visible"=w1295:bool[])  [unwired: 8 in]
            n635 = call-poly "Get Plot Visibility.vi"("error in (no error)"=w1296, "WFGraph in"=w1303) -> ("error out"=w1300:errorcluster, "Plot.Visible"=w1293:bool[])  [unwired: 8 in]
            n636 = call-poly "Get Plot Visibility.vi"("error in (no error)"=w1296, "WFGraph in"=w1301) -> ("error out"=w1298:errorcluster, "Plot.Visible"=w1294:bool[])  [unwired: 8 in]
            n637 = Bundle By Name(cluster=w1305, "UI Config.Plot.visibility.AI"=w1295, "UI Config.Plot.visibility.AO"=w1294, "UI Config.Plot.visibility.Lockin"=w1293) -> (w1304:T65)
            n638 = Merge Errors(w1296, w1297, w1298, w1300) -> (w1299:errorcluster)
            n639 = call <vilib>:"Add State(s) to Queue__jki_lib_state_machine.vi"("State(s) in (\"\")"=w1308) -> ("States Out"=w1307:string)  [unwired: 14 in]
          }
          frame "UI: Set Plot Visibility" {
            n640 = Unbundle By Name(w1312) -> ("References.Graphs.AI Graph"=w1319:refnum<vi>, "UI Config.Plot.visibility.AI"=w1310:bool[], "References.Graphs.AO Graph"=w1318:refnum<vi>, "UI Config.Plot.visibility.AO"=w1311:bool[], "References.Graphs.Lockin 1"=w1320:refnum<vi>, "UI Config.Plot.visibility.Lockin"=w1309:bool[])
            n641 = call-poly "Set Plot Visibility.vi"("error in (no error)"=w1313, "Plot.Visible?"=w1310, "WFGraph in"=w1319) -> ("error out"=w1314:errorcluster)  [unwired: 8 in]
            n642 = call-poly "Set Plot Visibility.vi"("error in (no error)"=w1313, "Plot.Visible?"=w1311, "WFGraph in"=w1318) -> ("error out"=w1315:errorcluster)  [unwired: 8 in]
            n643 = call-poly "Set Plot Visibility.vi"("error in (no error)"=w1313, "Plot.Visible?"=w1309, "WFGraph in"=w1320) -> ("error out"=w1317:errorcluster)  [unwired: 8 in]
            n644 = Merge Errors(w1314, w1315, w1317) -> (w1316:errorcluster)
            n645 = call <vilib>:"Add State(s) to Queue__jki_lib_state_machine.vi"("State(s) in (\"\")"=w1323) -> ("States Out"=w1322:string)  [unwired: 14 in]
          }
          frame "UI: Sync AI Plot Visibility" {
            n646 = Unbundle By Name(w1333) -> ("References.Graphs.PS WFGraph"=w1329:refnum<vi>, "References.Graphs.Sweep AI Graph"=w1330:refnum<vi>, "References.Graphs.AI Graph"=w1331:refnum<vi>)
            n647 = call-poly "Get Plot Visibility.vi"("error in (no error)"=w1325, "WFGraph in"=w1331) -> ("error out"=w1328:errorcluster, "Plot.Visible"=w1326:bool[])  [unwired: 8 in]
            n648 = call-poly "Set Plot Visibility.vi"("error in (no error)"=w1328, "Plot.Visible?"=w1326, "WFGraph in"=w1330) -> ("error out"=w1324:errorcluster)  [unwired: 8 in]
            n649 = call-poly "Set Plot Visibility.vi"("error in (no error)"=w1325, "Plot.Visible?"=w1326, "WFGraph (WDT) in"=w1329) -> ("error out"=w1327:errorcluster)  [unwired: 8 in]
            n650 = Merge Errors(w1324, w1327) -> (w1332:errorcluster)
            n651 = call <vilib>:"Add State(s) to Queue__jki_lib_state_machine.vi"("State(s) in (\"\")"=w1336) -> ("States Out"=w1335:string)  [unwired: 14 in]
          }
          frame "UI: Sync AO Plot Visibility" {
            n652 = Unbundle By Name(w1344) -> ("References.Graphs.Sweep AO Graph"=w1343:refnum<vi>, "References.Graphs.AO Graph"=w1341:refnum<vi>)
            n653 = call-poly "Get Plot Visibility.vi"("error in (no error)"=w1339, "WFGraph in"=w1341) -> ("error out"=w1337:errorcluster, "Plot.Visible"=w1338:bool[])  [unwired: 8 in]
            n654 = call-poly "Set Plot Visibility.vi"("error in (no error)"=w1337, "Plot.Visible?"=w1338, "WFGraph in"=w1343) -> ("error out"=w1340:errorcluster)  [unwired: 8 in]
            n655 = Merge Errors(w1340) -> (w1342:errorcluster)
            n656 = call <vilib>:"Add State(s) to Queue__jki_lib_state_machine.vi"("State(s) in (\"\")"=w1347) -> ("States Out"=w1346:string)  [unwired: 14 in]
          }
          frame "UI: Sync Lockin Plot Visibility" {
            # "Do not put any code in this frame.\n(It is a separator no-op. You can make a copy of this frame to create a new UI frame)"
            n657 = Unbundle By Name(w1361) -> ("References.Graphs.Sweep X Graph"=w1355:refnum<vi>, "References.Graphs.Sweep Y Graph"=w1356:refnum<vi>, "References.Graphs.Lockin XY"=w1357:refnum<vi>, "References.Graphs.Lockin 2"=w1360:refnum<vi>, "References.Graphs.Lockin 1"=w1358:refnum<vi>)
            n658 = call-poly "Get Plot Visibility.vi"("error in (no error)"=w1349, "WFGraph in"=w1358) -> ("error out"=w1350:errorcluster, "Plot.Visible"=w1348:bool[])  [unwired: 8 in]
            n659 = call-poly "Set Plot Visibility.vi"("error in (no error)"=w1350, "Plot.Visible?"=w1348, "WFGraph in"=w1360) -> ("error out"=w1351:errorcluster)  [unwired: 8 in]
            n660 = call-poly "Set Plot Visibility.vi"("error in (no error)"=w1350, "Plot.Visible?"=w1348, "XYGraph in"=w1357) -> ("error out"=w1352:errorcluster)  [unwired: 8 in]
            n661 = call-poly "Set Plot Visibility.vi"("error in (no error)"=w1350, "Plot.Visible?"=w1348, "WFGraph in"=w1356) -> ("error out"=w1353:errorcluster)  [unwired: 8 in]
            n662 = call-poly "Set Plot Visibility.vi"("error in (no error)"=w1350, "Plot.Visible?"=w1348, "WFGraph in"=w1355) -> ("error out"=w1354:errorcluster)  [unwired: 8 in]
            n663 = Merge Errors(w1354, w1353, w1352, w1351) -> (w1359:errorcluster)
            n664 = call <vilib>:"Add State(s) to Queue__jki_lib_state_machine.vi"("State(s) in (\"\")"=w1364) -> ("States Out"=w1363:string)  [unwired: 14 in]
          }
          frame "UI: Update Waveform Graphs" {
            n665 = Unbundle By Name(w1395) -> ("UI Config.DAQ.cfg.Sampling.Sampling"=w1382:T49, "UI Config.Amplifers.Gain_AI"=w1388:T17, "getAll.Waveforms.AI"=w1376:waveform(dbl)[], "getAll.Waveforms.AO"=w1377:waveform(dbl)[], "getAll.Waveforms.REF_X"=w1378:waveform(dbl)[], "getAll.Waveforms.REF_Y"=w1386:waveform(dbl)[])
            n666 = Decrement(x="Sync Ch") -> (x-1=w1383:i32)
            n667 = for {
              tunnel: w1388 -> [w1429] mode=indexing
              tunnel: [w1428] -> w1387 mode=indexing
              n668 = Unbundle By Name(w1429) -> ("Gain"=w1428:dbl)
            }
            n669 = Interleave 1D Arrays(w1378, w1386) -> (w1375:waveform(dbl)[])
            n670 = case shown="True" "Sync?" {
              tunnel: [w1405 w1426] -> w1372
              tunnel: w1376 -> [w1405 w1425]
              tunnel: w1377 -> [w1403 w1424]
              tunnel: [w1404 w1423] -> w1373
              tunnel: [w1402 w1422] -> w1370
              tunnel: [w1403 w1421] -> w1369
              tunnel: w1374 -> [w1402 w1420]
              tunnel: w1375 -> [w1401 w1419]
              tunnel: w1374 -> [w1400 w1418]
              tunnel: [w1400 w1417] -> w1368
              tunnel: [w1401 w1416] -> w1367
              tunnel: w1383 -> [_ w1415]
              tunnel: w1374 -> [w1404 w1414]
              tunnel: w1382 -> [_ w1413]
              tunnel: [_ w1411] -> w1380
              tunnel: [_ w1409] -> w1379
              tunnel: w1378 -> [_ w1406]
              frame False {
              }
              frame True {
                n671 = Index Array(array=w1406, index=w1415) -> (element=w1427:waveform(dbl))
                n672 = call-poly <vilib>:"Extract Single Tone Information.vi"("time signal in"=w1427) -> ("detected phase (deg)"=w1410:dbl, "detected frequency"=w1412:dbl)  [unwired: 5 in, 4 out]
                n673 = Format Into String(format string="%.1f (Hz)", w1412) -> (resulting string=w1411:string)  [unwired: 2 in, 1 out]
                n674 = Format Into String(format string="%.0f (°)", w1410) -> (resulting string=w1409:string)  [unwired: 2 in, 1 out]
                n675 = call "Display Synchronous.vi"("Sampling"=w1413, "error in (no error)"=w1414, "phase (°)"=w1410, "frequency (Hz)"=w1412, "Input Waveforms"=w1425) -> ("error out"=w1423:errorcluster, "Output Waveforms"=w1426:waveform(dbl)[])  [unwired: 5 in]
                n676 = call "Display Synchronous.vi"("Sampling"=w1413, "error in (no error)"=w1420, "phase (°)"=w1410, "frequency (Hz)"=w1412, "Input Waveforms"=w1424) -> ("error out"=w1422:errorcluster, "Output Waveforms"=w1421:waveform(dbl)[])  [unwired: 5 in]
                n677 = call "Display Synchronous.vi"("Sampling"=w1413, "error in (no error)"=w1418, "phase (°)"=w1410, "frequency (Hz)"=w1412, "Input Waveforms"=w1419) -> ("error out"=w1417:errorcluster, "Output Waveforms"=w1416:waveform(dbl)[])  [unwired: 5 in]
              }
            }
            "phi (°)" <- w1379
            "f (Hz)" <- w1380
            n678 = local read "X Scale"() -> (w1366:enum16{"time", "samples"})
            n679 = call "Display n or dt.vi"("error in (no error)"=w1368, "X Scale"=w1366, "Input Waveforms"=w1367) -> ("error out"=w1365:errorcluster, "Output Waveforms"=→"REF Graph":waveform(dbl)[])  [unwired: 7 in]
            n680 = call "Display n or dt.vi"("error in (no error)"=w1373, "X Scale"=w1366, "Input Waveforms"=w1372) -> ("error out"=w1396:errorcluster, "Output Waveforms"=w1371:waveform(dbl)[])  [unwired: 7 in]
            n681 = call "Display n or dt.vi"("error in (no error)"=w1370, "X Scale"=w1366, "Input Waveforms"=w1369) -> ("error out"=w1391:errorcluster, "Output Waveforms"=→"AO Graph":waveform(dbl)[])  [unwired: 7 in]
            n682 = local read "Input"() -> (w1394:enum16{"Device", "ADC"})
            n683 = case shown="\"ADC\"" w1394 {
              tunnel: w1371 -> [w1431 w1436]
              tunnel: w1387 -> [_ w1434]
              tunnel: [w1431 w1435] -> w1390
              tunnel: w1396 -> [w1430 w1433]
              tunnel: [w1430 w1432] -> w1392
              frame "Device", Default {
              }
              frame "ADC" {
                n684 = call "Multiply by Gain.vi"("error in (no error)"=w1433, "Gain"=w1434, "WFM in"=w1436) -> ("error out"=w1432:errorcluster, "WFM out"=w1435:waveform(dbl)[])  [unwired: 7 in]
              }
            }
            "AI Graph" <- w1390
            n685 = Merge Errors(w1392, w1391, w1365) -> (w1393:errorcluster)
            n686 = call <vilib>:"Add State(s) to Queue__jki_lib_state_machine.vi"("State(s) in (\"\")"=w1399) -> ("States Out"=w1398:string)  [unwired: 14 in]
          }
          frame "UI: Update AI Waveform Graphs Legends" {
            # "Do not put any code in this frame.\n(It is a separator no-op. You can make a copy of this frame to create a new UI frame)"
            n687 = Unbundle By Name(w1446) -> ("References.Graphs.AI Graph"=w1438:refnum<vi>, "References.Graphs.Sweep AI Graph"=w1437:refnum<vi>, "UI Config.DAQ.Configuration"=w1444:T9)
            n688 = call "Get AI StringsAndValues.vi"("error in (no error)"=w1443, "Configuration.DAQ"=w1444) -> ("error out"=w1441:errorcluster, "Strings"=w1442:string[])  [unwired: 7 in, 1 out]
            n689 = call-poly "Set Legend.vi"("error in (no error)"=w1441, "Plot.Plot Name"=w1442, "WFGraph in"=w1437) -> ("error out"=w1439:errorcluster)  [unwired: 8 in]
            n690 = call-poly "Set Legend.vi"("error in (no error)"=w1441, "Plot.Plot Name"=w1442, "WFGraph in"=w1438) -> ("error out"=w1440:errorcluster)  [unwired: 8 in]
            n691 = Merge Errors(w1440, w1439) -> (w1445:errorcluster)
            n692 = call <vilib>:"Add State(s) to Queue__jki_lib_state_machine.vi"("State(s) in (\"\")"=w1449) -> ("States Out"=w1448:string)  [unwired: 14 in]
          }
          frame "UI: Update AI Waveform Graphs Colors" {
            # "Do not put any code in this frame.\n(It is a separator no-op. You can make a copy of this frame to create a new UI frame)"
            n693 = Unbundle By Name(w1460) -> ("References.Graphs.PS WFGraph"=w1456:refnum<vi>, "References.Graphs.AI Graph"=w1457:refnum<vi>, "References.Graphs.Sweep AI Graph"=w1458:refnum<vi>)
            n694 = call-poly "Set Plot Color.vi"("error in (no error)"=w1451, "WFGraph in"=w1458) -> ("error out"=w1453:errorcluster)  [unwired: 9 in]
            n695 = call-poly "Set Plot Color.vi"("error in (no error)"=w1451, "WFGraph in"=w1457) -> ("error out"=w1454:errorcluster)  [unwired: 9 in]
            n696 = call-poly "Set Plot Color.vi"("error in (no error)"=w1451, "WFGraph (WDT) in"=w1456) -> ("error out"=w1455:errorcluster)  [unwired: 9 in]
            n697 = control-ref of="PS Chart"() -> (w1452:refnum<vi>)
            n698 = call-poly "Set Plot Color.vi"("error in (no error)"=w1451, "PS Chart 2"=w1452) -> ("error out"=w1450:errorcluster)  [unwired: 9 in]
            n699 = Merge Errors(w1450, w1455, w1454, w1453) -> (w1459:errorcluster)
            n700 = call <vilib>:"Add State(s) to Queue__jki_lib_state_machine.vi"("State(s) in (\"\")"=w1463) -> ("States Out"=w1462:string)  [unwired: 14 in]
          }
          frame "UI: Update AO Waveform Graphs Legends" {
            n701 = Unbundle By Name(w1473) -> ("References.Graphs.AO Graph"=w1471:refnum<vi>, "References.Graphs.Sweep AO Graph"=w1470:refnum<vi>, "UI Config.DAQ.Configuration"=w1467:T9)
            n702 = call "Get AO StringsAndValues.vi"("error in (no error)"=w1464, "Configuration.DAQ"=w1467) -> ("error out"=w1465:errorcluster, "Strings"=w1466:string[])  [unwired: 7 in, 1 out]
            n703 = call-poly "Set Legend.vi"("error in (no error)"=w1465, "Plot.Plot Name"=w1466, "WFGraph in"=w1470) -> ("error out"=w1468:errorcluster)  [unwired: 8 in]
            n704 = call-poly "Set Legend.vi"("error in (no error)"=w1465, "Plot.Plot Name"=w1466, "WFGraph in"=w1471) -> ("error out"=w1469:errorcluster)  [unwired: 8 in]
            n705 = Merge Errors(w1469, w1468) -> (w1472:errorcluster)
            n706 = call <vilib>:"Add State(s) to Queue__jki_lib_state_machine.vi"("State(s) in (\"\")"=w1476) -> ("States Out"=w1475:string)  [unwired: 14 in]
          }
          frame "UI: Update REF Waveform Graphs Legends" {
            n707 = Unbundle By Name(w1484) -> ("References.Graphs.REF Graph"=w1482:refnum<vi>, "UI Config.Channels.Cfg_REF"=w1483:T2)
            n708 = call "Get AI REF StringsAndValues.vi"("error in (no error)"=w1478, "Channels.REF"=w1483) -> ("error out"=w1481:errorcluster, "Strings"=w1479:string[])  [unwired: 7 in, 1 out]
            n709 = for {
              tunnel: [w1493] -> w1480 mode=concatenating
              tunnel: w1479 -> [w1488] mode=indexing
              n710 = Concatenate Strings(w1488, " X" ("string")) -> (w1492:string)
              n711 = Concatenate Strings(w1488, " Y" ("string")) -> (w1489:string)
              n712 = Build Array(w1492, w1489) -> (w1493:string[])
            }
            n713 = call-poly "Set Legend.vi"("error in (no error)"=w1481, "Plot.Plot Name"=w1480, "WFGraph in"=w1482) -> ("error out"=w1477:errorcluster)  [unwired: 8 in]
            n714 = call <vilib>:"Add State(s) to Queue__jki_lib_state_machine.vi"("State(s) in (\"\")"=w1487) -> ("States Out"=w1486:string)  [unwired: 14 in]
          }
          frame "UI: Update AO Waveform Graphs Colors" {
            n715 = Unbundle By Name(w1500) -> ("References.Graphs.AO Graph"=w1497:refnum<vi>, "References.Graphs.Sweep AO Graph"=w1498:refnum<vi>)
            n716 = call-poly "Set Plot Color.vi"("error in (no error)"=w1494, "WFGraph in"=w1498) -> ("error out"=w1495:errorcluster)  [unwired: 9 in]
            n717 = call-poly "Set Plot Color.vi"("error in (no error)"=w1494, "WFGraph in"=w1497) -> ("error out"=w1496:errorcluster)  [unwired: 9 in]
            n718 = Merge Errors(w1494, w1496, w1495) -> (w1499:errorcluster)
            n719 = call <vilib>:"Add State(s) to Queue__jki_lib_state_machine.vi"("State(s) in (\"\")"=w1503) -> ("States Out"=w1502:string)  [unwired: 14 in]
          }
          frame "UI: Update REF Waveform Graphs Colors" {
            n720 = Unbundle By Name(w1507) -> ("References.Graphs.REF Graph"=w1506:refnum<vi>)
            n721 = call-poly "Set Plot Color.vi"("error in (no error)"=w1504, "WFGraph in"=w1506) -> ("error out"=w1505:errorcluster)  [unwired: 9 in]
            n722 = call <vilib>:"Add State(s) to Queue__jki_lib_state_machine.vi"("State(s) in (\"\")"=w1510) -> ("States Out"=w1509:string)  [unwired: 14 in]
          }
          frame "UI: Show Hide AO Waveform Graphs" {
            n723 = Unbundle By Name(w1521) -> ("References.Graphs.REF Graph"=w1518:refnum<vi>, "References.Graphs.AO Graph"=w1519:refnum<vi>)
            n724 = local read "Output"() -> (w1517:enum16{"AO", "REF"})
            n725 = Equal?(x=w1517, y=enum16{"Analog Output", "Reference"}."Analog Output" ("Y Axis (Output)")) -> (x = y?=w1512:bool)
            n726 = property on="AO Graph None" class="Bool"("Visible"=w1512) -> ()  [unwired: 2 in, 2 out]
            n727 = property on="AO Graph All" class="Bool"("Visible"=w1512) -> ()  [unwired: 2 in, 2 out]
            n728 = property class="WFGraph (strict)"(reference=w1519, "Visible"=w1512) -> (error out=w1515:errorcluster)  [unwired: 1 in, 1 out]
            n729 = Not(x=w1512) -> (.not. x?=w1511:bool)
            n730 = property class="WFGraph (strict)"(reference=w1518, "Visible"=w1511) -> (error out=w1516:errorcluster)  [unwired: 1 in, 1 out]
            n731 = property on="REF Graph None" class="Bool (strict)"("Visible"=w1511) -> ()  [unwired: 2 in, 2 out]
            n732 = property on="REF Graph All" class="Bool (strict)"("Visible"=w1511) -> ()  [unwired: 2 in, 2 out]
            n733 = Merge Errors(w1513, w1516, w1515) -> (w1520:errorcluster)
            n734 = call <vilib>:"Add State(s) to Queue__jki_lib_state_machine.vi"("State(s) in (\"\")"=w1524) -> ("States Out"=w1523:string)  [unwired: 14 in]
          }
          frame "UI: Update Waveform Graph Labels" {
            n735 = Unbundle By Name(w1538) -> ("References.Graphs.REF Graph"=w1532:refnum<vi>, "References.Graphs.AO Graph"=w1536:refnum<vi>, "References.Graphs.AI Graph"=w1537:refnum<vi>)
            n736 = local read "X Scale"() -> (w1525:enum16{"time", "samples"})
            n737 = call "Set AO AI Graph X Axis (WFGraph).vi"("error in (no error)"=w1526, "X Axis"=w1525, "WaveformGraph in"=w1537) -> ("error out"=w1527:errorcluster)  [unwired: 8 in]
            n738 = call "Set AO AI Graph X Axis (WFGraph).vi"("error in (no error)"=w1526, "X Axis"=w1525, "WaveformGraph in"=w1536) -> ("error out"=w1530:errorcluster)  [unwired: 8 in]
            n739 = call "Set AO Graph Y Axis (WFGraph).vi"("error in (no error)"=w1530, "Y Axis (Output)"=enum16{"Analog Output", "Reference"}."Analog Output", "WaveformGraph in"=w1536) -> ("error out"=w1528:errorcluster)  [unwired: 8 in]
            n740 = call "Set AO AI Graph X Axis (WFGraph).vi"("error in (no error)"=w1526, "X Axis"=w1525, "WaveformGraph in"=w1532) -> ("error out"=w1531:errorcluster)  [unwired: 8 in]
            n741 = call "Set AO Graph Y Axis (WFGraph).vi"("error in (no error)"=w1531, "Y Axis (Output)"=enum16{"Analog Output", "Reference"}."Reference", "WaveformGraph in"=w1532) -> ("error out"=w1529:errorcluster)  [unwired: 8 in]
            n742 = Merge Errors(w1529, w1528, w1527) -> (w1533:errorcluster)
            n743 = call <vilib>:"Add State(s) to Queue__jki_lib_state_machine.vi"("State(s) in (\"\")"=w1541) -> ("States Out"=w1540:string)  [unwired: 14 in]
          }
          frame "UI: Init Graph Data" {
            # "UI: Init Graph Data.\n(IInitialize graphs with data before changing their properties)"
            n744 = Unbundle By Name(w1562) -> ("UI Config.DAQ.Configuration"=w1561:T9, "UI Config.Channels.Cfg_REF"=w1560:T2, "UI Config.Plot.visibility.AI"=w1555:bool[], "UI Config.Plot.visibility.AO"=w1554:bool[], "UI Config.Plot.visibility.Lockin"=w1553:bool[])
            n745 = call "Get AI StringsAndValues.vi"("Configuration.DAQ"=w1561) -> ()  [unwired: 8 in, 3 out]
            n746 = call "Get AO StringsAndValues.vi"("Configuration.DAQ"=w1561) -> ()  [unwired: 8 in, 3 out]
            n747 = call "Get AI REF StringsAndValues.vi"("Channels.REF"=w1560) -> ("Strings"=w1545:string[])  [unwired: 8 in, 2 out]
            n748 = Array Size(array=w1545) -> (size(s)=w1543:i32)
            n749 = Array Size(array=w1555) -> (size(s)=w1552:i32)
            n750 = Array Size(array=w1554) -> (size(s)=w1551:i32)
            n751 = Array Size(array=w1553) -> (size(s)=w1549:i32)
            n752 = Get Date/Time In Seconds() -> (seconds since 1Jan1904=w1559:timestamp)
            n753 = Multiply(x=w1543, y=2) -> (x*y=w1542:i32)
            n754 = Bundle By Name("t0"=w1559) -> (w1547:waveform(dbl))  [unwired: 1 in]
            n755 = Initialize Array(w1547, w1542) -> (w1546:waveform(dbl)[])
            n756 = Initialize Array(w1547, w1552) -> (w1558:waveform(dbl)[])
            n757 = Initialize Array(w1547, w1551) -> (w1557:waveform(dbl)[])
            n758 = Initialize Array(w1547, w1549) -> (w1556:waveform(dbl)[])
            n759 = Initialize Array(cluster{"Wavenumber":dbl[], "Data":dbl[]} {"Wavenumber"=[0.0], "Data"=[0.0]} ("Lockin XY"), w1549) -> (w1548:cluster{"Wavenumber":dbl[], "Data":dbl[]}[])
            n760 = local write "REF Graph"(w1546) -> ()
            n761 = local write "AI Graph"(w1558) -> ()
            n762 = local write "AO Graph"(w1557) -> ()
            n763 = local write "Lockin 1"(w1556) -> ()
            n764 = local write "Lockin 2"(w1556) -> ()
            n765 = local write "Lockin XY"(w1548) -> ()
            n766 = call <vilib>:"Add State(s) to Queue__jki_lib_state_machine.vi"("State(s) in (\"\")"=w1566) -> ("States Out"=w1565:string)  [unwired: 14 in]
          }
          frame "UI: Init Graph Legends" {
            # "Do not put any code in this frame.\n(It is a separator no-op. You can make a copy of this frame to create a new UI frame)"
            n767 = Unbundle By Name(w1579) -> ("References.Graphs.AI Graph"=w1578:refnum<vi>, "References.Graphs.AO Graph"=w1577:refnum<vi>, "References.Graphs.REF Graph"=w1576:refnum<vi>, "References.Graphs.Lockin 1"=w1568:refnum<vi>, "References.Graphs.Lockin 2"=w1567:refnum<vi>, "References.Graphs.Lockin XY"=w1575:refnum<vi>, "References.Graphs.Sweep X Graph"=w1574:refnum<vi>, "References.Graphs.Sweep Y Graph"=w1573:refnum<vi>, "References.Graphs.Sweep AI Graph"=w1572:refnum<vi>, "References.Graphs.Sweep AO Graph"=w1571:refnum<vi>, "References.Graphs.PS WFGraph"=w1570:refnum<vi>)  [unwired: 1 out]
            n768 = Build Array(w1578, w1577, w1576, w1568, w1567, w1575, w1574, w1573, w1572, w1571, w1570) -> (w1580:refnum<vi>[])
            n769 = for {
              tunnel: w1580 -> [w1586] mode=indexing
              tunnel: u32 142 ("Legend:Size:Width") -> [w1585]
              n770 = property on="Property Node" class="WFGraph"(reference=w1586, "LegWidth"=w1585) -> ()  [unwired: 1 in, 2 out]
            }
            n771 = call <vilib>:"Add State(s) to Queue__jki_lib_state_machine.vi"("State(s) in (\"\")"=w1584) -> ("States Out"=w1583:string)  [unwired: 14 in]
          }
          frame "UI: Update Lockin Graphs" {
            # "data used in PS"
            n772 = Unbundle By Name(w1594) -> ("clear lockin charts"=w1588:bool, "UI Config.DAQ.cfg.Sampling.Fs.Output"=w1593:dbl, "getAll.Results.Results (Dictionary)"=w1609:cluster{"key":string, "value":dbl[]}[], "UI Config.DAQ.Configuration"=w1608:T9, "UI Config.Amplifers.Gain_AI"=w1607:T17)
            n773 = call "Parse Results (table).vi"("error in (no error)"=w1615, "Input Gain"=w1607, "DAQ Config"=w1608, "Results (Dictionary)"=w1609) -> ("error out"=w1613:errorcluster, "Table"=→"Results":string[][], "Results (Dictionary) out"=w1611:cluster{"key":string, "value":dbl[]}[])  [unwired: 5 in]
            n774 = local read "Display 1"() -> (w1596:T26)
            n775 = local read "Display 2"() -> (w1597:T26)
            n776 = call "Dictionary to Chart.vi"("reset"=w1588, "error in (no error)"=w1613, "Fs.Output (S/s)"=w1593, "Results (Dictionary)"=w1611) -> ("error out"=w1599:errorcluster, "Waveform Graph"=w1591:waveform(dbl)[][], "Results (Dictionary) out"=w1600:cluster{"key":string, "value":dbl[]}[])  [unwired: 5 in]
            n777 = Index Array(array=w1591, index (row) #1=w1596, index (row) #2=w1597) -> (element #1=→"Lockin 1":waveform(dbl)[], element #2=→"Lockin 2":waveform(dbl)[])  [unwired: 2 in]
            n778 = Bundle By Name(cluster=w1594, "clear lockin charts"=FALSE, "Waveform Charts"=w1591) -> (w1595:T65)
            n779 = local read "channel-reference"() -> (w1598:u16)
            n780 = call "Dictionary to XY Graph.vi"("error in (no error)"=w1599, "Results (Dictionary)"=w1600) -> ("error out"=w1605:errorcluster, "XY Graph"=→"Lockin XY":cluster{dbl[], dbl[]}[], "Results (Dictionary) out"=w1606:cluster{"key":string, "value":dbl[]}[])  [unwired: 7 in]
            n781 = call "Dictionary to Indicator.vi"("Results (Dictionary)"=w1606, "AI Channel"=w1598, "error in (no error)"=w1605) -> ("X"=→"X (V)":dbl, "Y"=→"Y (V)":dbl, "R"=→"R (V)":dbl, "Theta"=→"theta (°)":dbl, "Mean"=→"mean (V)":dbl, "error out"=w1614:errorcluster)  [unwired: 7 in]
            n782 = call <vilib>:"Add State(s) to Queue__jki_lib_state_machine.vi"("State(s) in (\"\")"=w1618) -> ("States Out"=w1617:string)  [unwired: 14 in]
          }
          frame "UI: Update Lockin Graphs Legends" {
            n783 = Unbundle By Name(w1627) -> ("References.Graphs.Sweep X Graph"=w1639:refnum<vi>, "References.Graphs.Sweep Y Graph"=w1638:refnum<vi>, "References.Graphs.Lockin XY"=w1637:refnum<vi>, "References.Graphs.Lockin 2"=w1636:refnum<vi>, "References.Graphs.Lockin 1"=w1634:refnum<vi>)
            n784 = Unbundle By Name(w1627) -> ("UI Config.DAQ.Configuration"=w1629:T9, "UI Config.Channels.Cfg_REF"=w1628:T2)
            n785 = call "Get AI REF StringsAndValues.vi"("error in (no error)"=w1622, "Channels.REF"=w1628) -> ("error out"=w1623:errorcluster, "Strings"=w1625:string[])  [unwired: 7 in, 1 out]
            n786 = call "Get AI StringsAndValues.vi"("error in (no error)"=w1623, "Configuration.DAQ"=w1629) -> ("error out"=w1621:errorcluster, "Strings"=w1626:string[])  [unwired: 7 in, 1 out]
            n787 = call <vilib>:"Space Constant.vi"() -> ("String"=w1620:string)
            n788 = for {
              tunnel: w1626 -> [w1645]
              tunnel: w1625 -> [w1646] mode=indexing
              tunnel: [w1644] -> w1624 mode=concatenating
              tunnel: w1620 -> [w1643]
              n789 = for {
                tunnel: w1646 -> [w1649]
                tunnel: w1645 -> [w1648] mode=indexing
                tunnel: [w1650] -> w1644 mode=indexing
                tunnel: w1643 -> [w1647]
                n790 = Concatenate Strings(w1648, w1647, w1649) -> (w1650:string)
              }
            }
            n791 = call-poly "Set Legend.vi"("error in (no error)"=w1621, "Plot.Plot Name"=w1624, "WFGraph in"=w1634) -> ("error out"=w1630:errorcluster)  [unwired: 8 in]
            n792 = call-poly "Set Legend.vi"("error in (no error)"=w1621, "Plot.Plot Name"=w1624, "WFGraph in"=w1636) -> ("error out"=w1631:errorcluster)  [unwired: 8 in]
            n793 = call-poly "Set Legend.vi"("error in (no error)"=w1621, "Plot.Plot Name"=w1624, "XYGraph in"=w1637) -> ("error out"=w1632:errorcluster)  [unwired: 8 in]
            n794 = call-poly "Set Legend.vi"("error in (no error)"=w1621, "Plot.Plot Name"=w1624, "WFGraph in"=w1638) -> ("error out"=w1633:errorcluster)  [unwired: 8 in]
            n795 = call-poly "Set Legend.vi"("error in (no error)"=w1621, "Plot.Plot Name"=w1624, "WFGraph in"=w1639) -> ("error out"=w1619:errorcluster)  [unwired: 8 in]
            n796 = Merge Errors(w1619, w1633, w1632, w1631, w1630) -> (w1635:errorcluster)
            n797 = call <vilib>:"Add State(s) to Queue__jki_lib_state_machine.vi"("State(s) in (\"\")"=w1642) -> ("States Out"=w1641:string)  [unwired: 14 in]
          }
          frame "UI: Update Lockin Graphs Colors" {
            n798 = Unbundle By Name(w1663) -> ("References.Graphs.Sweep X Graph"=w1662:refnum<vi>, "References.Graphs.Sweep Y Graph"=w1661:refnum<vi>, "References.Graphs.Lockin XY"=w1651:refnum<vi>, "References.Graphs.Lockin 2"=w1660:refnum<vi>, "References.Graphs.Lockin 1"=w1659:refnum<vi>)
            n799 = call-poly "Set Plot Color.vi"("error in (no error)"=w1652, "WFGraph in"=w1659) -> ("error out"=w1653:errorcluster)  [unwired: 9 in]
            n800 = call-poly "Set Plot Color.vi"("error in (no error)"=w1652, "WFGraph in"=w1660) -> ("error out"=w1654:errorcluster)  [unwired: 9 in]
            n801 = call-poly "Set Plot Color.vi"("error in (no error)"=w1652, "XYGraph in"=w1651) -> ("error out"=w1655:errorcluster)  [unwired: 9 in]
            n802 = call-poly "Set Plot Color.vi"("error in (no error)"=w1652, "WFGraph in"=w1661) -> ("error out"=w1656:errorcluster)  [unwired: 9 in]
            n803 = call-poly "Set Plot Color.vi"("error in (no error)"=w1652, "WFGraph in"=w1662) -> ("error out"=w1657:errorcluster)  [unwired: 9 in]
            n804 = while {
              tunnel: w1651 -> [w1670]
              i -> [w1668]
              stop <- w1669 stop-if-true
              n805 = property on="Property Node" class="XYGraph (strict)"(reference=w1670, "Active Plot"=w1668, "Plot.Point Style"=u8 1) -> (error out=w1669:errorcluster)  [unwired: 1 in, 1 out]
            }
            n806 = Merge Errors(w1657, w1656, w1655, w1654, w1653) -> (w1658:errorcluster)
            n807 = call <vilib>:"Add State(s) to Queue__jki_lib_state_machine.vi"("State(s) in (\"\")"=w1666) -> ("States Out"=w1665:string)  [unwired: 14 in]
          }
          frame "UI: Update Lockin Graph Range" {
            # "xy"
            # "2"
            # "1"
            # "Do not put any code in this frame.\n(It is a separator no-op. You can make a copy of this frame to create a new UI frame)"
            n808 = Unbundle By Name(w1678) -> ("References.Graphs.Lockin 1"=w1675:refnum<vi>, "References.Graphs.Lockin 2"=w1674:refnum<vi>, "References.Graphs.Lockin XY"=w1673:refnum<vi>)
            n809 = Negate(x="X/R Range") -> (-x=w1679:dbl)
            n810 = Negate(x="Y/Theta Range") -> (-x=w1680:dbl)
            n811 = Negate(x="XY Range") -> (-x=w1672:dbl)
            n812 = property on="Property Node" class="WFGraph (strict)"(reference=w1675, "YScale.Maximum"="X/R Range", "YScale.Minimum"=w1679) -> ()  [unwired: 1 in, 2 out]
            n813 = property on="Property Node" class="WFGraph (strict)"(reference=w1674, "YScale.Maximum"="Y/Theta Range", "YScale.Minimum"=w1680) -> ()  [unwired: 1 in, 2 out]
            n814 = property on="Property Node" class="XYGraph (strict)"(reference=w1673, "XScale.Maximum"="XY Range", "YScale.Maximum"="XY Range", "XScale.Minimum"=w1672, "YScale.Minimum"=w1672) -> ()  [unwired: 1 in, 2 out]
            n815 = call <vilib>:"Add State(s) to Queue__jki_lib_state_machine.vi"("State(s) in (\"\")"=w1684) -> ("States Out"=w1683:string)  [unwired: 14 in]
          }
          frame "UI: Update Lockin Graph Labels" {
            n816 = local read "Display 1"() -> (w1691:T26)
            n817 = local read "Display 2"() -> (w1685:T26)
            n818 = Unbundle By Name(w1687) -> ("References.Graphs.Lockin 1"=w1689:refnum<vi>, "References.Graphs.Lockin 2"=w1688:refnum<vi>)
            n819 = case shown="\"Mean\"" w1691 {
              tunnel: ["Lockin X (A or V)" "Lockin Y (A or V)" "R (A or V)" "Theta (°)" "Mean (A or V)"] -> w1690
              frame "X", Default {
              }
              frame "Y" {
              }
              frame "R" {
              }
              frame "Theta" {
              }
              frame "Mean" {
              }
            }
            n820 = case shown="\"Mean\"" w1685 {
              tunnel: ["Lockin X (A or V)" "Lockin Y (A or V)" "R (A or V)" "Theta (°)" "Mean (A or V)"] -> w1686
              frame "X", Default {
              }
              frame "Y" {
              }
              frame "R" {
              }
              frame "Theta" {
              }
              frame "Mean" {
              }
            }
            n821 = property on="Property Node" class="WFGraph (strict)"(reference=w1689, "YScale.NameLbl.Text"=w1690) -> ()  [unwired: 1 in, 2 out]
            n822 = property on="Property Node" class="WFGraph (strict)"(reference=w1688, "YScale.NameLbl.Text"=w1686) -> ()  [unwired: 1 in, 2 out]
            n823 = call <vilib>:"Add State(s) to Queue__jki_lib_state_machine.vi"("State(s) in (\"\")"=w1695) -> ("States Out"=w1694:string)  [unwired: 14 in]
          }
          frame "UI: Update Sweep Graphs" {
            # "UI: Update Sweep Graphs.\n()"
            n824 = Unbundle By Name(w1712) -> ("getAll.SweepWaveforms.AO"=w1708:waveform(dbl)[], "getAll.SweepWaveforms.AI"=w1711:waveform(dbl)[], "getAll.SweepWaveforms.X"=w1710:waveform(dbl)[], "getAll.SweepWaveforms.Y"=w1709:waveform(dbl)[])
            n825 = Empty Array?(array=w1708) -> (empty?=w1707:bool)
            n826 = Not(x=w1707) -> (.not. x?=w1706:bool)
            n827 = case shown="True" w1706 {
              tunnel: w1711 -> [_ w1720]
              tunnel: w1710 -> [_ w1719]
              tunnel: w1709 -> [_ w1718]
              tunnel: w1708 -> [_ w1717]
              frame False {
              }
              frame True {
                "Sweep X" <- w1719
                "Sweep AO" <- w1717
                "Sweep AI" <- w1720
                "Sweep Y" <- w1718
              }
            }
            n828 = call <vilib>:"Add State(s) to Queue__jki_lib_state_machine.vi"("State(s) in (\"\")"=w1716) -> ("States Out"=w1715:string)  [unwired: 14 in]
          }
          frame "UI: Update Sweep Timer" {
            # "Do not put any code in this frame.\n(It is a separator no-op. You can make a copy of this frame to create a new UI frame)"
            n829 = local read "Sweep Time (s)"() -> (w1724:dbl)
            n830 = local read "Initial Wait (s)"() -> (w1723:dbl)
            n831 = Unbundle By Name(w1722) -> ("DAQ state"=w1721:T33)
            n832 = case shown="\"sweeping\"" w1721 {
              tunnel: [0.0 w1734] -> w1725
              tunnel: w1724 -> [_ w1732]
              tunnel: w1723 -> [_ w1731]
              frame Default {
              }
              frame "sweeping" {
                # "some overhead"
                n833 = call <userlib>:"MGI Milliseconds Since Last Reset.vi"() -> ("ms"=w1738:u32)  [unwired: 6 in, 1 out]
                n834 = Divide(x=w1738, y=u32 1000) -> (x/y=w1736:dbl)
                n835 = Negate(x=w1736) -> (-x=w1735:dbl)
                n836 = Compound Arithmetic op=ADD(2.0 ("value"), w1731, w1732, w1735) -> (w1734:dbl)
              }
            }
            n837 = local write "Sweep Timer (s)"(w1725) -> ()
            n838 = call <vilib>:"Add State(s) to Queue__jki_lib_state_machine.vi"("State(s) in (\"\")"=w1729) -> ("States Out"=w1728:string)  [unwired: 14 in]
          }
          frame "UI: Update Sweep Config" {
            # "UI: Update Sweep Config\n(Called by <DAQ Public Events.getSweepChannels>: User Event)"
            n839 = Unbundle By Name(w1745) -> ("UI Config.Sweep"=w1741:T55)
            n840 = Unbundle By Name(w1741) -> ("sweepTime"=w1743:dbl, "initialWaitTime"=w1744:dbl, "returnToStart"=w1742:bool, "sweepChannels"=w1739:T20)
            n841 = for {
              tunnel: w1739 -> [w1753] mode=indexing
              tunnel: [w1750] -> w1740 mode=indexing
              n842 = Unbundle By Name(w1753) -> ("Channel"=w1752:u16, "Table"=w1751:dbl[])
              n843 = Bundle("Channel"=w1752, "Table"=w1751) -> (w1750:cluster{"Channel":u16, "Table":dbl[]})  [unwired: 1 in]
            }
            n844 = local write "Sweep Time (s)"(w1743) -> ()
            n845 = local write "Initial Wait (s)"(w1744) -> ()
            n846 = local write "Return to Start?"(w1742) -> ()
            n847 = local write "Sweep Channels"(w1739) -> ()
            n848 = local write "Sweep Pattern"(w1740) -> ()
            n849 = call <vilib>:"Add State(s) to Queue__jki_lib_state_machine.vi"("State(s) in (\"\")"=w1749) -> ("States Out"=w1748:string)  [unwired: 14 in]
          }
          frame "UI: Initialize PS Graph" {
            # "Do not put any code in this frame.\n(It is a separator no-op. You can make a copy of this frame to create a new UI frame)"
            n850 = Unbundle By Name(w1759) -> ("UI Config.Plot.visibility.AI"=w1757:bool[])
            n851 = Array Size(array=w1757) -> (size(s)=w1754:i32)
            n852 = Initialize Array(cluster{"f0":dbl, "df":dbl, "magnitude":dbl[]} {"f0"=0.0, "df"=1.0, "magnitude"=[0.001]} ("power spectrum"), w1754) -> (w1755:cluster{"f0":dbl, "df":dbl, "magnitude":dbl[]}[])
            n853 = local write "PS Waveform"(w1755) -> ()
            n854 = call <vilib>:"Add State(s) to Queue__jki_lib_state_machine.vi"("State(s) in (\"\")"=w1762) -> ("States Out"=w1761:string)  [unwired: 14 in]
          }
          frame "UI: Update PS Graph Labels" {
            n855 = local read "export mode"() -> (w1766:u16)
            n856 = local read "PS Display"() -> (w1764:enum16{"AO", "AI", "X", "Y", "R", "Theta"})
            n857 = case shown="0, Default" w1766 {
              tunnel: ["%s power spectrum (dB( ))" ("Y Scale.Name Label.Text") "%s power strectral density (dB( )/Hz)" ("Y Scale.Name Label.Text")] -> w1765
              frame 0, Default {
              }
              frame 1 {
              }
            }
            n858 = Unbundle By Name(w1767) -> ("References.Graphs.PS WFGraph"=w1768:refnum<vi>)
            n859 = Format Into String(format string=w1765, w1764) -> (resulting string=w1763:string)  [unwired: 2 in, 1 out]
            n860 = property on="Property Node" class="WFGraph (strict)"(reference=w1768, "YScale.NameLbl.Text"=w1763) -> ()  [unwired: 1 in, 2 out]
            n861 = call <vilib>:"Add State(s) to Queue__jki_lib_state_machine.vi"("State(s) in (\"\")"=w1772) -> ("States Out"=w1771:string)  [unwired: 14 in]
          }
          frame "UI: Update PS Graph Legend" {
            # "UI: Update PS Graph Legend.\n()"
            n862 = local read "PS Display"() -> (w1781:enum16{"AO", "AI", "X", "Y", "R", "Theta"})
            n863 = Unbundle By Name(w1780) -> ("References.Graphs.PS WFGraph"=w1777:refnum<vi>)
            n864 = case shown="\"X\"..\"Theta\"" w1781 {
              tunnel: w1780 -> [w1788 w1794 w1800]
              tunnel: [w1789 w1792 w1796] -> w1778
              tunnel: [w1786 w1790 w1797] -> w1779
              tunnel: w1775 -> [w1785 w1791 w1799]
              frame "AO" {
                n865 = Unbundle By Name(w1788) -> ("UI Config.DAQ.Configuration"=w1787:T9)
                n866 = call "Get AO StringsAndValues.vi"("error in (no error)"=w1785, "Configuration.DAQ"=w1787) -> ("error out"=w1786:errorcluster, "Strings"=w1789:string[])  [unwired: 7 in, 1 out]
              }
              frame "AI" {
                n867 = Unbundle By Name(w1794) -> ("UI Config.DAQ.Configuration"=w1793:T9)
                n868 = call "Get AI StringsAndValues.vi"("error in (no error)"=w1791, "Configuration.DAQ"=w1793) -> ("error out"=w1790:errorcluster, "Strings"=w1792:string[])  [unwired: 7 in, 1 out]
              }
              frame "X".."Theta" {
                n869 = Unbundle By Name(w1800) -> ("UI Config.DAQ.Configuration"=w1801:T9, "UI Config.Channels.Cfg_REF"=w1802:T2)
                n870 = call "Get AI REF StringsAndValues.vi"("error in (no error)"=w1799, "Channels.REF"=w1802) -> ("error out"=w1798:errorcluster, "Strings"=w1804:string[])  [unwired: 7 in, 1 out]
                n871 = call "Get AI StringsAndValues.vi"("error in (no error)"=w1798, "Configuration.DAQ"=w1801) -> ("error out"=w1797:errorcluster, "Strings"=w1803:string[])  [unwired: 7 in, 1 out]
                n872 = call <vilib>:"Space Constant.vi"() -> ("String"=w1795:string)
                n873 = for {
                  tunnel: w1803 -> [w1807]
                  tunnel: w1804 -> [w1808] mode=indexing
                  tunnel: [w1806] -> w1796 mode=concatenating
                  tunnel: w1795 -> [w1805]
                  n874 = for {
                    tunnel: w1808 -> [w1811]
                    tunnel: w1807 -> [w1810] mode=indexing
                    tunnel: [w1812] -> w1806 mode=indexing
                    tunnel: w1805 -> [w1809]
                    n875 = Concatenate Strings(w1810, w1809, w1811) -> (w1812:string)
                  }
                }
              }
            }
            n876 = call-poly "Set Legend.vi"("error in (no error)"=w1779, "Plot.Plot Name"=w1778, "WFGraph (WDT) in"=w1777) -> ("error out"=w1776:errorcluster)  [unwired: 8 in]
            n877 = call <vilib>:"Add State(s) to Queue__jki_lib_state_machine.vi"("State(s) in (\"\")"=w1784) -> ("States Out"=w1783:string)  [unwired: 14 in]
          }
          frame "UI: Update Channel Ring" {
            # "UI: Update Channel Ring.\n()"
            n878 = Unbundle By Name(w1820) -> ("getAll.Results.Results (Dictionary)"=w1816:cluster{"key":string, "value":dbl[]}[])
            n879 = local read "channel-reference"() -> (w1815:u16)
            n880 = call "Dictionary to Plot Names.vi"("error in (no error)"=w1818, "Results (Dictionary)"=w1816) -> ("error out"=w1819:errorcluster, "Plot Names"=w1817:string[])  [unwired: 7 in, 1 out]
            n881 = property on="channel-reference" class="Ring (strict)"(error in=w1819, "Strings []"=w1817, "Value"=w1815) -> (error out=w1814:errorcluster)  [unwired: 1 in, 1 out]
            n882 = case shown="No Error" w1814 {
              selector: w1814 -> [w1824 _]
              tunnel: [w1824 _] -> w1813
              frame No Error {
              }
              frame Error {
                n883 = local write "channel-reference"(0) -> ()
              }
            }
            n884 = call <vilib>:"Add State(s) to Queue__jki_lib_state_machine.vi"("State(s) in (\"\")"=w1823) -> ("States Out"=w1822:string)  [unwired: 14 in]
          }
          frame "UI: Update AI REF Channel Ring" {
            # "update AI Ref Channel ring"
            # "Do not put any code in this frame.\n(It is a separator no-op. You can make a copy of this frame to create a new UI frame)"
            n885 = Unbundle By Name(w1829) -> ("UI Config.Channels.Cfg_REF"=w1828:T2)
            n886 = call "Get REF StringsAndValues.vi"("error in (no error)"=w1827, "Channels.REF"=w1828) -> ("error out"=w1831:errorcluster, "REF Strings and Values"=w1830:cluster{string, i32}[])  [unwired: 8 in]
            n887 = property on="reference channel" class="Ring (strict)"(error in=w1831, "StringsAndValues[]"=w1830) -> (error out=w1826:errorcluster)  [unwired: 1 in, 1 out]
            n888 = call <vilib>:"Add State(s) to Queue__jki_lib_state_machine.vi"("State(s) in (\"\")"=w1834) -> ("States Out"=w1833:string)  [unwired: 14 in]
          }
          frame "UI: Sync AI Ref Array" {
            n889 = Scan From String(input string=w1841, default 1=0 ("index")) -> (output 1=w1838:i32)  [unwired: 3 in, 3 out]
            n890 = local read "AI Channels"() -> (w1837:T4)
            n891 = Index Array(array=w1837, index=w1838) -> (element=w1843:T5)
            n892 = Array Size(array=w1837) -> (size(s)=w1836:i32)
            n893 = Unbundle By Name(w1843) -> ("reference index"=w1842:i32)
            n894 = for {
              N: w1836 -> [_]
              tunnel: w1842 -> [w1853]
              shift-right: [w1850] -> w1839
              shift-left: w1837 -> [w1852]
              i -> [w1851]
              n895 = in-place {
                in-place-border: w1853 -> [w1856]
                n896 = in-place-array #1(w1852, w1851) -> (w1855:T5)
                n897 = Bundle By Name(cluster=w1855, "reference index"=w1856) -> (w1854:T5)
                n898 = in-place-array #1(w1854) -> (w1850:T4)  [unwired: 1 out]
              }
            }
            n899 = control-ref of="References"() -> (w1835:refnum<vi>)
            n900 = Build Array(w1842) -> (w1844:i32[])
            n901 = property on="Property Node" class="Arr (strict)"(reference=w1835, "Index Values"=w1844) -> ()  [unwired: 1 in, 2 out]
            n902 = local write "AI Channels"(w1839) -> ()
            n903 = call <vilib>:"Add State(s) to Queue__jki_lib_state_machine.vi"("State(s) in (\"\")"=w1849) -> ("States Out"=w1848:string)  [unwired: 14 in]
          }
          frame "UI: Remove Unused References" {
            # "update Ch.AI after removing\nunused Ch.REF"
            # "Do not put any code in this frame.\n(It is a separator no-op. You can make a copy of this frame to create a new UI frame)"
            n904 = Unbundle By Name(w1862) -> ("UI Config.Channels.Cfg_AI"=w1861:T4, "UI Config.Channels.Cfg_REF"=w1860:T2)
            n905 = call "Remove Unused References.vi"("error in (no error)"=w1858, "Channels.REF"=w1860, "Channels.AI"=w1861) -> ("error out"=w1859:errorcluster, "Channels.AI out"=w1857:T4)  [unwired: 7 in]
            n906 = local write "AI Channels"(w1857) -> ()
            n907 = call <vilib>:"Add State(s) to Queue__jki_lib_state_machine.vi"("State(s) in (\"\")"=w1865) -> ("States Out"=w1864:string)  [unwired: 14 in]
          }
          frame "UI: Update AI REF Channels" {
            # "UI: Update AI REF Channels\n(enable/disable demodulation channels)"
            n908 = Unbundle By Name(w1868) -> ("UI Config.Channels.Cfg_AI"=w1872:T4, "UI Config.Channels.Cfg_REF"=w1866:T2)
            n909 = case shown="\"All 1\"" w1867 {
              tunnel: [w1877 i32[] [0] ("References")] -> w1871
              tunnel: w1866 -> [w1878 _]
              frame "All 1" {
                n910 = for {
                  tunnel: w1878 -> [w1881] mode=indexing
                  tunnel: [w1880] -> w1877 mode=indexing if=w1879
                  n911 = Unbundle By Name(w1881) -> ("Channel"=w1880:i32, "Enable?"=w1879:bool)
                }
              }
              frame "Disable", Default {
              }
            }
            n912 = for {
              tunnel: w1872 -> [w1885] mode=indexing
              tunnel: [w1884] -> w1869 mode=indexing
              tunnel: w1871 -> [w1883]
              n913 = Bundle By Name(cluster=w1885, "References"=w1883) -> (w1884:T5)
            }
            n914 = Bundle By Name(cluster=w1868, "UI Config.Channels.Cfg_AI"=w1869) -> (w1870:T65)
            n915 = local write "AI Channels"(w1869) -> ()
            n916 = call <vilib>:"Add State(s) to Queue__jki_lib_state_machine.vi"("State(s) in (\"\")"=w1876) -> ("States Out"=w1875:string)  [unwired: 14 in]
          }
          frame "UI: Update Sampling Status" {
            # "Do not put any code in this frame.\n(It is a separator no-op. You can make a copy of this frame to create a new UI frame)"
            n917 = Unbundle By Name(w1890) -> ("getAll.Waveforms.AI"=w1889:waveform(dbl)[])
            n918 = call <userlib>:"MGI Milliseconds Since Last Call.vi"() -> ("ms"=w1897:u32)  [unwired: 6 in, 1 out]
            "Wfm Refresh Time (ms)" <- w1897
            n919 = Index Array(array=w1889) -> (element=w1903:waveform(dbl))  [unwired: 1 in]
            n920 = call-poly <vilib>:"Waveform Duration.vi"("error in (no error)"=w1887, "waveform in"=w1903) -> ("error out"=w1888:errorcluster, "duration"=w1902:dbl)  [unwired: 7 in, 1 out]
            n921 = Multiply(x=w1902, y=1000.0) -> (x*y=w1901:dbl)
            n922 = Multiply(x=w1901, y=2.0) -> (x*y=w1900:dbl)
            n923 = Less?(x=w1897, y=w1900) -> (x < y?=w1899:bool)
            n924 = Select(t=u32 6618880, s=w1899, f=u32 16711680) -> (s? t:f=→"Sampling Status":u32)
            n925 = Select(t="Good", s=w1899, f="#s/Fs: too small!") -> (s? t:f=→"Sampling Status":string)
            n926 = call <vilib>:"Add State(s) to Queue__jki_lib_state_machine.vi"("State(s) in (\"\")"=w1906) -> ("States Out"=w1905:string)  [unwired: 14 in]
          }
          frame "---------- Macro ----------" {
            # "Do not put any code in this frame.\n(It is a separator no-op. You can make a copy of this frame to create a new Macro frame)"
            n927 = call <vilib>:"Add State(s) to Queue__jki_lib_state_machine.vi"("State(s) in (\"\")"=w1911) -> ("States Out"=w1910:string)  [unwired: 14 in]
          }
          frame "Macro: Initialize" {
            # "Initialization Macro\n(This is called once, when the VI starts)"
            n928 = call <vilib>:"Add State(s) to Queue__jki_lib_state_machine.vi"("State(s) in Front (\"\")"="Data: Initialize\nInitialize Core Data\nEvents: Register", "State(s) in (\"\")"="") -> ("States Out"=w1912:string)  [unwired: 13 in]
            n929 = call <vilib>:"Add State(s) to Queue__jki_lib_state_machine.vi"("State(s) in Front (\"\")"=w1912, "State(s) in (\"\")"="Process: Sync", "State(s) at Back (\"\")"="UI: Initialize\nMacro: Initialize UI Before Open\nUI: Front Panel State >> Open\nMacro: Initialize UI After Open\nData: Wait >> 500\nMacro: Initialize III") -> ("States Out"=w1916:string)  [unwired: 12 in]
            n930 = call <vilib>:"Add State(s) to Queue__jki_lib_state_machine.vi"("State(s) in Front (\"\")"=w1916, "State(s) in (\"\")"=w1922) -> ("States Out"=w1921:string)  [unwired: 13 in]
          }
          frame "Macro: Post Error Handling" {
            # "Clear Last Error?"
            # "Do not put any code in this frame.\n(It is a separator no-op. You can make a copy of this frame to create a new Macro frame)"
            n931 = Unbundle By Name(w1924) -> ("Core.Last Error.remaining states"=w1926:string, "Core.Shutdown?"=w1927:bool)
            n932 = Unbundle By Name(w1924) -> ("Core.Last Error.error"=w1930:errorcluster)
            n933 = case shown="False" FALSE {
              tunnel: w1930 -> [w1938 _]
              tunnel: [w1938 _] -> w1929
              frame False {
              }
              frame True {
              }
            }
            n934 = case shown="True" w1927 {
              tunnel: w1926 -> [w1935 w1937]
              tunnel: [w1935 w1936] -> w1923
              frame False {
                # "These are the remaining states (at the moment the error occured). States can be altered according to business logic."
                # "NOT SHUTTING DOWN"
              }
              frame True {
                # "Developer can decide to alter the states but should be aware that during the shutdown process, there are certain states that must be run for the SMO to properly shut itself (and this process) down. As such, one can add states to perform additional clean-ups, but should append the remaining state to be executed."
                # "SHUTTING DOWN"
                n935 = call <vilib>:"Add State(s) to Queue__jki_lib_state_machine.vi"("State(s) in (\"\")"=w1937) -> ("States Out"=w1936:string)  [unwired: 14 in]
              }
            }
            n936 = Bundle By Name(cluster=w1924, "Core.Last Error.error"=w1929) -> (w1925:T65)
            n937 = call <vilib>:"Add State(s) to Queue__jki_lib_state_machine.vi"("State(s) in Front (\"\")"=w1923, "State(s) in (\"\")"=w1934) -> ("States Out"=w1933:string)  [unwired: 13 in]
          }
          frame "Macro: Initialize UI Before Open" {
            # "Initialize UI\n(This is called after UI: Initialize and before UI: Front Panel State >> Open)"
            n938 = local write "Show DAQ UI"(FALSE ("Show UI")) -> ()
            n939 = call <vilib>:"Add State(s) to Queue__jki_lib_state_machine.vi"("State(s) in Front (\"\")"="UI: Cursor Set >> Busy\nUI: Defer Panel Updates >> TRUE\n\nData: Initialize Control References\nData: Initialize Graph References\n\nUI: Reinit To Default\nUI: Disable Buttons\n\nConfiguration: Initialize\nConfiguration: Read File\nUI: Cluster to UI\nUI: Cluster to UI 2\nUI: Init Graph Data\nUI: Init Graph Legends\nUI: Update PS Graph Legend\nUI: Update Waveform Graph Labels\n\nUI: Defer Panel Updates >> FALSE" ("State(s) in Front (\"\")"), "State(s) in (\"\")"=w1945) -> ("States Out"=w1944:string)  [unwired: 13 in]
          }
          frame "Macro: Initialize UI After Open" {
            # "Initialize UI\n(This is called after UI: Initialize and before UI: Front Panel State >> Open)"
            n940 = Format Into String(format string="UI: Defer Panel Updates >> TRUE\nUI: Set Left Tab >> %s\nUI: Set Right Tab >> %s\nAction: IDN\nUI: Defer Panel Updates >> FALSE\nUI: Cursor Set >> Idle" ("State(s) in Front (\"\")"), T1."Status" ("Left Tab"), T25."AO/AI Graphs" ("Right Tab")) -> (resulting string=w1948:string)  [unwired: 2 in, 1 out]
            n941 = call <vilib>:"Add State(s) to Queue__jki_lib_state_machine.vi"("State(s) in Front (\"\")"=w1948, "State(s) in (\"\")"=w1954) -> ("States Out"=w1953:string)  [unwired: 13 in]
          }
          frame "Macro: Initialize III" {
            # "Initialize UI\n(This is called after UI: Initialize and before UI: Front Panel State >> Open)"
            n942 = Format Into String(format string="UI: Cursor Set >> Busy\n\nMacro: Initialize DAQ\nIdle\nMacro: Initialize Waveform Graphs\nMacro: Initialize Lockin Graphs\n\nIdle\nUI: Defer Panel Updates >> TRUE\nUI: Enable Buttons\nUI: Init Scroll Bars\nUI: Set Left Tab >> %s\nUI: Set Right Tab >> %s\nUI: Defer Panel Updates >> FALSE\n\nUI: Cursor Set >> Idle" ("State(s) in Front (\"\")"), T1."AO/AI/REF" ("Left Tab"), T25."AO/AI Graphs" ("Right Tab")) -> (resulting string=w1957:string)  [unwired: 2 in, 1 out]
            n943 = call <vilib>:"Add State(s) to Queue__jki_lib_state_machine.vi"("State(s) in Front (\"\")"=w1957, "State(s) in (\"\")"=w1963) -> ("States Out"=w1962:string)  [unwired: 13 in]
          }
          frame "Macro: Initialize DAQ" {
            # "change order\n#180"
            # "Action: State >> reset\n//Action: Offset"
            n944 = call <vilib>:"Delimited String to 1D String Array.vi"("delimiter"="\n", "delimited string"="Action: AI Channels\nAction: DAQ Config\nAction: Input Gain\nAction: Output Gain\nAction: Offset\nAction: AO Channels\nAction: REF Channels\nAction: Sampling\nAction: Sampling Fs Mode\nAction: Sampling Fs Multiplier\nAction: Sampling Fs Output\nAction: Sampling Refresh Rate\nAction: Sampling Decimation Pre DSP\nAction: Sampling Decimation Post DSP\nAction: AI Simulate Mode\nAction: Sweep\nAction: Limit Amplitude\nAction: Limit DC\nAction: Link Frequencies\nAction: Duty Cycle\nAction: PreFilter\nAction: Offset Mode >> Remove\nAction: Log Configuration" ("State(s) in Front (\"\")")) -> ("string array"=w1964:string[])  [unwired: 9 in]
            n945 = Array Size(array=w1964) -> (size(s)=w1971:i32)
            n946 = Initialize Array("Action: Command\nData: Wait >> 25\n//Idle", w1971) -> (w1970:string[])
            n947 = Interleave 1D Arrays(w1964, w1970) -> (w1965:string[])
            n948 = call <vilib>:"1D String Array to Delimited String.vi"("delimiter"="\n", "string array"=w1965) -> ("delimited string"=w1969:string)  [unwired: 9 in]
            n949 = call <vilib>:"Add State(s) to Queue__jki_lib_state_machine.vi"("State(s) in Front (\"\")"=w1969, "State(s) in (\"\")"=w1977) -> ("States Out"=w1976:string)  [unwired: 13 in]
          }
          frame "Macro: Initialize Waveform Graphs" {
            n950 = call <vilib>:"Add State(s) to Queue__jki_lib_state_machine.vi"("State(s) in Front (\"\")"="UI: Defer Panel Updates >> TRUE\n\nUI: Update Waveform Graphs\nUI: Update Sweep Graphs\n\nUI: Update AI REF Channel Ring\n\nUI: Update AI Waveform Graphs Legends\nUI: Update AI Waveform Graphs Colors\nUI: Update AO Waveform Graphs Legends\nUI: Update AO Waveform Graphs Colors\nUI: Update REF Waveform Graphs Legends\nUI: Update REF Waveform Graphs Colors\n\nUI: Set Plot Visibility //from UI cluster\nUI: Sync AI Plot Visibility\nUI: Sync AO Plot Visibility\nUI: Show Hide AO Waveform Graphs\nUI: Initialize PS Graph\nUI: Update PS Graph Labels\n\nUI: Defer Panel Updates >> FALSE" ("State(s) in Front (\"\")"), "State(s) in (\"\")"=w1983) -> ("States Out"=w1982:string)  [unwired: 13 in]
          }
          frame "Macro: Initialize Lockin Graphs" {
            n951 = call <vilib>:"Add State(s) to Queue__jki_lib_state_machine.vi"("State(s) in Front (\"\")"="UI: Defer Panel Updates >> TRUE\n\nUI: Update Lockin Graphs\n\nUI: Update Channel Ring\nUI: Update Lockin Graph Labels\nUI: Update Lockin Graphs Legends\nUI: Update Lockin Graphs Colors\n\nUI: Sync Lockin Plot Visibility\n\nUI: Defer Panel Updates >> FALSE" ("State(s) in Front (\"\")"), "State(s) in (\"\")"=w1989) -> ("States Out"=w1988:string)  [unwired: 13 in]
          }
          frame "Macro: Update Waveform Graphs" {
            n952 = local read "Right Tab"() -> (w1995:T25)
            n953 = case shown="\"PS\"" w1995 {
              tunnel: ["UI: Update Waveform Graphs" ("State(s) in Front (\"\")") "Action: Power Spectrum" ("State(s) in Front (\"\")") "" ("State(s) in Front (\"\")")] -> w1993
              frame "AO/AI Graphs" {
              }
              frame "PS" {
              }
              frame Default {
              }
            }
            n954 = call <vilib>:"Add State(s) to Queue__jki_lib_state_machine.vi"("State(s) in Front (\"\")"="UI: Update Sampling Status\nData: Waveform Legends" ("State(s) in Front (\"\")"), "State(s) at Back (\"\")"=w1993) -> ("States Out"=w1992:string)  [unwired: 13 in]
            n955 = call <vilib>:"Add State(s) to Queue__jki_lib_state_machine.vi"("State(s) in Front (\"\")"=w1992, "State(s) in (\"\")"=w1998) -> ("States Out"=w1997:string)  [unwired: 13 in]
          }
          frame "Macro: Update Lockin Graphs" {
            n956 = Unbundle By Name(w2004) -> ("getAll.Results.Results (Dictionary)"=w2012:cluster{"key":string, "value":dbl[]}[])
            n957 = call "Dictionary to Plot Names.vi"("error in (no error)"=w2010, "Results (Dictionary)"=w2012) -> ("error out"=w2011:errorcluster, "Plot Names"=w2006:string[])  [unwired: 7 in, 1 out]
            n958 = call "Is Value Changed.vim"("value"=w2006) -> ("changed or first call?"=w2005:bool)
            n959 = Select(t="UI: Defer Panel Updates >> TRUE\nUI: Update Channel Ring\nUI: Update Lockin Graphs Legends\nUI: Update Lockin Graphs Colors\nUI: Defer Panel Updates >> FALSE" ("State(s) in Front (\"\")"), s=w2005, f="") -> (s? t:f=w2002:string)
            n960 = call <vilib>:"Add State(s) to Queue__jki_lib_state_machine.vi"("State(s) in Front (\"\")"="UI: Update Lockin Graphs" ("State(s) in Front (\"\")"), "State(s) at Back (\"\")"=w2002) -> ("States Out"=w2007:string)  [unwired: 13 in]
            n961 = call <vilib>:"Add State(s) to Queue__jki_lib_state_machine.vi"("State(s) in Front (\"\")"=w2007, "State(s) in (\"\")"=w2015) -> ("States Out"=w2014:string)  [unwired: 13 in]
          }
          frame "Macro: Save Configuration" {
            n962 = call <vilib>:"Add State(s) to Queue__jki_lib_state_machine.vi"("State(s) in Front (\"\")"="UI: Defer Panel Updates >> TRUE\nUI: Get Plot Visibility\nUI: UI to Cluster\nUI: UI to Cluster 2\nConfiguration: Write File\nUI: Defer Panel Updates >> FALSE", "State(s) in (\"\")"=w2021) -> ("States Out"=w2020:string)  [unwired: 13 in]
          }
          frame "Macro: Exit" {
            # "Exit Macro\n(This is called once, when the VI exits)"
            n963 = Unbundle By Name(w2024) -> ("Core.Close Panel on Exit?"=w2035:bool)
            n964 = Bundle By Name(cluster=w2024, "Core.Shutdown?"=TRUE) -> (w2025:T65)
            n965 = Select(t="UI: Front Panel State >> Open", s=w2035, f="") -> (s? t:f=w2022:string)
            n966 = call <vilib>:"Add State(s) to Queue__jki_lib_state_machine.vi"("State(s) in Front (\"\")"="Data: Cleanup\nEvents: Unregister\nProcess: Self Terminate", "State(s) in (\"\")"="Process: Sync", "State(s) at Back (\"\")"="Exit") -> ("States Out"=w2023:string)  [unwired: 12 in]
            n967 = call <vilib>:"Add State(s) to Queue__jki_lib_state_machine.vi"("State(s) in Front (\"\")"="Macro: Save Configuration", "State(s) in (\"\")"=w2022, "State(s) at Back (\"\")"=w2023) -> ("States Out"=w2032:string)  [unwired: 12 in]
            n968 = call <vilib>:"Add State(s) to Queue__jki_lib_state_machine.vi"("State(s) in Front (\"\")"=w2032, "State(s) in (\"\")"=w2038) -> ("States Out"=w2037:string)  [unwired: 13 in]
          }
          frame "---------- Process ----------" {
            # "Template Separator\n(You can make a copy of, or modify, this frame)"
            n969 = call <vilib>:"Add State(s) to Queue__jki_lib_state_machine.vi"("State(s) in (\"\")"=w2043) -> ("States Out"=w2042:string)  [unwired: 14 in]
          }
          frame "Process: Sync" {
            n970 = Unbundle By Name(w2051) -> ("SMO"=w2047:refnum<class "Instrument UI.Lockin.lvclass">)
            n971 = call <vilib>:"WaitOnProcessSync.vi"("error in (no error)"=w2046, "SMO"=w2047) -> ("error out"=w2045:errorcluster, "Don't run?"=w2050:bool)  [unwired: 7 in, 1 out]
            n972 = Select(t="Data: Cleanup\nEvents: Unregister\nExit", s=w2050, f="") -> (s? t:f=w2044:string)
            n973 = call <vilib>:"Add State(s) to Queue__jki_lib_state_machine.vi"("State(s) in Front (\"\")"=w2044, "State(s) in (\"\")"=w2054) -> ("States Out"=w2053:string)  [unwired: 13 in]
          }
          frame "Process: Self Terminate" {
            n974 = Unbundle By Name(w2056) -> ("SMO"=w2055:refnum<class "Instrument UI.Lockin.lvclass">)
            n975 = call <vilib>:"SelfTerminate.vi"("error in (no error)"=w2058, "SMO in"=w2055) -> ("error out"=w2057:errorcluster)  [unwired: 8 in, 1 out]
            n976 = call <vilib>:"Add State(s) to Queue__jki_lib_state_machine.vi"("State(s) in (\"\")"=w2061) -> ("States Out"=w2060:string)  [unwired: 14 in]
          }
          frame "---------- Events ----------" {
            # "Template Separator\n(You can make a copy of, or modify, this frame)"
            n977 = call <vilib>:"Add State(s) to Queue__jki_lib_state_machine.vi"("State(s) in (\"\")"=w2066) -> ("States Out"=w2065:string)  [unwired: 14 in]
          }
          frame "Events: Register" {
            # "Base Class Protected Events"
            n978 = Unbundle By Name(w2083) -> ("SMO"=w2079:refnum<class "Instrument UI.Lockin.lvclass">, "Lockin"=w2073:refnum<class "Instrument.Lockin.lvclass">)
            n979 = call <vilib>:"GetProtectedEvents.vi"("SMO"=w2079) -> ("error out"=w2080:errorcluster, "SMO Protected Events"=w2072:T70, "SMO out"=w2071:refnum<class "Instrument UI.Lockin.lvclass">)  [unwired: 8 in]
            n980 = call <userlib>:"Instrument.GetPublicEvents.vi"("Instrument"=w2073) -> ("error out"=w2078:errorcluster, "Instrument Public Events"=w2074:T71, "Instrument out"=w2075:refnum<class "Instrument.Lockin.lvclass">)  [unwired: 8 in]
            n981 = call <vilib>:"SMO.UI.GetPublicEvents.vi"("SMO.UI"=w2071) -> ("SMO.UI Public Events"=w2070:T72)  [unwired: 8 in, 2 out]
            n982 = call "Lockin.getDAQPublicEvents.vi"("Instrument.Lockin in"=w2075) -> ("error out"=w2068:errorcluster, "DAQ SMO Public Events"=w2069:T73, "DAQ Public Events"=w2067:T74)  [unwired: 7 in, 1 out]
            n983 = register-events(w2072, w2070, w2074, w2067, w2069) -> (reference out=w2082:refnum<event-registration>, error out=w2077:errorcluster)  [unwired: 2 in]
            n984 = Merge Errors(w2077, w2068, w2078, w2080, w2076) -> (w2081:errorcluster)
            n985 = call <vilib>:"Add State(s) to Queue__jki_lib_state_machine.vi"("State(s) in (\"\")"=w2085) -> ("States Out"=w2084:string)  [unwired: 14 in]
          }
          frame "Events: Unregister" {
            n986 = Unregister For Events(event registration refnum=w2088, error in=w2087) -> (error out=w2086:errorcluster)
            n987 = call <vilib>:"Add State(s) to Queue__jki_lib_state_machine.vi"("State(s) in (\"\")"=w2091) -> ("States Out"=w2090:string)  [unwired: 14 in]
          }
          frame "---------- Action ----------" {
            n988 = Unbundle By Name(w2092) -> ("SMO"=w2094:refnum<class "Instrument UI.Lockin.lvclass">)
            n989 = Bundle By Name(cluster=w2092, "SMO"=w2094) -> (w2093:T65)
            n990 = call <vilib>:"Add State(s) to Queue__jki_lib_state_machine.vi"("State(s) in (\"\")"=w2098) -> ("States Out"=w2097:string)  [unwired: 14 in]
          }
          frame "Action: ><><>Unhandled Controls<><><" {
            n991 = call <vilib>:"Add State(s) to Queue__jki_lib_state_machine.vi"("State(s) in (\"\")"=w2103) -> ("States Out"=w2102:string)  [unwired: 14 in]
          }
          frame "Action: Notify UI Closed" {
            # "Notify that the UI has been closed"
            n992 = Unbundle By Name(w2106) -> ("SMO"=w2107:refnum<class "Instrument UI.Lockin.lvclass">)
            n993 = call <vilib>:"Hide.vi"("error in (no error)"=w2105, "SMO.UI"=w2107) -> ("error out"=w2104:errorcluster)  [unwired: 8 in, 1 out]
            n994 = call <vilib>:"Add State(s) to Queue__jki_lib_state_machine.vi"("State(s) in (\"\")"=w2110) -> ("States Out"=w2109:string)  [unwired: 14 in]
          }
          frame "Action: Command" {
            n995 = Unbundle By Name(w2118) -> ("Lockin"=w2116:refnum<class "Instrument.Lockin.lvclass">, "Message.Command"=w2115:variant, "Message.Data"=w2114:variant)
            n996 = call "Lockin.Local Client.vim"("error in (no error)"=w2113, "Data"=w2114, "Command"=w2115, "Instrument.Lockin in"=w2116) -> ("error out"=w2112:errorcluster, "Instrument.Lockin out"=w2111:refnum<class "Instrument.Lockin.lvclass">)  [unwired: 6 in]
            n997 = Bundle By Name(cluster=w2118, "Lockin"=w2111) -> (w2119:T65)
            n998 = call <vilib>:"Add State(s) to Queue__jki_lib_state_machine.vi"("State(s) in Front (\"\")"="" ("State(s) in Front (\"\")"), "State(s) in (\"\")"=w2122) -> ("States Out"=w2121:string)  [unwired: 13 in]
          }
          frame "Action: IDN" {
            n999 = Unbundle By Name(w2130) -> ("Lockin"=w2128:refnum<class "Instrument.Lockin.lvclass">)
            n1000 = call <userlib>:"IDN.vi"("error in (no error)"=w2127, "Instrument in"=w2128) -> ("error out"=w2126:errorcluster, "IDN"=w2124:T75, "Instrument in"=w2125:refnum<class "Instrument.Lockin.lvclass">)  [unwired: 7 in]
            n1001 = Unbundle By Name(w2124) -> ("serial"=→"System Serial Number":string)
            n1002 = Bundle By Name(cluster=w2130, "Lockin"=w2125) -> (w2131:T65)
            n1003 = call <vilib>:"Add State(s) to Queue__jki_lib_state_machine.vi"("State(s) in Front (\"\")"="" ("State(s) in Front (\"\")"), "State(s) in (\"\")"=w2134) -> ("States Out"=w2133:string)  [unwired: 13 in]
          }
          frame "Action: State" {
            n1004 = Scan From String(input string=w2139, default 1=State--enum."start" ("State")) -> (output 1=w2136:T29)  [unwired: 3 in, 3 out]
            n1005 = Bundle By Name(cluster=T37 {"State"=enum."start"} ("setState"), "State"=w2136) -> (w2135:T37)
            n1006 = Bundle By Name(cluster=w2141, "Message.Command"=Lockin.Commands--Enum."setState" ("Locking.Commands"), "Message.Data"=w2135) -> (w2142:T65)
            n1007 = call <vilib>:"Add State(s) to Queue__jki_lib_state_machine.vi"("State(s) in (\"\")"=w2146) -> ("States Out"=w2145:string)  [unwired: 14 in]
          }
          frame "Action: show DAQ UI" {
            n1008 = Scan From String(input string=w2150, default 1=T40 FALSE ("showDAQUI")) -> (output 1=w2147:T40)  [unwired: 3 in, 3 out]
            n1009 = Bundle By Name(cluster=w2151, "Message.Command"=Lockin.Commands.Local--Enum."showUI" ("Locking.Commands.Local"), "Message.Data"=w2147) -> (w2152:T65)
            n1010 = call <vilib>:"Add State(s) to Queue__jki_lib_state_machine.vi"("State(s) in (\"\")"=w2156) -> ("States Out"=w2155:string)  [unwired: 14 in]
          }
          frame "Action: Logging" {
            n1011 = Scan From String(input string=w2168, default 1=FALSE ("showDAQUI")) -> (output 1=w2161:bool)  [unwired: 3 in, 3 out]
            n1012 = Select(t=Lockin.Commands--Enum."startLogging" ("Locking.Commands"), s=w2161, f=Lockin.Commands--Enum."stopLogging" ("Locking.Commands")) -> (s? t:f=w2162:T38)
            n1013 = Bundle By Name(cluster=T41 {"interval"=1} ("setLogging"), "interval"=u32 1000 ("LogMode")) -> (w2165:T41)
            n1014 = To Variant(anything=w2165) -> (Variant=w2159:variant)
            n1015 = Select(t=w2159, s=w2161, f=variant) -> (s? t:f=w2158:variant)
            n1016 = Bundle By Name(cluster=w2169, "Message.Command"=w2162, "Message.Data"=w2158) -> (w2170:T65)
            n1017 = call <vilib>:"Add State(s) to Queue__jki_lib_state_machine.vi"("State(s) in (\"\")"=w2174) -> ("States Out"=w2173:string)  [unwired: 14 in]
          }
          frame "Action: Log Configuration" {
            n1018 = Bundle By Name(cluster=w2177, "Message.Command"=Lockin.Commands--Enum."logConfiguration" ("Locking.Commands"), "Message.Data"=variant) -> (w2178:T65)
            n1019 = call <vilib>:"Add State(s) to Queue__jki_lib_state_machine.vi"("State(s) in (\"\")"=w2182) -> ("States Out"=w2181:string)  [unwired: 14 in]
          }
          frame "Action: Auto DAQ" {
            n1020 = Bundle By Name(cluster=w2184, "Message.Command"=Lockin.Commands.Local--Enum."autoConfigureDAQ" ("Locking.Commands.Local")) -> (w2185:T65)
            n1021 = call <vilib>:"Add State(s) to Queue__jki_lib_state_machine.vi"("State(s) in (\"\")"=w2189) -> ("States Out"=w2188:string)  [unwired: 14 in]
          }
          frame "Action: DAQ Config" {
            n1022 = Unbundle By Name(w2192) -> ("UI Config.DAQ.Configuration"=w2190:T9)
            n1023 = Bundle By Name(cluster=w2192, "Message.Command"=Lockin.Commands--Enum."setDAQ" ("Locking.Commands"), "Message.Data"=w2190) -> (w2193:T65)
            n1024 = call <vilib>:"Add State(s) to Queue__jki_lib_state_machine.vi"("State(s) in (\"\")"=w2197) -> ("States Out"=w2196:string)  [unwired: 14 in]
          }
          frame "Action: AI Channels" {
            n1025 = Unbundle By Name(w2200) -> ("UI Config.Channels.Cfg_AI"=w2199:T4)
            n1026 = Bundle By Name(cluster=w2200, "Message.Command"=Lockin.Commands.Local--Enum."setAI" ("Locking.Commands.Local"), "Message.Data"=w2199) -> (w2201:T65)
            n1027 = call <vilib>:"Add State(s) to Queue__jki_lib_state_machine.vi"("State(s) in (\"\")"=w2205) -> ("States Out"=w2204:string)  [unwired: 14 in]
          }
          frame "Action: AO Channels" {
            n1028 = Unbundle By Name(w2208) -> ("UI Config.Channels.Cfg_AO"=w2206:T6)
            n1029 = Bundle By Name(cluster=w2208, "Message.Command"=Lockin.Commands--Enum."setAO" ("Locking.Commands"), "Message.Data"=w2206) -> (w2209:T65)
            n1030 = call <vilib>:"Add State(s) to Queue__jki_lib_state_machine.vi"("State(s) in (\"\")"=w2213) -> ("States Out"=w2212:string)  [unwired: 14 in]
          }
          frame "Action: AO Zero Amplitude" {
            n1031 = Unbundle By Name(w2214) -> ("UI Config.Channels.Cfg_AO"=w2217:T6)
            n1032 = for {
              tunnel: w2217 -> [w2226] mode=indexing
              tunnel: [w2224] -> w2216 mode=indexing
              n1033 = Bundle By Name(cluster=w2226, "Amplitude"=0.0 ("element")) -> (w2224:T7)
            }
            n1034 = Bundle By Name(cluster=w2214, "Message.Command"=Lockin.Commands--Enum."setAO" ("Enum"), "Message.Data"=w2216) -> (w2215:T65)
            n1035 = call <vilib>:"Add State(s) to Queue__jki_lib_state_machine.vi"("State(s) in Front (\"\")"="", "State(s) in (\"\")"=w2223) -> ("States Out"=w2222:string)  [unwired: 13 in]
          }
          frame "Action: REF Channels" {
            n1036 = Unbundle By Name(w2231) -> ("UI Config.Channels.Cfg_REF"=w2229:T2, "UI Config.DAQ.cfg.Sampling.Sampling"=w2227:T49)
            n1037 = call "Calculate Output Sampling.vi"("sampling info"=w2227, "Cfg_REF"=w2229) -> ("Cfg_REF out"=w2228:T2)  [unwired: 8 in, 1 out]
            n1038 = Bundle By Name(cluster=w2231, "Message.Command"=Lockin.Commands--Enum."setREF" ("Locking.Commands"), "Message.Data"=w2228) -> (w2232:T65)
            n1039 = call <vilib>:"Add State(s) to Queue__jki_lib_state_machine.vi"("State(s) in (\"\")"=w2236) -> ("States Out"=w2235:string)  [unwired: 14 in]
          }
          frame "Action: Sweep" {
            n1040 = Unbundle By Name(w2239) -> ("UI Config.Sweep"=w2237:T55)
            n1041 = Bundle By Name(cluster=w2239, "Message.Command"=Lockin.Commands--Enum."setSweep" ("Locking.Commands"), "Message.Data"=w2237) -> (w2240:T65)
            n1042 = call <vilib>:"Add State(s) to Queue__jki_lib_state_machine.vi"("State(s) in (\"\")"=w2244) -> ("States Out"=w2243:string)  [unwired: 14 in]
          }
          frame "Action: Sampling" {
            w2249 = Lockin.Commands--Enum."setSampling"  # Lockin.Commands
            n1043 = Unbundle By Name(w2250) -> ("UI Config.DAQ.cfg.Sampling.Sampling"=w2247:T49)
            n1044 = Bundle By Name(cluster=w2247, "Fs"="Fs (S/s) (buffer)", "#s"="#s (S) (buffer)") -> (w2246:T49)
            n1045 = Bundle By Name(cluster=w2250, "Message.Command"=w2249, "Message.Data"=w2246) -> (w2251:T65)
            n1046 = call <vilib>:"Add State(s) to Queue__jki_lib_state_machine.vi"("State(s) in (\"\")"=w2255) -> ("States Out"=w2254:string)  [unwired: 14 in]
          }
          frame "Action: Sampling Mode" {
            n1047 = Unbundle By Name(w2260) -> ("UI Config.DAQ.cfg.Sampling.sample mode"=w2257:i32)
            n1048 = Bundle By Name(cluster=T42 {"SampleMode"=10123} ("setSampleMode"), "SampleMode"=w2257) -> (w2256:T42)
            n1049 = Bundle By Name(cluster=w2260, "Message.Command"=Lockin.Commands.Local--Enum."setSamplingMode" ("Enum"), "Message.Data"=w2256) -> (w2261:T65)
            n1050 = call <vilib>:"Add State(s) to Queue__jki_lib_state_machine.vi"("State(s) in (\"\")"=w2265) -> ("States Out"=w2264:string)  [unwired: 14 in]
          }
          frame "Action: Sampling Fs Mode" {
            n1051 = Unbundle By Name(w2270) -> ("UI Config.DAQ.cfg.Sampling.Fs Mode"=w2267:T15)
            n1052 = Bundle By Name(cluster=T44 {"FsMode"=enum."Manual"} ("setSampleFsMode"), "FsMode"=w2267) -> (w2266:T44)
            n1053 = Bundle By Name(cluster=w2270, "Message.Command"=Lockin.Commands--Enum."setSamplingFsMode" ("Commands"), "Message.Data"=w2266) -> (w2271:T65)
            n1054 = call <vilib>:"Add State(s) to Queue__jki_lib_state_machine.vi"("State(s) in (\"\")"=w2275) -> ("States Out"=w2274:string)  [unwired: 14 in]
          }
          frame "Action: Sampling Fs Multiplier" {
            n1055 = Unbundle By Name(w2278) -> ("UI Config.DAQ.cfg.Sampling.Fs Multiplier"=w2277:dbl)
            n1056 = Bundle By Name(cluster=w2278, "Message.Command"=Lockin.Commands.Local--Enum."setSamplingFsMultiplier" ("Locking.Commands.Local"), "Message.Data"=w2277) -> (w2279:T65)
            n1057 = call <vilib>:"Add State(s) to Queue__jki_lib_state_machine.vi"("State(s) in (\"\")"=w2283) -> ("States Out"=w2282:string)  [unwired: 14 in]
          }
          frame "Action: Sampling Fs Output" {
            n1058 = Unbundle By Name(w2292) -> ("UI Config.Channels.Cfg_REF"=w2290:T2, "UI Config.DAQ.cfg.Sampling.Sampling"=w2289:T49)
            n1059 = call "Calculate Output Sampling.vi"("sampling info"=w2289, "Cfg_REF"=w2290) -> ("Filter Parameters"=w2288:T68)  [unwired: 8 in, 1 out]
            n1060 = Unbundle By Name(w2288) -> ("Fs.Output (S/s)"=w2284:dbl, "Settling Time (s)"=→"Settling Time (s)":dbl, "Noise Bandwidth (Hz)"=→"Noise BW (Hz)":dbl, "-3dB Bandwidth (Hz)"=→"-3dB BW (Hz)":dbl)
            "Fs Output (S/s)" <- w2284
            n1061 = Bundle By Name(cluster=w2292, "Message.Command"=Lockin.Commands.Local--Enum."setSamplingFsOutput" ("Locking.Commands.Local"), "Message.Data"=w2284, "UI Config.DAQ.cfg.Sampling.Fs.Output"=w2284) -> (w2293:T65)
            n1062 = call <vilib>:"Add State(s) to Queue__jki_lib_state_machine.vi"("State(s) in (\"\")"=w2297) -> ("States Out"=w2296:string)  [unwired: 14 in]
          }
          frame "Action: Sampling Refresh Rate" {
            n1063 = Unbundle By Name(w2300) -> ("UI Config.DAQ.cfg.Sampling.Refresh Rate (Hz)"=w2299:dbl)
            n1064 = Bundle By Name(cluster=w2300, "Message.Command"=Lockin.Commands.Local--Enum."setSamplingRefreshRate" ("Locking.Commands.Local"), "Message.Data"=w2299) -> (w2301:T65)
            n1065 = call <vilib>:"Add State(s) to Queue__jki_lib_state_machine.vi"("State(s) in (\"\")"=w2305) -> ("States Out"=w2304:string)  [unwired: 14 in]
          }
          frame "Action: Sampling Decimation Pre DSP" {
            n1066 = Unbundle By Name(w2308) -> ("UI Config.DAQ.cfg.Sampling.Decimation.PreDSP"=w2307:i32)
            n1067 = Bundle By Name(cluster=w2308, "Message.Command"=Lockin.Commands.Local--Enum."setSamplingDecimationPreDSP" ("Locking.Commands.Local"), "Message.Data"=w2307) -> (w2309:T65)
            n1068 = call <vilib>:"Add State(s) to Queue__jki_lib_state_machine.vi"("State(s) in (\"\")"=w2313) -> ("States Out"=w2312:string)  [unwired: 14 in]
          }
          frame "Action: Sampling Decimation Post DSP" {
            n1069 = Unbundle By Name(w2316) -> ("UI Config.DAQ.cfg.Sampling.Decimation.PostDSP"=w2315:i32)
            n1070 = Bundle By Name(cluster=w2316, "Message.Command"=Lockin.Commands.Local--Enum."setSamplingDecimationPostDSP" ("Locking.Commands.Local"), "Message.Data"=w2315) -> (w2317:T65)
            n1071 = call <vilib>:"Add State(s) to Queue__jki_lib_state_machine.vi"("State(s) in (\"\")"=w2321) -> ("States Out"=w2320:string)  [unwired: 14 in]
          }
          frame "Action: AI Simulate Mode" {
            n1072 = Unbundle By Name(w2324) -> ("UI Config.DAQ.Simulation mode"=w2323:T16)
            n1073 = Bundle By Name(cluster=w2324, "Message.Command"=Lockin.Commands.Local--Enum."setSimulationMode" ("Locking.Commands.Local"), "Message.Data"=w2323) -> (w2325:T65)
            n1074 = call <vilib>:"Add State(s) to Queue__jki_lib_state_machine.vi"("State(s) in (\"\")"=w2329) -> ("States Out"=w2328:string)  [unwired: 14 in]
          }
          frame "Action: Limit Amplitude" {
            n1075 = Unbundle By Name(w2332) -> ("UI Config.Limit Amplitude"=w2331:T52)
            n1076 = Bundle By Name(cluster=w2332, "Message.Command"=Lockin.Commands.Local--Enum."setAmplitudeLimit" ("Locking.Commands.Local"), "Message.Data"=w2331) -> (w2333:T65)
            n1077 = call <vilib>:"Add State(s) to Queue__jki_lib_state_machine.vi"("State(s) in (\"\")"=w2337) -> ("States Out"=w2336:string)  [unwired: 14 in]
          }
          frame "Action: Limit DC" {
            n1078 = Unbundle By Name(w2340) -> ("UI Config.Limit DC"=w2339:T53)
            n1079 = Bundle By Name(cluster=w2340, "Message.Command"=Lockin.Commands.Local--Enum."setDCLimit" ("Locking.Commands.Local"), "Message.Data"=w2339) -> (w2341:T65)
            n1080 = call <vilib>:"Add State(s) to Queue__jki_lib_state_machine.vi"("State(s) in (\"\")"=w2345) -> ("States Out"=w2344:string)  [unwired: 14 in]
          }
          frame "Action: Link Frequencies" {
            n1081 = Unbundle By Name(w2348) -> ("UI Config.Link Frequencies"=w2347:T54)
            n1082 = Bundle By Name(cluster=w2348, "Message.Command"=Lockin.Commands.Local--Enum."setFrequencyLink" ("Locking.Commands.Local"), "Message.Data"=w2347) -> (w2349:T65)
            n1083 = call <vilib>:"Add State(s) to Queue__jki_lib_state_machine.vi"("State(s) in (\"\")"=w2353) -> ("States Out"=w2352:string)  [unwired: 14 in]
          }
          frame "Action: Duty Cycle" {
            n1084 = Unbundle By Name(w2356) -> ("UI Config.Function Option"=w2355:T56)
            n1085 = Bundle By Name(cluster=w2356, "Message.Command"=Lockin.Commands.Local--Enum."setDutyCycle" ("Locking.Commands.Local"), "Message.Data"=w2355) -> (w2357:T65)
            n1086 = call <vilib>:"Add State(s) to Queue__jki_lib_state_machine.vi"("State(s) in (\"\")"=w2361) -> ("States Out"=w2360:string)  [unwired: 14 in]
          }
          frame "Action: PreFilter" {
            n1087 = Unbundle By Name(w2364) -> ("UI Config.PreFilter"=w2363:T50)
            n1088 = Bundle By Name(cluster=w2364, "Message.Command"=Lockin.Commands.Local--Enum."setPreFilter" ("Locking.Commands.Local"), "Message.Data"=w2363) -> (w2365:T65)
            n1089 = call <vilib>:"Add State(s) to Queue__jki_lib_state_machine.vi"("State(s) in (\"\")"=w2369) -> ("States Out"=w2368:string)  [unwired: 14 in]
          }
          frame "Action: Input Gain" {
            n1090 = Unbundle By Name(w2373) -> ("UI Config.Amplifers.Gain_AI"=w2371:T17)
            n1091 = for {
              tunnel: w2371 -> [w2380] mode=indexing
              tunnel: [w2379] -> w2370 mode=indexing
              n1092 = Unbundle By Name(w2380) -> ("Gain"=w2379:dbl)
            }
            n1093 = Bundle By Name(cluster=w2373, "Message.Command"=Lockin.Commands--Enum."setInputGain" ("Locking.Commands"), "Message.Data"=w2370) -> (w2374:T65)
            n1094 = call <vilib>:"Add State(s) to Queue__jki_lib_state_machine.vi"("State(s) in (\"\")"=w2378) -> ("States Out"=w2377:string)  [unwired: 14 in]
          }
          frame "Action: Output Gain" {
            n1095 = Unbundle By Name(w2384) -> ("UI Config.Amplifers.Gain_AO"=w2382:T17)
            n1096 = for {
              tunnel: w2382 -> [w2391] mode=indexing
              tunnel: [w2390] -> w2381 mode=indexing
              n1097 = Unbundle By Name(w2391) -> ("Gain"=w2390:dbl)
            }
            n1098 = Bundle By Name(cluster=w2384, "Message.Command"=Lockin.Commands--Enum."setOutputGain" ("Locking.Commands"), "Message.Data"=w2381) -> (w2385:T65)
            n1099 = call <vilib>:"Add State(s) to Queue__jki_lib_state_machine.vi"("State(s) in (\"\")"=w2389) -> ("States Out"=w2388:string)  [unwired: 14 in]
          }
          frame "Action: Offset" {
            n1100 = Unbundle By Name(w2393) -> ("UI Config.Amplifers.Offset_AI"=w2394:T17)
            n1101 = for {
              tunnel: w2394 -> [w2402] mode=indexing
              tunnel: [w2401] -> w2392 mode=indexing
              n1102 = Unbundle By Name(w2402) -> ("Gain"=w2401:dbl)
            }
            n1103 = Bundle By Name(cluster=w2393, "Message.Command"=Lockin.Commands.Local--Enum."setOffset" ("Locking.Commands.Local"), "Message.Data"=w2392) -> (w2396:T65)
            n1104 = call <vilib>:"Add State(s) to Queue__jki_lib_state_machine.vi"("State(s) in (\"\")"=w2400) -> ("States Out"=w2399:string)  [unwired: 14 in]
          }
          frame "Action: Offset Mode" {
            n1105 = Scan From String(input string=w2406, default 1=Offset_Mode--Enum."Measure" ("Offset Mode")) -> (output 1=w2405:T31)  [unwired: 3 in, 3 out]
            n1106 = Build Array(w2405) -> (w2404:T31[])
            n1107 = Bundle By Name(cluster=w2408, "Message.Command"=Lockin.Commands.Local--Enum."setOffsetMode" ("Locking.Commands.Local"), "Message.Data"=w2404) -> (w2409:T65)
            n1108 = call <vilib>:"Add State(s) to Queue__jki_lib_state_machine.vi"("State(s) in (\"\")"=w2413) -> ("States Out"=w2412:string)  [unwired: 14 in]
          }
          frame "Action: Calibrate" {
            n1109 = Scan From String(input string=w2416, default 1=PrivateEvents--DAQ.setCalibration."Check" ("setCalibration")) -> (output 1=w2415:T32)  [unwired: 3 in, 3 out]
            n1110 = Bundle By Name(cluster=w2418, "Message.Command"=Lockin.Commands.Local--Enum."setCalibration" ("Locking.Commands.Local"), "Message.Data"=w2415) -> (w2419:T65)
            n1111 = call <vilib>:"Add State(s) to Queue__jki_lib_state_machine.vi"("State(s) in (\"\")"=w2423) -> ("States Out"=w2422:string)  [unwired: 14 in]
          }
          frame "Action: Zero Phase" {
            n1112 = Bundle By Name(cluster=w2425, "Message.Command"=Lockin.Commands.Local--Enum."zeroPhase" ("Locking.Commands.Local")) -> (w2426:T65)
            n1113 = call <vilib>:"Add State(s) to Queue__jki_lib_state_machine.vi"("State(s) in (\"\")"=w2430) -> ("States Out"=w2429:string)  [unwired: 14 in]
          }
          frame "Action: Power Spectrum" {
            n1114 = Unbundle By Name(w2454) -> ("getAll.Waveforms.AO"=w2443:waveform(dbl)[], "getAll.Waveforms.AI"=w2439:waveform(dbl)[], "Waveform Charts"=w2436:waveform(dbl)[][])
            n1115 = call "Is Value Changed.vim"("value"="PS Display") -> ("changed or first call?"=w2442:bool)
            n1116 = case shown="\"AI\"" "PS Display" {
              tunnel: w2443 -> [w2467 _ _ _ _ _]
              tunnel: [w2467 w2468 w2469 w2473 w2476 w2479] -> w2440
              tunnel: w2439 -> [_ w2468 _ _ _ _]
              tunnel: w2436 -> [_ _ w2470 w2474 w2477 w2480]
              frame "AO", Default {
              }
              frame "AI" {
              }
              frame "X" {
                n1117 = Index Array(array=w2470, index (row)=0) -> (element=w2469:waveform(dbl)[])  [unwired: 1 in]
              }
              frame "Y" {
                n1118 = Index Array(array=w2474, index (row)=1) -> (element=w2473:waveform(dbl)[])  [unwired: 1 in]
              }
              frame "R" {
                n1119 = Index Array(array=w2477, index (row)=2) -> (element=w2476:waveform(dbl)[])  [unwired: 1 in]
              }
              frame "Theta" {
                n1120 = Index Array(array=w2480, index (row)=3) -> (element=w2479:waveform(dbl)[])  [unwired: 1 in]
              }
            }
            n1121 = Bundle By Name(cluster=T45 {"averaging mode"=enum."No averaging", "weighting mode"=enum."Exponential", "number of averages"=10} ("averaging parameters"), "averaging mode"="averaging mode", "weighting mode"="weighting mode", "number of averages"="# averages") -> (w2447:T45)
            n1122 = Or(x="restart", y=w2442) -> (x .or. y?=w2431:bool)
            n1123 = call-poly <vilib>:"FFT Power Spectrum and PSD.vi"("export mode"="export mode", "averaging parameters"=w2447, "restart averaging (F)"=w2431, "error in (no error)"=w2453, "dB On (F)"=TRUE, "window"="window", "time signals"=w2440) -> ("error out"=w2434:errorcluster, "averages completed"=→"averages":dbl, "averaging done"=→"done?":bool, "Power Spectrum / PSD"=w2435:cluster{"f0":dbl, "df":dbl, "magnitude":dbl[]}[])  [unwired: 1 in]
            "PS Waveform" <- w2435
            n1124 = case shown="True" w2431 {
              frame False {
              }
              frame True {
                w2458 = u8 1 ("X Scale.Scale Fit")
                n1125 = property on="PS Waveform" class="WFGraph (strict)"("XScale.ScaleFit"=w2458, "YScale.ScaleFit"=w2458) -> ()  [unwired: 2 in, 2 out]
              }
            }
            n1126 = case shown="True" "chart?" {
              tunnel: w2435 -> [_ w2466]
              tunnel: w2434 -> [w2460 w2465]
              tunnel: [w2460 w2464] -> w2433
              frame False {
                n1127 = local write "PS Chart"(dbl[][] [] ("Waveform Chart")) -> ()
              }
              frame True {
                n1128 = control-ref of="PS Waveform"() -> (w2463:refnum<vi>)
                n1129 = call "PS Chart.vi"("all?"="chart all?", "error in (no error)"=w2465, "Power Spectrum / PSD"=w2466, "WFGraph (WDT) in"=w2463) -> ("error out"=w2464:errorcluster, "Chart"=→"PS Chart":dbl[][])  [unwired: 6 in]
              }
            }
            n1130 = call <vilib>:"Add State(s) to Queue__jki_lib_state_machine.vi"("State(s) in (\"\")"=w2457) -> ("States Out"=w2456:string)  [unwired: 14 in]
          }
          frame "Action: Route" {
            n1131 = Unbundle By Name(w2481) -> ("SMO"=w2483:refnum<class "Instrument UI.Lockin.lvclass">)
            n1132 = Bundle By Name(cluster=w2481, "SMO"=w2483) -> (w2482:T65)
            n1133 = call <vilib>:"Add State(s) to Queue__jki_lib_state_machine.vi"("State(s) in (\"\")"=w2487) -> ("States Out"=w2486:string)  [unwired: 14 in]
          }
          frame "Action: PLL" {
            n1134 = Unbundle By Name(w2488) -> ("SMO"=w2490:refnum<class "Instrument UI.Lockin.lvclass">)
            n1135 = Bundle By Name(cluster=w2488, "SMO"=w2490) -> (w2489:T65)
            n1136 = call <vilib>:"Add State(s) to Queue__jki_lib_state_machine.vi"("State(s) in (\"\")"=w2494) -> ("States Out"=w2493:string)  [unwired: 14 in]
          }
        }
      }
    }
    frame Error {
    }
  }
  n1137 = call-parent "Process.vi"("error in"=w5, "Instrument UI in"=w4) -> ("error out"=w2:errorcluster, "Instrument UI out"=→"Lockin.UI out":refnum<class "Instrument UI.Lockin.lvclass">)  [unwired: 8 in]
  n1138 = Merge Errors(w2, w1) -> (→"error out":errorcluster)
